vi "Thermal_Camera_Evaluation.vi"() -> (11 "placeholder image":T1(plugin-control))   [LabVIEW 2020]
uses:
  <vilib>/vision/Image Controls.llb/IMAQ Image.ctl
  DataCluster_TCAL.ctl
  <vilib>/Utility/file.llb/Write Delimited Spreadsheet (string).vi
  <vilib>/Utility/file.llb/Read Delimited Spreadsheet (string).vi
  <vilib>/Analysis/NI_AALBase.lvlib
panel:
  in  "Correct Data":bool
  out "Offset Applied?":bool=TRUE
  out "recentPaths":path[](array[path])=[path "C:/Users/au540322/Documents/Projects/Ice-Nucleation/Data/D20_4/Result Data.csv", path "C:/Users/au540322/Documents/Projects/Ice-Nucleation/Data/System Test_9/Result Data.csv"]
  out "version":string="version 0.0.0.1" caption="Version"
  out "Title":string="Thermal Camera Evaluation" caption="Version"
  in  "Remove_Correction":bool
  out "Offsets":dbl[](array[numeric])
  in  "Calc_All":bool
  in  "Well":i32=94
  in  "ImageIdx":u32(slide)=74 scale=0.0..527.0
  in  "Path":path=path "C:/Users/au540322/Documents/Projects/Ice-Nucleation/Data/D20_4"
  out "FreezeArray":bool[](array[boolean])=[TRUE, TRUE, TRUE, TRUE, TRUE, TRUE, TRUE, TRUE, TRUE, TRUE, TRUE, TRUE, TRUE, TRUE, TRUE, TRUE, TRUE, TRUE, FALSE, TRUE, TRUE, TRUE, TRUE, TRUE, TRUE, TRUE, TRUE, TRUE, TRUE, TRUE, TRUE, TRUE, TRUE, TRUE, TRUE, TRUE, TRUE, TRUE, TRUE, TRUE, TRUE, TRUE, FALSE, TRUE, TRUE, TRUE, TRUE, TRUE, TRUE, TRUE, TRUE, TRUE, TRUE, TRUE, TRUE, TRUE, TRUE, TRUE, TRUE, TRUE, TRUE, TRUE, TRUE, TRUE, TRUE, TRUE, FALSE, TRUE, TRUE, FALSE, TRUE, TRUE, TRUE, TRUE, TRUE, TRUE, TRUE, TRUE, TRUE, TRUE, TRUE, TRUE, TRUE, TRUE, TRUE, TRUE, TRUE, TRUE, TRUE, TRUE, TRUE, TRUE, TRUE, TRUE, TRUE, TRUE, TRUE, TRUE, TRUE, TRUE, TRUE, TRUE, TRUE, TRUE, TRUE, TRUE, TRUE, TRUE, TRUE, TRUE, TRUE, TRUE, TRUE, TRUE, TRUE, TRUE, TRUE, TRUE, TRUE, TRUE, TRUE, TRUE, TRUE, TRUE, TRUE, TRUE, TRUE, TRUE, TRUE, TRUE, TRUE, TRUE, TRUE, TRUE, TRUE, TRUE, TRUE, TRUE, TRUE, TRUE, TRUE, TRUE, TRUE, TRUE, TRUE, TRUE, TRUE, TRUE, TRUE, TRUE, TRUE, TRUE, TRUE, TRUE, TRUE, TRUE, TRUE, TRUE, TRUE, TRUE, TRUE, TRUE, TRUE, TRUE, TRUE, TRUE, TRUE, TRUE, TRUE, TRUE, TRUE, TRUE, TRUE, TRUE, TRUE, TRUE, TRUE, TRUE, TRUE, TRUE, TRUE, TRUE, TRUE, TRUE, TRUE, TRUE, TRUE, TRUE, TRUE, TRUE, TRUE, TRUE, TRUE, TRUE, TRUE, TRUE, TRUE, TRUE, TRUE, TRUE, TRUE, TRUE, TRUE, TRUE, TRUE, TRUE, TRUE, TRUE, TRUE, TRUE, FALSE, TRUE, TRUE, TRUE, TRUE, TRUE, TRUE, TRUE, TRUE, TRUE, TRUE, TRUE, TRUE, TRUE, TRUE, TRUE, TRUE, TRUE, TRUE, TRUE, TRUE, TRUE, TRUE, TRUE, FALSE, TRUE, TRUE, TRUE, TRUE, TRUE, TRUE, TRUE, TRUE, TRUE, TRUE, TRUE, TRUE, TRUE, TRUE, TRUE, TRUE, TRUE, TRUE, TRUE, TRUE, TRUE, TRUE, TRUE, FALSE, TRUE, TRUE, TRUE, TRUE, TRUE, TRUE, TRUE, TRUE, TRUE, TRUE, TRUE, TRUE, TRUE, TRUE, TRUE, TRUE, TRUE, TRUE, TRUE, TRUE, TRUE, TRUE, TRUE, TRUE, TRUE, TRUE, TRUE, TRUE, TRUE, TRUE, TRUE, TRUE, TRUE, TRUE, TRUE, TRUE, TRUE, TRUE, TRUE, TRUE, TRUE, TRUE, TRUE, TRUE, TRUE, TRUE, TRUE, TRUE, TRUE, TRUE, TRUE, TRUE, TRUE, TRUE, TRUE, TRUE, TRUE, TRUE, TRUE, TRUE, TRUE, TRUE, TRUE, TRUE, TRUE, TRUE, TRUE, TRUE, TRUE, TRUE, TRUE, TRUE, TRUE, TRUE, TRUE, TRUE, TRUE, TRUE, TRUE, TRUE, TRUE, TRUE, TRUE, TRUE, TRUE, TRUE, TRUE, TRUE, TRUE, TRUE, TRUE, TRUE, TRUE, TRUE, TRUE, TRUE, TRUE, TRUE, TRUE, TRUE, TRUE, TRUE, TRUE, TRUE, TRUE, TRUE, TRUE, TRUE, TRUE, TRUE, TRUE, TRUE, TRUE, TRUE, TRUE, TRUE, TRUE, TRUE, TRUE, TRUE, TRUE, TRUE, TRUE, TRUE, TRUE]
  out "ThermTemps":dbl[](array[numeric])=[7.37336, 7.350183, 7.292026, 7.209824, 7.126844, 7.047335, 6.967812, 6.887927, 6.807507, 6.726127, 6.647346, 6.566629, 6.484972, 6.403476, 6.320742, 6.240016, 6.159057, 6.077253, 5.994363, 5.911582, 5.834026, 5.750156, 5.668103, 5.585564, 5.503295, 5.421148, 5.337707, 5.255535, 5.176404, 5.097319, 5.014855, 4.933567, 4.8527, 4.772503, 4.690195, 4.609957, 4.530865, 4.450195, 4.368275, 4.287447, 4.20743, 4.128069, 4.046262, 3.966046, 3.884444, 3.804914, 3.72549, 3.644432, 3.56432, 3.482743, 3.402111, 3.320773, 3.241597, 3.160814, 3.078633, 2.999147, 2.916221, 2.834318, 2.753718, 2.671023, 2.590394, 2.507449, 2.425426, 2.345006, 2.263807, 2.180767, 2.098148, 2.01567, 1.933412, 1.852712, 1.770749, 1.688175, 1.60685, 1.526749, 1.447674, 1.3716, 1.297226, 1.221186, 1.146355, 1.070605, 0.992937, 0.915288, 0.838683, 0.762464, 0.679874, 0.600579, 0.51705, 0.434996, 0.356589, 0.277921, 0.196637, 0.111731, 0.026607, -0.060313, -0.14656, -0.233002, -0.318977, -0.403944, -0.487975, -0.568988, -0.651118, -0.726572, -0.802282, -0.877375, -0.955081, -1.032134, -1.111683, -1.190094, -1.270206, -1.349321, -1.429882, -1.51019, -1.594696, -1.675437, -1.76021, -1.842875, -1.926273, -2.011868, -2.097424, -2.180477, -2.265338, -2.350737, -2.434776, -2.520055, -2.603456, -2.685369, -2.767054, -2.849678, -2.928727, -3.007247, -3.085221, -3.160799, -3.237649, -3.314684, -3.391643, -3.468468, -3.546785, -3.624741, -3.70393, -3.783419, -3.864142, -3.943202, -4.022923, -4.103283, -4.185443, -4.267742, -4.351195, -4.432318, -4.516093, -4.599727, -4.682185, -4.766104, -4.850224, -4.93466, -5.017512, -5.101476, -5.183878, -5.266203, -5.3476, -5.430232, -5.512818, -5.595638, -5.678559, -5.759164, -5.842224, -5.925119, -6.00861, -6.087647, -6.169719, -6.250624, -6.332033, -6.41154, -6.493741, -6.574607, -6.65432, -6.735998, -6.81658, -6.884113, -6.971353, -7.058345, -7.13845, -7.217778, -7.29712, -7.376817, -7.457704, -7.536944, -7.618041, -7.696611, -7.776192, -7.856406, -7.936625, -8.015928, -8.096638, -8.176965, -8.256535, -8.333434, -8.412476, -8.491866, -8.572104, -8.653451, -8.736341, -8.818344, -8.9003, -8.979957, -9.063351, -9.144428, -9.225466, -9.308084, -9.389312, -9.471749, -9.55375, -9.635666, -9.719444, -9.801393, -9.883319, -9.965156, -10.046111, -10.126569, -10.206901, -10.288882, -10.367175, -10.44764, -10.528476, -10.607278, -10.686439, -10.76692, -10.846853, -10.925344, -11.005718, -11.085251, -11.164821, -11.243882, -11.32307, -11.402453, -11.482498, -11.561041, -11.641285, -11.721693, -11.802165, -11.881356, -11.960557, -12.038971, -12.117215, -12.198103, -12.277232, -12.357776, -12.438832, -12.518799, -12.601298, -12.682659, -12.764128, -12.845615, -12.926062, -13.007562, -13.090462, -13.172514, -13.253457, -13.335363, -13.415947, -13.500095, -13.581218, -13.662798, -13.745541, -13.827711, -13.909167, -13.988528, -14.067897, -14.146499, -14.22637, -14.306951, -14.385678, -14.465256, -14.545529, -14.624618, -14.703428, -14.780312, -14.860595, -14.938995, -15.018888, -15.099258, -15.177778, -15.257835, -15.336496, -15.415752, -15.494147, -15.573314, -15.652589, -15.731922, -15.809635, -15.888123, -15.96994, -16.049542, -16.129671, -16.210636, -16.291627, -16.372217, -16.453213, -16.533459, -16.614772, -16.697373, -16.777753, -16.859325, -16.941111, -17.021954, -17.104644, -17.18694, -17.265191, -17.34818, -17.429989, -17.511056, -17.592864, -17.672998, -17.752001, -17.832689, -17.912607, -17.991497, -18.072515, -18.152648, -18.231922, -18.310442, -18.39034, -18.469296, -18.547367, -18.625873, -18.703345, -18.784246, -18.861563, -18.939331, -19.016652, -19.094699, -19.172515, -19.250605, -19.329034, -19.40733, -19.486762, -19.565877, -19.648403, -19.726327, -19.808446, -19.888915, -19.969109, -20.049822, -20.129964, -20.210119, -20.290948, -20.37219, -20.454346, -20.533518, -20.615081, -20.69688, -20.779181, -20.859909, -20.940508, -21.021895, -21.10374, -21.185525, -21.268245, -21.348339, -21.425612, -21.505022, -21.583855, -21.662198, -21.739967, -21.818083, -21.894826, -21.972925, -22.050531, -22.127525, -22.204371, -22.282005, -22.35634, -22.434321, -22.511412, -22.589688, -22.667553, -22.744158, -22.822019, -22.89791, -22.975844, -23.05133, -23.130531, -23.211038, -23.290909, -23.370573, -23.45021, -23.530535, -23.609552, -23.687938, -23.768015, -23.847606, -23.927972, -24.010068, -24.089525, -24.16956, -24.249907, -24.330105, -24.40904, -24.488729, -24.569942, -24.649037, -24.729342, -24.80955, -24.888373, -24.967519, -25.047611, -25.125437, -25.204448, -25.282442, -25.360463, -25.437591, -25.514136, -25.593629, -25.668979, -25.743502, -25.820043, -25.89306, -25.97015, -26.045113, -26.118008, -26.194843, -26.268271, -26.342508, -26.416119, -26.490791, -26.566611, -26.642888, -26.719932, -26.797288, -26.874969, -26.951676, -27.028748, -27.104065, -27.181792, -27.258419, -27.33566, -27.413455, -27.493028, -27.56923, -27.646282, -27.721342, -27.798636, -27.878491, -27.956447, -28.033548, -28.109932, -28.186744, -28.262818, -28.340363, -28.41596, -28.491609, -28.56755, -28.642851, -28.720287, -28.794581, -28.868607, -28.943815, -29.019102, -29.093409, -29.168045, -29.242483, -29.315565, -29.390267, -29.463635, -29.540833, -29.613751, -29.686, -29.757983, -29.830992, -29.902322, -29.975634, -30.043051, -30.107764, -30.175561, -30.243789, -30.314343, -30.381896, -30.449693, -30.507812, -30.566745, -30.623567, -30.680952, -30.734143, -30.787765, -30.83898, -30.888996, -30.939253, -30.987606, -31.032869, -31.08053, -31.125474, -31.170159, -31.214239, -31.2553, -31.297168, -31.338367, -31.377898, -31.416899, -31.456416, -31.492706, -31.528817, -31.56739, -31.602582, -31.637368, -31.673019, -31.704931, -31.738656, -31.77053, -31.801731, -31.832112, -31.862399, -31.888523, -31.920833, -31.946986, -31.97368, -32.001595, -32.026341, -32.054092, -32.079652, -32.104587, -32.128267, -32.154891, -32.176728, -32.198059, -32.21954, -32.242051, -32.264665, -32.28386, -32.306436]
  out "PartitionArray":string[](array[string])=["A, MQ unfiltered", "A, MQ unfiltered", "A, MQ unfiltered", "B, D2O unfiltered", "B, D2O unfiltered", "B, D2O unfiltered", "C, 1mg/ml Snomax in MQ", "C, 1mg/ml Snomax in MQ", "C, 1mg/ml Snomax in MQ", "C, 1mg/ml Snomax in MQ", "C, 1mg/ml Snomax in MQ", "C, 1mg/ml Snomax in MQ", "D, 1mg/ml Snomax in 1:1 MQ:D2O", "D, 1mg/ml Snomax in 1:1 MQ:D2O", "D, 1mg/ml Snomax in 1:1 MQ:D2O", "D, 1mg/ml Snomax in 1:1 MQ:D2O", "D, 1mg/ml Snomax in 1:1 MQ:D2O", "D, 1mg/ml Snomax in 1:1 MQ:D2O", "E, 1mg/ml Snomax in D2O", "E, 1mg/ml Snomax in D2O", "E, 1mg/ml Snomax in D2O", "E, 1mg/ml Snomax in D2O", "E, 1mg/ml Snomax in D2O", "E, 1mg/ml Snomax in D2O", "A, MQ unfiltered", "A, MQ unfiltered", "A, MQ unfiltered", "B, D2O unfiltered", "B, D2O unfiltered", "B, D2O unfiltered", "C, 1mg/ml Snomax in MQ", "C, 1mg/ml Snomax in MQ", "C, 1mg/ml Snomax in MQ", "C, 1mg/ml Snomax in MQ", "C, 1mg/ml Snomax in MQ", "C, 1mg/ml Snomax in MQ", "D, 1mg/ml Snomax in 1:1 MQ:D2O", "D, 1mg/ml Snomax in 1:1 MQ:D2O", "D, 1mg/ml Snomax in 1:1 MQ:D2O", "D, 1mg/ml Snomax in 1:1 MQ:D2O", "D, 1mg/ml Snomax in 1:1 MQ:D2O", "D, 1mg/ml Snomax in 1:1 MQ:D2O", "E, 1mg/ml Snomax in D2O", "E, 1mg/ml Snomax in D2O", "E, 1mg/ml Snomax in D2O", "E, 1mg/ml Snomax in D2O", "E, 1mg/ml Snomax in D2O", "E, 1mg/ml Snomax in D2O", "A, MQ unfiltered", "A, MQ unfiltered", "A, MQ unfiltered", "B, D2O unfiltered", "B, D2O unfiltered", "B, D2O unfiltered", "C, 1mg/ml Snomax in MQ", "C, 1mg/ml Snomax in MQ", "C, 1mg/ml Snomax in MQ", "C, 1mg/ml Snomax in MQ", "C, 1mg/ml Snomax in MQ", "C, 1mg/ml Snomax in MQ", "D, 1mg/ml Snomax in 1:1 MQ:D2O", "D, 1mg/ml Snomax in 1:1 MQ:D2O", "D, 1mg/ml Snomax in 1:1 MQ:D2O", "D, 1mg/ml Snomax in 1:1 MQ:D2O", "D, 1mg/ml Snomax in 1:1 MQ:D2O", "D, 1mg/ml Snomax in 1:1 MQ:D2O", "E, 1mg/ml Snomax in D2O", "E, 1mg/ml Snomax in D2O", "E, 1mg/ml Snomax in D2O", "E, 1mg/ml Snomax in D2O", "E, 1mg/ml Snomax in D2O", "E, 1mg/ml Snomax in D2O", "A, MQ unfiltered", "A, MQ unfiltered", "A, MQ unfiltered", "B, D2O unfiltered", "B, D2O unfiltered", "B, D2O unfiltered", "C, 1mg/ml Snomax in MQ", "C, 1mg/ml Snomax in MQ", "C, 1mg/ml Snomax in MQ", "C, 1mg/ml Snomax in MQ", "C, 1mg/ml Snomax in MQ", "C, 1mg/ml Snomax in MQ", "D, 1mg/ml Snomax in 1:1 MQ:D2O", "D, 1mg/ml Snomax in 1:1 MQ:D2O", "D, 1mg/ml Snomax in 1:1 MQ:D2O", "D, 1mg/ml Snomax in 1:1 MQ:D2O", "D, 1mg/ml Snomax in 1:1 MQ:D2O", "D, 1mg/ml Snomax in 1:1 MQ:D2O", "E, 1mg/ml Snomax in D2O", "E, 1mg/ml Snomax in D2O", "E, 1mg/ml Snomax in D2O", "E, 1mg/ml Snomax in D2O", "E, 1mg/ml Snomax in D2O", "E, 1mg/ml Snomax in D2O", "A, MQ unfiltered", "A, MQ unfiltered", "A, MQ unfiltered", "B, D2O unfiltered", "B, D2O unfiltered", "B, D2O unfiltered", "C, 1mg/ml Snomax in MQ", "C, 1mg/ml Snomax in MQ", "C, 1mg/ml Snomax in MQ", "C, 1mg/ml Snomax in MQ", "C, 1mg/ml Snomax in MQ", "C, 1mg/ml Snomax in MQ", "D, 1mg/ml Snomax in 1:1 MQ:D2O", "D, 1mg/ml Snomax in 1:1 MQ:D2O", "D, 1mg/ml Snomax in 1:1 MQ:D2O", "D, 1mg/ml Snomax in 1:1 MQ:D2O", "D, 1mg/ml Snomax in 1:1 MQ:D2O", "D, 1mg/ml Snomax in 1:1 MQ:D2O", "E, 1mg/ml Snomax in D2O", "E, 1mg/ml Snomax in D2O", "E, 1mg/ml Snomax in D2O", "E, 1mg/ml Snomax in D2O", "E, 1mg/ml Snomax in D2O", "E, 1mg/ml Snomax in D2O", "A, MQ unfiltered", "A, MQ unfiltered", "A, MQ unfiltered", "B, D2O unfiltered", "B, D2O unfiltered", "B, D2O unfiltered", "C, 1mg/ml Snomax in MQ", "C, 1mg/ml Snomax in MQ", "C, 1mg/ml Snomax in MQ", "C, 1mg/ml Snomax in MQ", "C, 1mg/ml Snomax in MQ", "C, 1mg/ml Snomax in MQ", "D, 1mg/ml Snomax in 1:1 MQ:D2O", "D, 1mg/ml Snomax in 1:1 MQ:D2O", "D, 1mg/ml Snomax in 1:1 MQ:D2O", "D, 1mg/ml Snomax in 1:1 MQ:D2O", "D, 1mg/ml Snomax in 1:1 MQ:D2O", "D, 1mg/ml Snomax in 1:1 MQ:D2O", "E, 1mg/ml Snomax in D2O", "E, 1mg/ml Snomax in D2O", "E, 1mg/ml Snomax in D2O", "E, 1mg/ml Snomax in D2O", "E, 1mg/ml Snomax in D2O", "E, 1mg/ml Snomax in D2O", "A, MQ unfiltered", "A, MQ unfiltered", "A, MQ unfiltered", "B, D2O unfiltered", "B, D2O unfiltered", "B, D2O unfiltered", "C, 1mg/ml Snomax in MQ", "C, 1mg/ml Snomax in MQ", "C, 1mg/ml Snomax in MQ", "C, 1mg/ml Snomax in MQ", "C, 1mg/ml Snomax in MQ", "C, 1mg/ml Snomax in MQ", "D, 1mg/ml Snomax in 1:1 MQ:D2O", "D, 1mg/ml Snomax in 1:1 MQ:D2O", "D, 1mg/ml Snomax in 1:1 MQ:D2O", "D, 1mg/ml Snomax in 1:1 MQ:D2O", "D, 1mg/ml Snomax in 1:1 MQ:D2O", "D, 1mg/ml Snomax in 1:1 MQ:D2O", "E, 1mg/ml Snomax in D2O", "E, 1mg/ml Snomax in D2O", "E, 1mg/ml Snomax in D2O", "E, 1mg/ml Snomax in D2O", "E, 1mg/ml Snomax in D2O", "E, 1mg/ml Snomax in D2O", "A, MQ unfiltered", "A, MQ unfiltered", "A, MQ unfiltered", "B, D2O unfiltered", "B, D2O unfiltered", "B, D2O unfiltered", "C, 1mg/ml Snomax in MQ", "C, 1mg/ml Snomax in MQ", "C, 1mg/ml Snomax in MQ", "C, 1mg/ml Snomax in MQ", "C, 1mg/ml Snomax in MQ", "C, 1mg/ml Snomax in MQ", "D, 1mg/ml Snomax in 1:1 MQ:D2O", "D, 1mg/ml Snomax in 1:1 MQ:D2O", "D, 1mg/ml Snomax in 1:1 MQ:D2O", "D, 1mg/ml Snomax in 1:1 MQ:D2O", "D, 1mg/ml Snomax in 1:1 MQ:D2O", "D, 1mg/ml Snomax in 1:1 MQ:D2O", "E, 1mg/ml Snomax in D2O", "E, 1mg/ml Snomax in D2O", "E, 1mg/ml Snomax in D2O", "E, 1mg/ml Snomax in D2O", "E, 1mg/ml Snomax in D2O", "E, 1mg/ml Snomax in D2O", "A, MQ unfiltered", "A, MQ unfiltered", "A, MQ unfiltered", "B, D2O unfiltered", "B, D2O unfiltered", "B, D2O unfiltered", "C, 1mg/ml Snomax in MQ", "C, 1mg/ml Snomax in MQ", "C, 1mg/ml Snomax in MQ", "C, 1mg/ml Snomax in MQ", "C, 1mg/ml Snomax in MQ", "C, 1mg/ml Snomax in MQ", "D, 1mg/ml Snomax in 1:1 MQ:D2O", "D, 1mg/ml Snomax in 1:1 MQ:D2O", "D, 1mg/ml Snomax in 1:1 MQ:D2O", "D, 1mg/ml Snomax in 1:1 MQ:D2O", "D, 1mg/ml Snomax in 1:1 MQ:D2O", "D, 1mg/ml Snomax in 1:1 MQ:D2O", "E, 1mg/ml Snomax in D2O", "E, 1mg/ml Snomax in D2O", "E, 1mg/ml Snomax in D2O", "E, 1mg/ml Snomax in D2O", "E, 1mg/ml Snomax in D2O", "E, 1mg/ml Snomax in D2O", "A, MQ unfiltered", "A, MQ unfiltered", "A, MQ unfiltered", "B, D2O unfiltered", "B, D2O unfiltered", "B, D2O unfiltered", "C, 1mg/ml Snomax in MQ", "C, 1mg/ml Snomax in MQ", "C, 1mg/ml Snomax in MQ", "C, 1mg/ml Snomax in MQ", "C, 1mg/ml Snomax in MQ", "C, 1mg/ml Snomax in MQ", "D, 1mg/ml Snomax in 1:1 MQ:D2O", "D, 1mg/ml Snomax in 1:1 MQ:D2O", "D, 1mg/ml Snomax in 1:1 MQ:D2O", "D, 1mg/ml Snomax in 1:1 MQ:D2O", "D, 1mg/ml Snomax in 1:1 MQ:D2O", "D, 1mg/ml Snomax in 1:1 MQ:D2O", "E, 1mg/ml Snomax in D2O", "E, 1mg/ml Snomax in D2O", "E, 1mg/ml Snomax in D2O", "E, 1mg/ml Snomax in D2O", "E, 1mg/ml Snomax in D2O", "E, 1mg/ml Snomax in D2O", "A, MQ unfiltered", "A, MQ unfiltered", "A, MQ unfiltered", "B, D2O unfiltered", "B, D2O unfiltered", "B, D2O unfiltered", "C, 1mg/ml Snomax in MQ", "C, 1mg/ml Snomax in MQ", "C, 1mg/ml Snomax in MQ", "C, 1mg/ml Snomax in MQ", "C, 1mg/ml Snomax in MQ", "C, 1mg/ml Snomax in MQ", "D, 1mg/ml Snomax in 1:1 MQ:D2O", "D, 1mg/ml Snomax in 1:1 MQ:D2O", "D, 1mg/ml Snomax in 1:1 MQ:D2O", "D, 1mg/ml Snomax in 1:1 MQ:D2O", "D, 1mg/ml Snomax in 1:1 MQ:D2O", "D, 1mg/ml Snomax in 1:1 MQ:D2O", "E, 1mg/ml Snomax in D2O", "E, 1mg/ml Snomax in D2O", "E, 1mg/ml Snomax in D2O", "E, 1mg/ml Snomax in D2O", "E, 1mg/ml Snomax in D2O", "E, 1mg/ml Snomax in D2O", "A, MQ unfiltered", "A, MQ unfiltered", "A, MQ unfiltered", "B, D2O unfiltered", "B, D2O unfiltered", "B, D2O unfiltered", "C, 1mg/ml Snomax in MQ", "C, 1mg/ml Snomax in MQ", "C, 1mg/ml Snomax in MQ", "C, 1mg/ml Snomax in MQ", "C, 1mg/ml Snomax in MQ", "C, 1mg/ml Snomax in MQ", "D, 1mg/ml Snomax in 1:1 MQ:D2O", "D, 1mg/ml Snomax in 1:1 MQ:D2O", "D, 1mg/ml Snomax in 1:1 MQ:D2O", "D, 1mg/ml Snomax in 1:1 MQ:D2O", "D, 1mg/ml Snomax in 1:1 MQ:D2O", "D, 1mg/ml Snomax in 1:1 MQ:D2O", "E, 1mg/ml Snomax in D2O", "E, 1mg/ml Snomax in D2O", "E, 1mg/ml Snomax in D2O", "E, 1mg/ml Snomax in D2O", "E, 1mg/ml Snomax in D2O", "E, 1mg/ml Snomax in D2O", "A, MQ unfiltered", "A, MQ unfiltered", "A, MQ unfiltered", "B, D2O unfiltered", "B, D2O unfiltered", "B, D2O unfiltered", "C, 1mg/ml Snomax in MQ", "C, 1mg/ml Snomax in MQ", "C, 1mg/ml Snomax in MQ", "C, 1mg/ml Snomax in MQ", "C, 1mg/ml Snomax in MQ", "C, 1mg/ml Snomax in MQ", "D, 1mg/ml Snomax in 1:1 MQ:D2O", "D, 1mg/ml Snomax in 1:1 MQ:D2O", "D, 1mg/ml Snomax in 1:1 MQ:D2O", "D, 1mg/ml Snomax in 1:1 MQ:D2O", "D, 1mg/ml Snomax in 1:1 MQ:D2O", "D, 1mg/ml Snomax in 1:1 MQ:D2O", "E, 1mg/ml Snomax in D2O", "E, 1mg/ml Snomax in D2O", "E, 1mg/ml Snomax in D2O", "E, 1mg/ml Snomax in D2O", "E, 1mg/ml Snomax in D2O", "E, 1mg/ml Snomax in D2O", "A, MQ unfiltered", "A, MQ unfiltered", "A, MQ unfiltered", "B, D2O unfiltered", "B, D2O unfiltered", "B, D2O unfiltered", "C, 1mg/ml Snomax in MQ", "C, 1mg/ml Snomax in MQ", "C, 1mg/ml Snomax in MQ", "C, 1mg/ml Snomax in MQ", "C, 1mg/ml Snomax in MQ", "C, 1mg/ml Snomax in MQ", "D, 1mg/ml Snomax in 1:1 MQ:D2O", "D, 1mg/ml Snomax in 1:1 MQ:D2O", "D, 1mg/ml Snomax in 1:1 MQ:D2O", "D, 1mg/ml Snomax in 1:1 MQ:D2O", "D, 1mg/ml Snomax in 1:1 MQ:D2O", "D, 1mg/ml Snomax in 1:1 MQ:D2O", "E, 1mg/ml Snomax in D2O", "E, 1mg/ml Snomax in D2O", "E, 1mg/ml Snomax in D2O", "E, 1mg/ml Snomax in D2O", "E, 1mg/ml Snomax in D2O", "E, 1mg/ml Snomax in D2O", "A, MQ unfiltered", "A, MQ unfiltered", "A, MQ unfiltered", "B, D2O unfiltered", "B, D2O unfiltered", "B, D2O unfiltered", "C, 1mg/ml Snomax in MQ", "C, 1mg/ml Snomax in MQ", "C, 1mg/ml Snomax in MQ", "C, 1mg/ml Snomax in MQ", "C, 1mg/ml Snomax in MQ", "C, 1mg/ml Snomax in MQ", "D, 1mg/ml Snomax in 1:1 MQ:D2O", "D, 1mg/ml Snomax in 1:1 MQ:D2O", "D, 1mg/ml Snomax in 1:1 MQ:D2O", "D, 1mg/ml Snomax in 1:1 MQ:D2O", "D, 1mg/ml Snomax in 1:1 MQ:D2O", "D, 1mg/ml Snomax in 1:1 MQ:D2O", "E, 1mg/ml Snomax in D2O", "E, 1mg/ml Snomax in D2O", "E, 1mg/ml Snomax in D2O", "E, 1mg/ml Snomax in D2O", "E, 1mg/ml Snomax in D2O", "E, 1mg/ml Snomax in D2O", "A, MQ unfiltered", "A, MQ unfiltered", "A, MQ unfiltered", "B, D2O unfiltered", "B, D2O unfiltered", "B, D2O unfiltered", "C, 1mg/ml Snomax in MQ", "C, 1mg/ml Snomax in MQ", "C, 1mg/ml Snomax in MQ", "C, 1mg/ml Snomax in MQ", "C, 1mg/ml Snomax in MQ", "C, 1mg/ml Snomax in MQ", "D, 1mg/ml Snomax in 1:1 MQ:D2O", "D, 1mg/ml Snomax in 1:1 MQ:D2O", "D, 1mg/ml Snomax in 1:1 MQ:D2O", "D, 1mg/ml Snomax in 1:1 MQ:D2O", "D, 1mg/ml Snomax in 1:1 MQ:D2O", "D, 1mg/ml Snomax in 1:1 MQ:D2O", "E, 1mg/ml Snomax in D2O", "E, 1mg/ml Snomax in D2O", "E, 1mg/ml Snomax in D2O", "E, 1mg/ml Snomax in D2O", "E, 1mg/ml Snomax in D2O", "E, 1mg/ml Snomax in D2O"]
  out "FreezeTemps":dbl[](array[numeric])=[-17.28714285714284, -23.360476190476163, -18.044761904761884, -18.98333333333329, -13.286190476190427, -20.920476190476165, -5.292380952380938, -5.350476190476172, -5.453809523809525, -5.195714285714246, -5.249047619047587, -5.483333333333292, -2.8057142857142594, -2.902380952380952, -2.915714285714273, -2.8785714285713766, -2.9642857142857224, -3.019999999999982, 0.0, -1.2985714285713925, -0.7119047619047478, -0.5214285714285438, -0.0428571428570876, -0.5152380952380895, -16.166190476190422, -14.609999999999957, -25.292857142857116, -20.543333333333294, -22.113333333333287, -21.32571428571424, -5.505238095238042, -5.593809523809512, -5.405714285714225, -5.401428571428539, -5.500952380952356, -5.363333333333287, -3.08095238095234, -3.0838095238095207, -3.0514285714285734, -3.015714285714239, -2.96333333333331, -3.152380952380952, 0.0, -0.61761904761903, -0.7347619047618537, -0.5952380952380736, -0.6928571428571217, -0.4047619047618696, -19.03666666666666, -14.313333333333276, -15.039047619047608, -14.185238095238049, -20.61285714285711, -21.26190476190473, -5.579523809523778, -5.624285714285691, -5.4423809523809155, -5.434761904761899, -5.471904761904739, -5.935238095238049, -3.0038095238095366, -2.935714285714255, -2.964761904761872, -3.1223809523809223, -3.133333333333269, -2.9828571428570854, 0.0, -1.0409523809523193, -0.8623809523809314, 0.0, -0.1014285714285847, -0.7966666666666242, -15.671428571428578, -11.62428571428569, -15.217142857142846, -14.780476190476179, -20.487619047619006, -16.03047619047618, -5.399523809523771, -5.3642857142857, -5.5033333333332735, -5.954285714285675, -5.610476190476163, -5.480476190476168, -3.2566666666666606, -3.0785714285713652, -2.83428571428567, -3.031904761904741, -3.0571428571428214, -3.1619047619047365, -0.6461904761904407, -1.014285714285677, -0.8404761904761813, -0.9290476190475943, -0.8390476190476193, -0.8742857142856906, -25.16952380952378, -17.619999999999976, -22.054285714285697, -14.887142857142862, -19.3942857142857, -20.490952380952336, -5.6619047619047365, -5.628571428571377, -5.825714285714241, -5.541904761904732, -5.704761904761881, -5.809523809523796, -3.402380952380952, -3.1676190476190413, -3.2052380952380872, -3.1780952380951817, -3.08428571428567, -3.1638095238095048, -1.1566666666666379, -0.8852380952380372, -0.9509523809523444, -0.784761904761865, -0.6295238095237892, -0.5247619047618741, -20.52047619047616, -22.020952380952338, -18.561428571428564, -21.041904761904732, -20.22999999999996, -19.46857142857138, -5.632380952380913, -5.829047619047628, -5.757619047619016, -5.409999999999968, -5.2971428571428305, -5.7942857142857065, -3.439047619047585, -3.210476190476129, -3.2157142857142276, -3.1152380952380554, -3.0599999999999454, -2.903809523809514, -0.9961904761904066, -1.029047619047617, -0.9152380952380668, -0.8190476190475806, -0.4390476190475852, -0.7114285714285415, -21.997619047619025, -23.774285714285696, -20.46666666666664, -19.79761904761901, -16.629999999999995, -19.37476190476187, -5.673809523809496, -5.544761904761856, -5.559523809523796, -5.588571428571413, -5.5719047619047615, -5.441904761904766, -3.299047619047599, -3.1723809523809336, -3.216190476190434, -3.300476190476161, -2.9395238095237914, -3.2376190476190345, -1.2780952380952044, -0.9566666666666492, -1.0123809523809086, -0.4071428571428441, -0.1261904761904589, -0.6047619047618582, -23.76714285714283, -20.47142857142856, -20.978095238095193, -16.091904761904743, -22.034285714285687, -16.039999999999964, -5.609047619047601, -5.653333333333308, -5.613333333333287, -5.550476190476161, -5.621904761904716, -5.621904761904716, -3.3133333333332757, -3.3828571428571195, -3.167142857142835, -3.2052380952380872, -3.2128571428571036, -3.1499999999999773, -1.1733333333332894, -1.3190476190475806, -0.8604761904761631, -1.011428571428553, -0.9661904761904339, -0.8266666666666538, -16.467142857142846, -22.642380952380933, -21.78380952380951, -20.803333333333285, -18.689047619047614, -5.77571428571423, -5.7071428571428555, -5.840952380952331, -5.715238095238078, -5.647619047619003, -5.512380952380909, -5.458095238095211, -3.29047619047617, -3.388095238095218, -3.332857142857108, -3.2142857142857224, -3.185714285714255, -3.296190476190418, 0.0, -1.360476190476163, -0.9638095238095161, -0.7519047619047683, -0.8533333333332962, -0.7152380952380781, -13.07714285714286, -22.502857142857096, -14.274285714285725, -21.791904761904732, -18.57238095238094, -14.203809523809525, -5.652380952380952, -5.71666666666664, -5.596666666666636, -5.579047619047628, -5.486666666666679, -5.535714285714221, -3.5138095238095275, -3.322857142857117, -3.3861904761904498, -3.308095238095177, -3.056666666666672, -3.133333333333269, 0.0, -1.0552380952380531, -0.9566666666666492, -0.8438095238095116, -0.5733333333332666, -0.8880952380952181, -11.63952380952378, -16.895714285714234, -23.103333333333296, -14.486666666666679, -6.6823809523809246, -19.833333333333286, -5.862857142857138, -5.714761904761872, -5.702857142857113, -5.740952380952365, -5.64285714285711, -5.604285714285709, -3.1357142857142435, -3.3133333333332757, -3.1299999999999955, -3.1995238095237823, -3.238095238095184, -3.1633333333332985, 0.0, -0.9942857142856951, -0.9276190476190322, -0.8047619047619037, -0.8871428571428623, -0.9176190476190413, -22.81761904761902, -17.840476190476153, -11.563809523809539, -8.832857142857108, -7.065238095238044, -17.505714285714248, -5.720952380952326, -5.677619047619032, -5.690476190476147, -5.643809523809523, -5.464761904761872, -5.563333333333276, -3.345714285714223, -3.254285714285686, -2.8928571428571104, -3.0804761904761335, -2.969523809523764, -3.0995238095238165, -1.1228571428571286, -0.9161904761904225, -0.6747619047619082, -0.781904761904741, -0.8728571428571286, -0.6352380952380372, -23.009999999999962, -17.229523809523783, -9.71999999999997, -5.177142857142826, -22.008095238095194, -5.899999999999977, -5.7390476190475965, -5.714285714285722, -5.618095238095179, -5.594761904761867, -5.941904761904766, -5.534285714285716, -3.293333333333294, -3.2347619047618537, -2.966190476190434, -3.1838095238094866, -2.9609523809523353, -3.0385714285714016, -1.167142857142835, -1.0023809523809177, -0.9547619047618809, -0.9495238095237823, -0.8280952380952158, -0.8585714285713948, -15.54095238095232, -11.46999999999997, -10.558095238095177, -22.105714285714242, -9.649523809523771, -8.017142857142858, -5.544761904761856, -5.662380952380943, -5.586190476190438, -5.632380952380913, -5.582380952380902, -5.65476190476187, -3.2333333333332916, -3.0485714285713925, -3.2085714285713607, -3.1385714285713675, -3.2114285714285415, -3.283333333333303, -0.5752380952380918, -0.8571428571428328, -0.7447619047619014, -0.6280952380952272, -0.8199999999999932, -0.6380952380952181, -18.772857142857106, -16.079523809523778, -10.479523809523812, -21.853333333333296, -16.9080952380952, -20.799523809523777, -5.465714285714228, -5.371904761904716, -5.692857142857122, -5.553809523809491, -5.554761904761904, -5.547619047619037, -2.9614285714285415, -2.967619047618996, -3.189047619047585, -3.2057142857142367, -2.995238095238051, -3.0338095238095093, -1.1819047619047183, -0.7414285714285711, -0.8514285714285847, -0.6380952380952181, -0.6257142857142526, -0.5314285714285347, -15.450476190476138, -17.551428571428545, -14.244285714285695, -5.428095238095182, -13.503809523809537, -11.372380952380922, -5.407142857142844, -5.306190476190409, -5.479999999999961, -5.233333333333292, -5.076666666666654, -5.421428571428578, -2.956190476190443, -2.809523809523796, -2.8680952380951794, -2.8466666666666356, -2.704761904761881, -2.7071428571428555, -0.3071428571428214, -0.5847619047618764, -0.5171428571428578, -0.3957142857142344, -0.4861904761904157, -0.4599999999999795]
  out "FreezeIdx":i32[](array[numeric])=[255, 322, 264, 271, 213, 293, 124, 126, 128, 125, 124, 129, 98, 99, 102, 99, 98, 98, 0, 81, 76, 73, 80, 73, 242, 225, 335, 285, 302, 293, 131, 126, 127, 130, 129, 126, 100, 105, 106, 99, 98, 99, 0, 73, 75, 79, 77, 71, 272, 219, 231, 224, 285, 293, 130, 135, 124, 133, 126, 135, 98, 99, 108, 99, 99, 98, 0, 76, 75, 0, 77, 76, 236, 192, 232, 228, 284, 240, 125, 125, 126, 137, 128, 126, 105, 106, 96, 110, 99, 100, 71, 80, 77, 79, 74, 77, 335, 254, 302, 233, 271, 287, 128, 133, 136, 127, 128, 133, 99, 107, 100, 108, 101, 101, 80, 77, 76, 74, 73, 74, 287, 301, 265, 290, 280, 272, 128, 136, 130, 124, 123, 130, 102, 99, 108, 100, 107, 100, 76, 76, 82, 75, 73, 74, 303, 321, 285, 279, 243, 273, 126, 126, 125, 126, 132, 124, 98, 108, 104, 111, 99, 106, 84, 76, 75, 82, 89, 72, 320, 283, 291, 240, 297, 236, 129, 131, 129, 124, 131, 126, 100, 105, 99, 100, 99, 101, 81, 81, 75, 76, 77, 75, 243, 307, 301, 286, 267, 129, 124, 132, 125, 127, 125, 124, 97, 104, 100, 99, 100, 100, 0, 88, 76, 73, 75, 75, 209, 309, 219, 296, 262, 217, 127, 131, 134, 127, 127, 124, 104, 100, 108, 107, 98, 99, 0, 77, 83, 80, 71, 76, 191, 248, 312, 218, 143, 278, 126, 126, 131, 133, 125, 126, 97, 100, 98, 99, 104, 100, 0, 78, 81, 75, 76, 75, 311, 257, 192, 162, 147, 252, 126, 126, 126, 130, 124, 123, 98, 98, 97, 98, 98, 99, 74, 79, 72, 73, 74, 73, 316, 253, 172, 122, 302, 135, 129, 129, 130, 124, 136, 125, 99, 103, 97, 101, 98, 98, 77, 74, 74, 82, 74, 77, 234, 193, 182, 305, 170, 153, 126, 132, 125, 133, 126, 125, 99, 98, 99, 99, 99, 102, 72, 74, 73, 73, 74, 73, 271, 240, 181, 300, 248, 288, 124, 125, 133, 132, 129, 124, 97, 97, 98, 99, 99, 99, 78, 81, 74, 75, 75, 73, 238, 259, 221, 128, 214, 192, 128, 128, 128, 124, 126, 129, 99, 99, 98, 99, 98, 98, 75, 78, 74, 79, 73, 75]
  out "maxSize":i32=527
  out "img":i32
  out "Slide":u8(slide) scale=0.0..100.0
  in  "Help":bool
  out "Tutorial":string="Click on a Well to show single or click outside the plate to show all."
  out "Points":T2[](array[typedef])=[{"X"=62.0, "Y"=66.0}, {"X"=77.521736, "Y"=65.73913}, {"X"=93.04348, "Y"=65.478264}, {"X"=108.565216, "Y"=65.21739}, {"X"=124.08696, "Y"=64.95652}, {"X"=139.6087, "Y"=64.695656}, {"X"=155.13043, "Y"=64.434784}, {"X"=170.65218, "Y"=64.17391}, {"X"=186.17392, "Y"=63.913044}, {"X"=201.69565, "Y"=63.652176}, {"X"=217.21739, "Y"=63.391304}, {"X"=232.73914, "Y"=63.130436}, {"X"=248.26086, "Y"=62.869564}, {"X"=263.7826, "Y"=62.608696}, {"X"=279.30435, "Y"=62.347824}, {"X"=294.82608, "Y"=62.086956}, {"X"=310.34784, "Y"=61.826088}, {"X"=325.86957, "Y"=61.565216}, {"X"=341.3913, "Y"=61.304348}, {"X"=356.91306, "Y"=61.04348}, {"X"=372.43478, "Y"=60.782608}, {"X"=387.9565, "Y"=60.52174}, {"X"=403.47827, "Y"=60.260868}, {"X"=419.0, "Y"=60.0}, {"X"=62.333332, "Y"=81.53333}, {"X"=77.85507, "Y"=81.27246}, {"X"=93.37681, "Y"=81.0116}, {"X"=108.89855, "Y"=80.750725}, {"X"=124.42029, "Y"=80.48985}, {"X"=139.94203, "Y"=80.22899}, {"X"=155.46376, "Y"=79.96812}, {"X"=170.9855, "Y"=79.707245}, {"X"=186.50725, "Y"=79.44638}, {"X"=202.02898, "Y"=79.18551}, {"X"=217.55072, "Y"=78.92464}, {"X"=233.07246, "Y"=78.66377}, {"X"=248.5942, "Y"=78.4029}, {"X"=264.11594, "Y"=78.14203}, {"X"=279.6377, "Y"=77.88116}, {"X"=295.15942, "Y"=77.62029}, {"X"=310.68115, "Y"=77.35942}, {"X"=326.2029, "Y"=77.09855}, {"X"=341.72464, "Y"=76.837685}, {"X"=357.2464, "Y"=76.57681}, {"X"=372.76813, "Y"=76.31594}, {"X"=388.28986, "Y"=76.05507}, {"X"=403.8116, "Y"=75.794205}, {"X"=419.33334, "Y"=75.53333}, {"X"=62.666668, "Y"=97.066666}, {"X"=78.18841, "Y"=96.8058}, {"X"=93.710144, "Y"=96.54493}, {"X"=109.23188, "Y"=96.28406}, {"X"=124.753624, "Y"=96.02319}, {"X"=140.27536, "Y"=95.76232}, {"X"=155.7971, "Y"=95.50145}, {"X"=171.31885, "Y"=95.240585}, {"X"=186.84058, "Y"=94.97971}, {"X"=202.36232, "Y"=94.71884}, {"X"=217.88406, "Y"=94.45797}, {"X"=233.4058, "Y"=94.1971}, {"X"=248.92754, "Y"=93.93623}, {"X"=264.44928, "Y"=93.67536}, {"X"=279.971, "Y"=93.41449}, {"X"=295.49274, "Y"=93.153625}, {"X"=311.0145, "Y"=92.89275}, {"X"=326.53622, "Y"=92.63188}, {"X"=342.05795, "Y"=92.37102}, {"X"=357.5797, "Y"=92.110146}, {"X"=373.10144, "Y"=91.84927}, {"X"=388.62317, "Y"=91.58841}, {"X"=404.14493, "Y"=91.32754}, {"X"=419.66666, "Y"=91.066666}, {"X"=63.0, "Y"=112.600006}, {"X"=78.521736, "Y"=112.339134}, {"X"=94.04348, "Y"=112.07826}, {"X"=109.565216, "Y"=111.8174}, {"X"=125.08696, "Y"=111.55652}, {"X"=140.6087, "Y"=111.295654}, {"X"=156.13043, "Y"=111.03479}, {"X"=171.65218, "Y"=110.77391}, {"X"=187.17392, "Y"=110.51305}, {"X"=202.69565, "Y"=110.252174}, {"X"=218.21739, "Y"=109.9913}, {"X"=233.73914, "Y"=109.73044}, {"X"=249.26086, "Y"=109.46957}, {"X"=264.78262, "Y"=109.208694}, {"X"=280.30435, "Y"=108.94783}, {"X"=295.82608, "Y"=108.68696}, {"X"=311.34784, "Y"=108.42609}, {"X"=326.86957, "Y"=108.16522}, {"X"=342.3913, "Y"=107.90435}, {"X"=357.91306, "Y"=107.64348}, {"X"=373.43478, "Y"=107.382614}, {"X"=388.9565, "Y"=107.12174}, {"X"=404.47827, "Y"=106.86087}, {"X"=420.0, "Y"=106.600006}, {"X"=63.333332, "Y"=128.13333}, {"X"=78.85507, "Y"=127.87247}, {"X"=94.37681, "Y"=127.611595}, {"X"=109.89855, "Y"=127.35072}, {"X"=125.42029, "Y"=127.08986}, {"X"=140.94203, "Y"=126.82899}, {"X"=156.46376, "Y"=126.568115}, {"X"=171.9855, "Y"=126.30725}, {"X"=187.50725, "Y"=126.04638}, {"X"=203.02898, "Y"=125.78551}, {"X"=218.55072, "Y"=125.52464}, {"X"=234.07246, "Y"=125.26377}, {"X"=249.5942, "Y"=125.0029}, {"X"=265.11594, "Y"=124.742035}, {"X"=280.6377, "Y"=124.48116}, {"X"=296.15942, "Y"=124.22029}, {"X"=311.68115, "Y"=123.95943}, {"X"=327.2029, "Y"=123.69855}, {"X"=342.72464, "Y"=123.43768}, {"X"=358.2464, "Y"=123.17682}, {"X"=373.76813, "Y"=122.91594}, {"X"=389.28986, "Y"=122.655075}, {"X"=404.8116, "Y"=122.3942}, {"X"=420.33334, "Y"=122.13333}, {"X"=63.666668, "Y"=143.66667}, {"X"=79.18841, "Y"=143.40579}, {"X"=94.710144, "Y"=143.14493}, {"X"=110.23188, "Y"=142.88406}, {"X"=125.753624, "Y"=142.6232}, {"X"=141.27536, "Y"=142.36234}, {"X"=156.7971, "Y"=142.10146}, {"X"=172.31885, "Y"=141.84058}, {"X"=187.84058, "Y"=141.57971}, {"X"=203.36232, "Y"=141.31885}, {"X"=218.88406, "Y"=141.05798}, {"X"=234.4058, "Y"=140.7971}, {"X"=249.92754, "Y"=140.53624}, {"X"=265.44928, "Y"=140.27536}, {"X"=280.971, "Y"=140.0145}, {"X"=296.49274, "Y"=139.75363}, {"X"=312.0145, "Y"=139.49277}, {"X"=327.53622, "Y"=139.23189}, {"X"=343.05795, "Y"=138.97102}, {"X"=358.5797, "Y"=138.71014}, {"X"=374.10144, "Y"=138.44928}, {"X"=389.62317, "Y"=138.18842}, {"X"=405.14493, "Y"=137.92755}, {"X"=420.66666, "Y"=137.66667}, {"X"=64.0, "Y"=159.20001}, {"X"=79.521736, "Y"=158.93913}, {"X"=95.04348, "Y"=158.67827}, {"X"=110.565216, "Y"=158.41739}, {"X"=126.08696, "Y"=158.15652}, {"X"=141.6087, "Y"=157.89566}, {"X"=157.13043, "Y"=157.6348}, {"X"=172.65218, "Y"=157.37392}, {"X"=188.17392, "Y"=157.11304}, {"X"=203.69565, "Y"=156.85217}, {"X"=219.21739, "Y"=156.59131}, {"X"=234.73914, "Y"=156.33044}, {"X"=250.26086, "Y"=156.06958}, {"X"=265.78262, "Y"=155.8087}, {"X"=281.30435, "Y"=155.54782}, {"X"=296.82608, "Y"=155.28696}, {"X"=312.34784, "Y"=155.0261}, {"X"=327.86957, "Y"=154.76523}, {"X"=343.3913, "Y"=154.50435}, {"X"=358.91306, "Y"=154.24348}, {"X"=374.43478, "Y"=153.9826}, {"X"=389.9565, "Y"=153.72174}, {"X"=405.47827, "Y"=153.46088}, {"X"=421.0, "Y"=153.20001}, {"X"=64.333336, "Y"=174.73334}, {"X"=79.85507, "Y"=174.47247}, {"X"=95.37681, "Y"=174.21161}, {"X"=110.89855, "Y"=173.95073}, {"X"=126.42029, "Y"=173.68985}, {"X"=141.94203, "Y"=173.42899}, {"X"=157.46376, "Y"=173.16812}, {"X"=172.9855, "Y"=172.90726}, {"X"=188.50725, "Y"=172.64638}, {"X"=204.02898, "Y"=172.38551}, {"X"=219.55072, "Y"=172.12463}, {"X"=235.07246, "Y"=171.86377}, {"X"=250.5942, "Y"=171.6029}, {"X"=266.11594, "Y"=171.34204}, {"X"=281.6377, "Y"=171.08116}, {"X"=297.15942, "Y"=170.8203}, {"X"=312.68115, "Y"=170.55942}, {"X"=328.2029, "Y"=170.29855}, {"X"=343.72464, "Y"=170.03769}, {"X"=359.2464, "Y"=169.77682}, {"X"=374.76813, "Y"=169.51595}, {"X"=390.28986, "Y"=169.25507}, {"X"=405.8116, "Y"=168.9942}, {"X"=421.33334, "Y"=168.73334}, {"X"=64.666664, "Y"=190.26666}, {"X"=80.18841, "Y"=190.0058}, {"X"=95.710144, "Y"=189.74493}, {"X"=111.23188, "Y"=189.48407}, {"X"=126.753624, "Y"=189.22319}, {"X"=142.27536, "Y"=188.96233}, {"X"=157.7971, "Y"=188.70145}, {"X"=173.31885, "Y"=188.44058}, {"X"=188.84058, "Y"=188.17972}, {"X"=204.36232, "Y"=187.91885}, {"X"=219.88406, "Y"=187.65797}, {"X"=235.4058, "Y"=187.3971}, {"X"=250.92754, "Y"=187.13623}, {"X"=266.44928, "Y"=186.87537}, {"X"=281.971, "Y"=186.6145}, {"X"=297.49274, "Y"=186.35364}, {"X"=313.0145, "Y"=186.09276}, {"X"=328.53622, "Y"=185.83188}, {"X"=344.05795, "Y"=185.57101}, {"X"=359.5797, "Y"=185.31015}, {"X"=375.10144, "Y"=185.04929}, {"X"=390.62317, "Y"=184.7884}, {"X"=406.14493, "Y"=184.52754}, {"X"=421.66666, "Y"=184.26666}, {"X"=65.0, "Y"=205.8}, {"X"=80.521736, "Y"=205.53914}, {"X"=96.04348, "Y"=205.27826}, {"X"=111.565216, "Y"=205.0174}, {"X"=127.08696, "Y"=204.75653}, {"X"=142.6087, "Y"=204.49565}, {"X"=158.13043, "Y"=204.23479}, {"X"=173.65218, "Y"=203.97392}, {"X"=189.17392, "Y"=203.71304}, {"X"=204.69565, "Y"=203.45218}, {"X"=220.21739, "Y"=203.19131}, {"X"=235.73914, "Y"=202.93044}, {"X"=251.26086, "Y"=202.66957}, {"X"=266.78262, "Y"=202.40869}, {"X"=282.30435, "Y"=202.14783}, {"X"=297.82608, "Y"=201.88696}, {"X"=313.34784, "Y"=201.62608}, {"X"=328.86957, "Y"=201.36522}, {"X"=344.3913, "Y"=201.10435}, {"X"=359.91306, "Y"=200.84348}, {"X"=375.43478, "Y"=200.58261}, {"X"=390.9565, "Y"=200.32175}, {"X"=406.47827, "Y"=200.06087}, {"X"=422.0, "Y"=199.8}, {"X"=65.333336, "Y"=221.33334}, {"X"=80.85507, "Y"=221.07248}, {"X"=96.37681, "Y"=220.8116}, {"X"=111.89855, "Y"=220.55074}, {"X"=127.42029, "Y"=220.28987}, {"X"=142.94203, "Y"=220.02899}, {"X"=158.46376, "Y"=219.76813}, {"X"=173.9855, "Y"=219.50726}, {"X"=189.50725, "Y"=219.24638}, {"X"=205.02898, "Y"=218.98552}, {"X"=220.55072, "Y"=218.72466}, {"X"=236.07246, "Y"=218.46378}, {"X"=251.5942, "Y"=218.20291}, {"X"=267.11594, "Y"=217.94203}, {"X"=282.6377, "Y"=217.68117}, {"X"=298.15942, "Y"=217.4203}, {"X"=313.68115, "Y"=217.15942}, {"X"=329.2029, "Y"=216.89856}, {"X"=344.72464, "Y"=216.6377}, {"X"=360.2464, "Y"=216.37682}, {"X"=375.76813, "Y"=216.11595}, {"X"=391.28986, "Y"=215.85509}, {"X"=406.8116, "Y"=215.59421}, {"X"=422.33334, "Y"=215.33334}, {"X"=65.666664, "Y"=236.86667}, {"X"=81.18841, "Y"=236.6058}, {"X"=96.710144, "Y"=236.34492}, {"X"=112.23188, "Y"=236.08406}, {"X"=127.753624, "Y"=235.8232}, {"X"=143.27536, "Y"=235.56232}, {"X"=158.7971, "Y"=235.30145}, {"X"=174.31885, "Y"=235.04059}, {"X"=189.84058, "Y"=234.77971}, {"X"=205.36232, "Y"=234.51884}, {"X"=220.88406, "Y"=234.25798}, {"X"=236.4058, "Y"=233.9971}, {"X"=251.92754, "Y"=233.73624}, {"X"=267.44928, "Y"=233.47536}, {"X"=282.971, "Y"=233.2145}, {"X"=298.49274, "Y"=232.95363}, {"X"=314.0145, "Y"=232.69275}, {"X"=329.53622, "Y"=232.43188}, {"X"=345.05795, "Y"=232.17102}, {"X"=360.5797, "Y"=231.91014}, {"X"=376.10144, "Y"=231.64928}, {"X"=391.62317, "Y"=231.38841}, {"X"=407.14493, "Y"=231.12753}, {"X"=422.66666, "Y"=230.86667}, {"X"=66.0, "Y"=252.40001}, {"X"=81.521736, "Y"=252.13914}, {"X"=97.04348, "Y"=251.87827}, {"X"=112.565216, "Y"=251.6174}, {"X"=128.08696, "Y"=251.35654}, {"X"=143.6087, "Y"=251.09566}, {"X"=159.13043, "Y"=250.8348}, {"X"=174.65218, "Y"=250.57393}, {"X"=190.17392, "Y"=250.31305}, {"X"=205.69565, "Y"=250.05219}, {"X"=221.21739, "Y"=249.79132}, {"X"=236.73914, "Y"=249.53044}, {"X"=252.26086, "Y"=249.26958}, {"X"=267.78262, "Y"=249.0087}, {"X"=283.30435, "Y"=248.74783}, {"X"=298.82608, "Y"=248.48697}, {"X"=314.34784, "Y"=248.22609}, {"X"=329.86957, "Y"=247.96523}, {"X"=345.3913, "Y"=247.70436}, {"X"=360.91306, "Y"=247.44348}, {"X"=376.43478, "Y"=247.18262}, {"X"=391.9565, "Y"=246.92175}, {"X"=407.47827, "Y"=246.66087}, {"X"=423.0, "Y"=246.40001}, {"X"=66.333336, "Y"=267.93335}, {"X"=81.85507, "Y"=267.6725}, {"X"=97.37681, "Y"=267.4116}, {"X"=112.89855, "Y"=267.15073}, {"X"=128.42029, "Y"=266.88986}, {"X"=143.94203, "Y"=266.62897}, {"X"=159.46376, "Y"=266.3681}, {"X"=174.9855, "Y"=266.10724}, {"X"=190.50725, "Y"=265.84637}, {"X"=206.02898, "Y"=265.5855}, {"X"=221.55072, "Y"=265.32465}, {"X"=237.07246, "Y"=265.06378}, {"X"=252.5942, "Y"=264.80292}, {"X"=268.11594, "Y"=264.54202}, {"X"=283.6377, "Y"=264.28116}, {"X"=299.15942, "Y"=264.0203}, {"X"=314.68115, "Y"=263.7594}, {"X"=330.2029, "Y"=263.49854}, {"X"=345.72464, "Y"=263.23767}, {"X"=361.2464, "Y"=262.9768}, {"X"=376.76813, "Y"=262.71594}, {"X"=392.28986, "Y"=262.45508}, {"X"=407.8116, "Y"=262.1942}, {"X"=423.33334, "Y"=261.93335}, {"X"=66.666664, "Y"=283.46667}, {"X"=82.18841, "Y"=283.2058}, {"X"=97.710144, "Y"=282.94495}, {"X"=113.23188, "Y"=282.68408}, {"X"=128.75362, "Y"=282.42322}, {"X"=144.27536, "Y"=282.16232}, {"X"=159.7971, "Y"=281.90146}, {"X"=175.31885, "Y"=281.6406}, {"X"=190.84058, "Y"=281.3797}, {"X"=206.36232, "Y"=281.11884}, {"X"=221.88406, "Y"=280.85797}, {"X"=237.4058, "Y"=280.5971}, {"X"=252.92754, "Y"=280.33624}, {"X"=268.44928, "Y"=280.07538}, {"X"=283.971, "Y"=279.8145}, {"X"=299.49274, "Y"=279.55365}, {"X"=315.0145, "Y"=279.29276}, {"X"=330.53622, "Y"=279.0319}, {"X"=346.05795, "Y"=278.77103}, {"X"=361.5797, "Y"=278.51013}, {"X"=377.10144, "Y"=278.24927}, {"X"=392.62317, "Y"=277.9884}, {"X"=408.14493, "Y"=277.72754}, {"X"=423.66666, "Y"=277.46667}, {"X"=67.0, "Y"=299.0}, {"X"=82.521736, "Y"=298.73914}, {"X"=98.04348, "Y"=298.47827}, {"X"=113.565216, "Y"=298.2174}, {"X"=129.08696, "Y"=297.95654}, {"X"=144.6087, "Y"=297.69565}, {"X"=160.13043, "Y"=297.43478}, {"X"=175.65218, "Y"=297.17392}, {"X"=191.17392, "Y"=296.91302}, {"X"=206.69565, "Y"=296.65216}, {"X"=222.21739, "Y"=296.3913}, {"X"=237.73914, "Y"=296.13043}, {"X"=253.26086, "Y"=295.86957}, {"X"=268.78262, "Y"=295.6087}, {"X"=284.30435, "Y"=295.34784}, {"X"=299.82608, "Y"=295.08698}, {"X"=315.34784, "Y"=294.82608}, {"X"=330.86957, "Y"=294.56522}, {"X"=346.3913, "Y"=294.30435}, {"X"=361.91306, "Y"=294.04346}, {"X"=377.43478, "Y"=293.7826}, {"X"=392.9565, "Y"=293.52173}, {"X"=408.47827, "Y"=293.26086}, {"X"=424.0, "Y"=293.0}] {"Y" format="%.2f"; "X" format="%.2f"}
  out "Image":T1(plugin-control)
  out "FreezeTemp":dbl=-0.8390476190476193 caption="Froze at" format="%.3g °C"
  out "Title 2":string="Well Data" caption="Version"
  out "Well":string="D23"
  out "CurTemp":dbl=1.5766666666667106 caption="Temp" format="%.3g °C"
  out "Contents":string="E, 1mg/ml Snomax in D2O"
  out "Temps":dbl[][](graph)
  out "Temps single":dbl[](graph)=[5.531428571428592, 5.503809523809593, 5.5400000000000205, 5.459047619047681, 5.39714285714291, 5.2928571428571445, 5.241428571428628, 5.18428571428575, 5.007142857142867, 4.931904761904775, 4.809523809523853, 4.909047619047669, 4.747142857142876, 4.635238095238094, 4.415238095238124, 4.284761904761922, 4.249047619047644, 4.226190476190482, 4.137619047619069, 4.0109523809524035, 3.944761904761947, 3.7904761904762267, 3.8252380952381486, 3.7423809523809837, 3.571428571428612, 3.4947619047619582, 3.4966666666667265, 3.329047619047685, 3.245714285714314, 3.2019047619048138, 3.0895238095238255, 3.009047619047635, 2.9138095238095616, 2.716666666666697, 2.677619047619089, 2.543809523809557, 2.5214285714286007, 2.342857142857156, 2.3033333333333417, 2.276190476190493, 2.181904761904775, 2.0571428571428783, 1.9038095238095707, 1.827142857142917, 1.7461904761904634, 1.582857142857165, 1.5066666666667174, 1.5004761904762063, 1.5095238095238415, 1.36047619047622, 1.2328571428571422, 1.1666666666666856, 1.0000000000000568, 0.9819047619047865, 0.9090476190476693, 0.7404761904762154, 0.6947619047619469, 0.5071428571428669, 0.4980952380952317, 0.3190476190476375, 0.2890476190476647, 0.1800000000000068, 0.1114285714286325, 0.0323809523810041, -0.11761904761903, -0.1738095238094957, -0.1942857142856838, -0.150952380952333, -0.2676190476190072, -0.4671428571428464, -0.5428571428570876, -0.589999999999975, -0.6971428571428078, -0.8390476190476193, 1.5766666666667106, 1.95952380952383, 2.0919047619048, 2.090476190476238, 2.009047619047635, 1.9466666666667152, 2.033809523809566, 1.9204761904762222, 1.8066666666667288, 1.8442857142857747, 1.9061904761904884, 1.8423809523810064, 1.7100000000000364, 1.6704761904762222, 1.3585714285714516, 1.2161904761904907, 1.0633333333333326, 0.6014285714286416, -0.1571428571428441, -1.8128571428571263, -2.284761904761865, -2.4685714285714084, -2.5480952380951862, -2.772857142857106, -2.9495238095237823, -3.04047619047617, -3.0866666666666447, -3.2666666666666515, -3.2504761904761494, -3.4014285714285393, -3.3957142857142344, -3.4771428571428373, -3.5528571428571354, -3.7219047619047387, -3.8114285714285643, -3.8347619047618764, -3.9480952380952203, -4.072380952380911, -4.1604761904761745, -4.1795238095238005, -4.307142857142821, -4.550476190476161, -4.605714285714271, -4.532380952380947, -4.656666666666638, -4.8261904761904475, -5.041904761904732, -5.182857142857131, -5.24666666666667, -5.395714285714234, -5.435714285714255, -5.539999999999964, -5.619999999999948, -5.719047619047615, -5.802380952380929, -5.90476190476187, -5.913809523809505, -6.07714285714286, -6.1314285714285575, -6.181904761904718, -6.393809523809523, -6.40428571428572, -6.553333333333285, -6.642380952380904, -6.7433333333332826, -6.719047619047615, -6.798095238095186, -6.927142857142826, -6.949999999999989, -7.055714285714259, -7.2071428571428555, -7.288095238095195, -7.363809523809493, -7.359047619047601, -7.540952380952319, -7.679047619047594, -7.8609523809523125, -8.032380952380947, -8.09904761904761, -8.176666666666677, -8.109999999999957, -8.318095238095225, -8.435238095238049, -8.5223809523809, -8.626190476190459, -8.63904761904763, -8.766666666666652, -8.849523809523816, -8.879999999999995, -9.036666666666633, -9.213809523809516, -9.259047619047578, -9.36761904761903, -9.445714285714246, -9.556190476190409, -9.661428571428587, -9.745714285714257, -9.806666666666672, -9.899523809523771, -9.993809523809489, -9.99523809523805, -10.209523809523773, -10.362380952380931, -10.39619047619044, -10.470952380952326, -10.555238095238053, -10.68809523809523, -10.715238095238078, -10.897619047619003, -10.826666666666654, -10.890476190476136, -10.989999999999952, -11.12952380952379, -11.251428571428562, -11.412380952380943, -11.38952380952378, -11.67999999999995, -11.625714285714253, -11.720476190476177, -11.84238095238095, -11.945714285714246, -12.1580952380952, -12.155714285714225, -12.1795238095238, -12.384761904761888, -12.415238095238067, -12.494761904761901, -12.440952380952353, -12.708095238095211, -12.774285714285725, -12.91809523809519, -12.98142857142858, -13.10619047619042, -13.224761904761863, -13.212380952380954, -13.304285714285697, -13.497619047619025, -13.524761904761874, -13.59095238095233, -13.619999999999948, -13.773809523809518, -13.859999999999957, -13.949999999999989, -14.326190476190447, -14.24190476190472, -14.28380952380951, -14.489047619047597, -14.570476190476143, -14.707142857142856, -14.692380952380915, -14.773809523809518, -14.759523809523785, -14.943333333333271, -15.14619047619044, -15.155238095238076, -15.373333333333278, -15.363333333333287, -15.421904761904727, -15.485714285714266, -15.641904761904755, -15.760952380952347, -15.869523809523798, -15.875714285714253, -15.970952380952326, -16.12952380952379, -16.152380952380952, -16.3590476190476, -16.2938095238095, -16.54571428571427, -16.550952380952367, -16.660476190476174, -16.9080952380952, -16.85619047619042, -16.9347619047619, -17.084761904761876, -17.19666666666666, -17.231428571428552, -17.292380952380938, -17.49857142857138, -17.575238095238063, -17.656666666666638, -17.806190476190437, -17.84619047619043, -18.00047619047615, -18.05571428571426, -18.091428571428565, -18.206190476190443, -18.33095238095234, -18.39619047619044, -18.445238095238068, -18.609999999999985, -18.67999999999998, -18.8342857142857, -18.83761904761903, -18.94999999999996, -19.130476190476145, -19.26666666666665, -19.252857142857096, -19.274761904761874, -19.36285714285711, -19.34571428571425, -19.46333333333328, -19.65619047619043, -19.664285714285683, -19.950476190476166, -20.024285714285696, -20.09095238095233, -20.14809523809521, -20.31714285714284, -20.369047619047592, -20.452857142857113, -20.549523809523777, -20.618095238095208, -20.742857142857105, -20.832857142857108, -20.893809523809523, -20.974285714285685, -21.059523809523796, -21.206190476190443, -21.36285714285711, -21.47666666666666, -21.578571428571394, -21.68999999999997, -21.658571428571378, -21.732380952380936, -21.763333333333293, -21.907142857142844, -21.959047619047595, -22.029523809523795, -22.169047619047603, -22.30571428571426, -22.39142857142855, -22.53190476190474, -22.746190476190435, -22.792380952380938, -22.68333333333328, -22.962857142857104, -23.052857142857107, -23.15952380952379, -23.083333333333286, -23.163809523809505, -23.35095238095235, -23.495714285714257, -23.619047619047592, -23.575238095238063, -23.637619047619012, -23.736190476190444, -23.747619047619025, -23.9295238095238, -24.160476190476146, -24.250952380952327, -24.212380952380926, -24.39142857142855, -24.514285714285705, -24.68476190476187, -24.86619047619044, -24.85952380952378, -24.889047619047602, -25.12904761904761, -25.079523809523778, -25.116666666666646, -25.322857142857117, -25.45809523809521, -25.391904761904755, -25.62619047619043, -25.649999999999977, -25.594761904761867, -25.651428571428568, -25.831904761904752, -25.946190476190424, -26.054761904761875, -26.24190476190475, -26.180952380952334, -26.28095238095233, -26.34095238095233, -26.318571428571374, -26.642380952380933, -26.80047619047616, -26.762857142857115, -26.930952380952334, -27.172380952380934, -27.30238095238093, -27.413809523809505, -27.41999999999996, -27.529999999999973, -27.558571428571383, -27.775238095238052, -27.76190476190473, -28.038095238095195, -28.036190476190427, -28.212857142857104, -28.115238095238055, -28.402380952380923, -28.39761904761903, -28.573333333333295, -28.766190476190445, -28.779047619047617, -28.82238095238094, -28.895714285714234, -29.014761904761883, -29.07095238095235, -29.375238095238075, -29.472857142857123, -29.380476190476145, -29.431904761904747, -29.69476190476189, -29.63809523809519, -29.860476190476163, -30.029047619047617, -30.121904761904744, -30.072857142857117, -30.15428571428569, -30.343333333333305, -30.31428571428569, -30.46857142857138, -30.605238095238064, -30.667619047619013, -30.798571428571393, -30.747142857142848, -30.910476190476146, -30.98190476190473, -31.308571428571383, -31.384761904761888, -31.516190476190445, -31.348095238095198, -31.589999999999975, -31.69999999999996, -31.81238095238092, -31.89761904761903, -32.05571428571426, -31.9733333333333, -32.23857142857139, -32.42142857142855, -32.463809523809516, -32.5333333333333, -32.412380952380914, -32.667142857142835, -32.752857142857124, -32.83809523809521, -32.97714285714284, -32.939047619047614, -33.05666666666664, -33.273333333333284, -33.22476190476189, -33.273333333333284, -33.51761904761901, -33.53142857142856, -33.61380952380952, -33.79619047619042, -34.02095238095234, -34.02857142857138, -34.016190476190445, -34.12761904761902, -34.31666666666666, -34.5790476190476, -34.529523809523795, -34.47238095238092, -34.571428571428555, -34.78666666666666, -34.890476190476164, -34.9890476190476, -35.024285714285696, -35.15952380952379, -35.244285714285695, -35.45619047619044, -35.30047619047616, -35.47999999999996, -35.62904761904761, -35.64333333333329, -35.6528571428571, -35.80095238095234, -35.851904761904734, -36.02761904761903, -36.151904761904746, -36.08619047619044, -36.3728571428571, -36.380476190476145, -36.53523809523807, -36.66523809523807, -36.78904761904761, -36.845238095238074, -37.170476190476165, -37.24190476190475, -37.22380952380951, -37.3590476190476, -37.420476190476165, -37.4595238095238, -37.44476190476189, -37.5328571428571, -37.51047619047617, -37.69999999999996, -37.91476190476189, -37.97714285714284, -38.1742857142857, -38.30619047619044, -38.421904761904756, -38.47380952380951, -38.55571428571426, -38.61142857142855, -38.63095238095235, -38.97952380952378, -38.98190476190473, -38.965714285714256, -39.0790476190476, -39.22190476190474, -39.274285714285696, -39.51095238095235, -39.719047619047615, -39.696190476190424, -39.70999999999998, -39.70333333333329, -39.70476190476188, -39.75190476190474, -39.682380952380925, -39.7938095238095, -39.970952380952326, -40.03571428571425, -39.859999999999985, -40.05714285714282, -40.04999999999998, -40.076666666666654, -40.11047619047616, -40.12571428571425, -40.0328571428571, -40.13238095238091, -40.14809523809521, -40.37142857142857, -40.28428571428569, -40.34190476190474, -40.376666666666665, -40.421904761904756, -40.482380952380936, -40.49666666666664, -40.49666666666664, -40.600476190476144, -40.66142857142856, -40.61476190476188, -40.712380952380926, -40.66095238095235, -40.81523809523807, -40.91952380952378, -41.0895238095238, -41.02190476190475, -40.93523809523808, -40.95857142857139, -41.03761904761902, -41.115238095238055, -41.1795238095238, -41.12380952380951, -41.131904761904735, -41.15238095238092, -41.2095238095238, -41.224285714285685, -41.249523809523794]
  out "Temps single grad":dbl[](graph)=[0.0, -0.027619047618998138, 0.036190476190427034, -0.08095238095233981, -0.06190476190477057, -0.10428571428576561, -0.051428571428516534, -0.057142857142878256, -0.1771428571428828, -0.07523809523809177, -0.12238095238092228, 0.09952380952381645, -0.1619047619047933, -0.11190476190478194, -0.21999999999997044, -0.13047619047620174, -0.035714285714277594, -0.02285714285716267, -0.08857142857141298, -0.12666666666666515, -0.06619047619045659, -0.15428571428572013, 0.03476190476192187, -0.08285714285716494, -0.17095238095237164, -0.07666666666665378, 0.0019047619047682929, -0.16761904761904134, -0.08333333333337123, -0.043809523809500206, -0.11238095238098822, -0.08047619047619037, -0.09523809523807358, -0.1971428571428646, -0.039047619047607895, -0.13380952380953204, -0.022380952380956387, -0.1785714285714448, -0.03952380952381418, -0.027142857142848698, -0.09428571428571786, -0.12476190476189686, -0.15333333333330756, -0.07666666666665378, -0.0809523809524535, -0.16333333333329847, -0.0761904761904475, -0.006190476190511163, 0.00904761904763518, -0.14904761904762154, -0.12761904761907772, -0.06619047619045659, -0.16666666666662877, -0.01809523809527036, -0.0728571428571172, -0.1685714285714539, -0.0457142857142685, -0.18761904761908, -0.00904761904763518, -0.1790476190475942, -0.029999999999972826, -0.10904761904765789, -0.0685714285713743, -0.07904761904762839, -0.1500000000000341, -0.05619047619046569, -0.020476190476188122, 0.04333333333335082, -0.11666666666667419, -0.19952380952383925, -0.07571428571424121, -0.04714285714288735, -0.10714285714283278, -0.1419047619048115, 2.41571428571433, 0.38285714285711947, 0.13238095238097003, -0.0014285714285620088, -0.08142857142860294, -0.06238095238092001, 0.08714285714285097, -0.11333333333334394, -0.11380952380949338, 0.03761904761904589, 0.06190476190471372, -0.06380952380948202, -0.13238095238097003, -0.03952380952381418, -0.31190476190477057, -0.14238095238096093, -0.15285714285715812, -0.461904761904691, -0.7585714285714857, -1.6557142857142821, -0.47190476190473873, -0.1838095238095434, -0.0795238095237778, -0.2247619047619196, -0.17666666666667652, -0.09095238095238756, -0.04619047619047478, -0.18000000000000682, 0.016190476190502068, -0.15095238095238983, 0.005714285714304879, -0.08142857142860294, -0.07571428571429806, -0.16904761904760335, -0.08952380952382555, -0.023333333333312112, -0.11333333333334394, -0.12428571428569057, -0.08809523809526354, -0.019047619047626085, -0.12761904761902088, -0.2433333333333394, -0.05523809523810996, 0.07333333333332348, -0.12428571428569057, -0.16952380952380963, -0.21571428571428442, -0.14095238095239893, -0.06380952380953886, -0.1490476190475647, -0.040000000000020464, -0.10428571428570876, -0.07999999999998408, -0.09904761904766701, -0.08333333333331439, -0.10238095238094047, -0.00904761904763518, -0.1633333333333553, -0.054285714285697395, -0.05047619047616081, -0.21190476190480467, -0.010476190476197189, -0.1490476190475647, -0.08904761904761926, -0.10095238095237846, 0.024285714285667837, -0.07904761904757152, -0.12904761904763973, -0.02285714285716267, -0.10571428571427077, -0.15142857142859611, -0.08095238095233981, -0.07571428571429806, 0.0047619047618923105, -0.18190476190471827, -0.1380952380952749, -0.18190476190471827, -0.17142857142863477, -0.06666666666666288, -0.07761904761906635, 0.06666666666671972, -0.2080952380952681, -0.11714285714282369, -0.08714285714285097, -0.10380952380955932, -0.012857142857171766, -0.12761904761902088, -0.08285714285716494, -0.030476190476179, -0.15666666666663787, -0.1771428571428828, -0.045238095238062215, -0.10857142857145163, -0.07809523809521579, -0.11047619047616308, -0.10523809523817818, -0.08428571428567011, -0.06095238095241484, -0.092857142857099, -0.09428571428571786, -0.0014285714285620088, -0.2142857142857224, -0.15285714285715812, -0.0338095238095093, -0.07476190476188549, -0.08428571428572695, -0.1328571428571763, -0.027142857142848698, -0.18238095238092455, 0.0709523809523489, -0.06380952380948202, -0.09952380952381645, -0.13952380952383692, -0.12190476190477284, -0.16095238095238074, 0.02285714285716267, -0.2904761904761699, 0.054285714285697395, -0.09476190476192414, -0.12190476190477284, -0.1033333333332962, -0.2123809523809541, 0.002380952380974577, -0.02380952380957524, -0.20523809523808723, -0.030476190476179, -0.07952380952383464, 0.053809523809547954, -0.2671428571428578, -0.06619047619051344, -0.1438095238094661, -0.06333333333338942, -0.12476190476184001, -0.11857142857144254, 0.012380952380908639, -0.09190476190474328, -0.19333333333332803, -0.027142857142848698, -0.06619047619045659, -0.02904761904761699, -0.1538095238095707, -0.0861904761904384, -0.09000000000003183, -0.37619047619045887, 0.08428571428572695, -0.041904761904788757, -0.20523809523808723, -0.08142857142854609, -0.1366666666667129, 0.014761904761940059, -0.08142857142860294, 0.014285714285733775, -0.18380952380948656, -0.2028571428571695, -0.00904761904763518, -0.21809523809520215, 0.009999999999990905, -0.058571428571440265, -0.06380952380953886, -0.15619047619048843, -0.11904761904759198, -0.10857142857145163, -0.006190476190454319, -0.09523809523807358, -0.158571428571463, -0.02285714285716267, -0.20666666666664923, 0.06523809523810087, -0.2519047619047683, -0.0052380952380985946, -0.10952380952380736, -0.24761904761902542, 0.05190476190477966, -0.07857142857147892, -0.14999999999997726, -0.11190476190478194, -0.03476190476189345, -0.06095238095238642, -0.20619047619044295, -0.0766666666666822, -0.08142857142857451, -0.1495238095237994, -0.03999999999999204, -0.15428571428572013, -0.05523809523810996, -0.035714285714306016, -0.11476190476187753, -0.12476190476189686, -0.06523809523810087, -0.04904761904762722, -0.16476190476191732, -0.06999999999999318, -0.15428571428572013, -0.0033333333333303017, -0.11238095238093138, -0.18047619047618468, -0.13619047619050662, 0.013809523809555913, -0.021904761904778525, -0.08809523809523512, 0.017142857142857792, -0.11761904761902997, -0.19285714285715017, -0.008095238095251034, -0.2861904761904839, -0.07380952380952976, -0.06666666666663446, -0.057142857142878256, -0.16904761904763177, -0.05190476190475124, -0.08380952380952067, -0.09666666666666401, -0.06857142857143117, -0.12476190476189686, -0.09000000000000341, -0.06095238095241484, -0.08047619047616195, -0.0852380952381111, -0.14666666666664696, -0.1566666666666663, -0.11380952380955023, -0.10190476190473419, -0.11142857142857565, 0.03142857142859157, -0.07380952380955819, -0.03095238095235686, -0.14380952380955137, -0.05190476190475124, -0.07047619047619946, -0.1395238095238085, -0.13666666666665606, -0.08571428571428896, -0.14047619047619264, -0.21428571428569398, -0.046190476190503205, 0.10904761904765792, -0.2795238095238233, -0.09000000000000341, -0.10666666666668334, 0.07619047619050434, -0.08047619047621879, -0.1871428571428453, -0.1447619047619071, -0.12333333333333485, 0.04380952380952863, -0.06238095238094843, -0.0985714285714323, -0.011428571428581336, -0.18190476190477511, -0.2309523809523455, -0.09047619047618127, 0.03857142857140161, -0.17904761904762267, -0.12285714285715699, -0.17047619047616536, -0.18142857142856883, 0.006666666666660603, -0.029523809523823275, -0.2400000000000091, 0.049523809523833506, -0.037142857142868024, -0.20619047619047137, -0.13523809523809405, 0.06619047619045659, -0.2342857142856758, -0.023809523809546818, 0.05523809523810996, -0.056666666666700394, -0.18047619047618468, -0.11428571428567125, -0.10857142857145163, -0.1871428571428737, 0.06095238095241484, -0.09999999999999432, -0.060000000000002274, 0.022380952380956387, -0.3238095238095582, -0.1580952380952283, 0.03761904761904589, -0.1680952380952192, -0.24142857142859953, -0.12999999999999545, -0.11142857142857565, -0.006190476190454319, -0.11000000000001364, -0.028571428571410706, -0.21666666666666856, 0.013333333333321207, -0.27619047619046455, 0.0019047619047682929, -0.17666666666667652, 0.09761904761904816, -0.287142857142868, 0.0047619047618923105, -0.17571428571426395, -0.19285714285715017, -0.012857142857171766, -0.043333333333322344, -0.07333333333329506, -0.11904761904764882, -0.05619047619046569, -0.3042857142857258, -0.09761904761904816, 0.09238095238097799, -0.0514285714286018, -0.26285714285714334, 0.056666666666700394, -0.22238095238097344, -0.1685714285714539, -0.09285714285712743, 0.04904761904762722, -0.08142857142857451, -0.18904761904761358, 0.02904761904761699, -0.1542857142856917, -0.13666666666668448, -0.06238095238094843, -0.1309523809523796, 0.051428571428544956, -0.16333333333329847, -0.07142857142858361, -0.3266666666666538, -0.07619047619050434, -0.13142857142855746, 0.16809523809524762, -0.2419047619047774, -0.10999999999998522, -0.1123809523809598, -0.0852380952381111, -0.1580952380952283, 0.08238095238095866, -0.2652380952380895, -0.18285714285715926, -0.04238095238096662, -0.0695238095237869, 0.1209523809523887, -0.25476190476192073, -0.08571428571428896, -0.08523809523808268, -0.13904761904763063, 0.03809523809522375, -0.11761904761902997, -0.21666666666664014, 0.048571428571392516, -0.048571428571392516, -0.24428571428572354, -0.013809523809555913, -0.08238095238095866, -0.18238095238089613, -0.2247619047619196, -0.00761904761904475, 0.01238095238093706, -0.11142857142857565, -0.189047619047642, -0.26238095238093706, 0.049523809523805085, 0.057142857142878256, -0.09904761904763859, -0.21523809523810655, -0.10380952380950248, -0.0985714285714323, -0.03523809523809973, -0.13523809523809405, -0.08476190476190482, -0.21190476190474783, 0.15571428571428214, -0.17952380952380054, -0.14904761904764996, -0.014285714285676931, -0.009523809523813043, -0.1480952380952374, -0.050952380952395515, -0.17571428571429237, -0.124285714285719, 0.06571428571430715, -0.28666666666666174, -0.00761904761904475, -0.15476190476192642, -0.12999999999999545, -0.12380952380954113, -0.05619047619046569, -0.3252380952380918, -0.07142857142858361, 0.01809523809524194, -0.13523809523809405, -0.06142857142856428, -0.03904761904763632, 0.014761904761911637, -0.0880952380952067, 0.022380952380927965, -0.18952380952379144, -0.2147619047619287, -0.06238095238094843, -0.1971428571428646, -0.13190476190473532, -0.11571428571431852, -0.05190476190475124, -0.08190476190475238, -0.055714285714287826, -0.019523809523803948, -0.3485714285714323, -0.0023809523809461552, 0.016190476190473646, -0.11333333333334394, -0.1428571428571388, -0.052380952380957524, -0.23666666666665037, -0.2080952380952681, 0.022857142857191093, -0.013809523809555913, 0.006666666666689025, -0.0014285714285904305, -0.04714285714285893, 0.06952380952381532, -0.11142857142857565, -0.17714285714282596, -0.064761904761923, 0.17571428571426395, -0.1971428571428362, 0.007142857142838466, -0.026666666666670835, -0.0338095238095093, -0.0152380952380895, 0.09285714285715585, -0.09952380952381645, -0.015714285714295784, -0.2233333333333576, 0.08714285714287939, -0.05761904761905612, -0.03476190476192187, -0.045238095238090636, -0.060476190476180136, -0.014285714285705353, 0.0, -0.10380952380950248, -0.06095238095241484, 0.04666666666668107, -0.09761904761904816, 0.05142857142857338, -0.15428571428572013, -0.10428571428570876, -0.17000000000001592, 0.06761904761904702, 0.08666666666667311, -0.023333333333312112, -0.07904761904762836, -0.07761904761903793, -0.06428571428574514, 0.055714285714287826, -0.008095238095222612, -0.020476190476188094, -0.057142857142878256, -0.014761904761883216, -0.025238095238108826]
  out "Temps grads":dbl[][](graph)
  # "hints: \nUse the Mouse Wheel to zoom in and out"
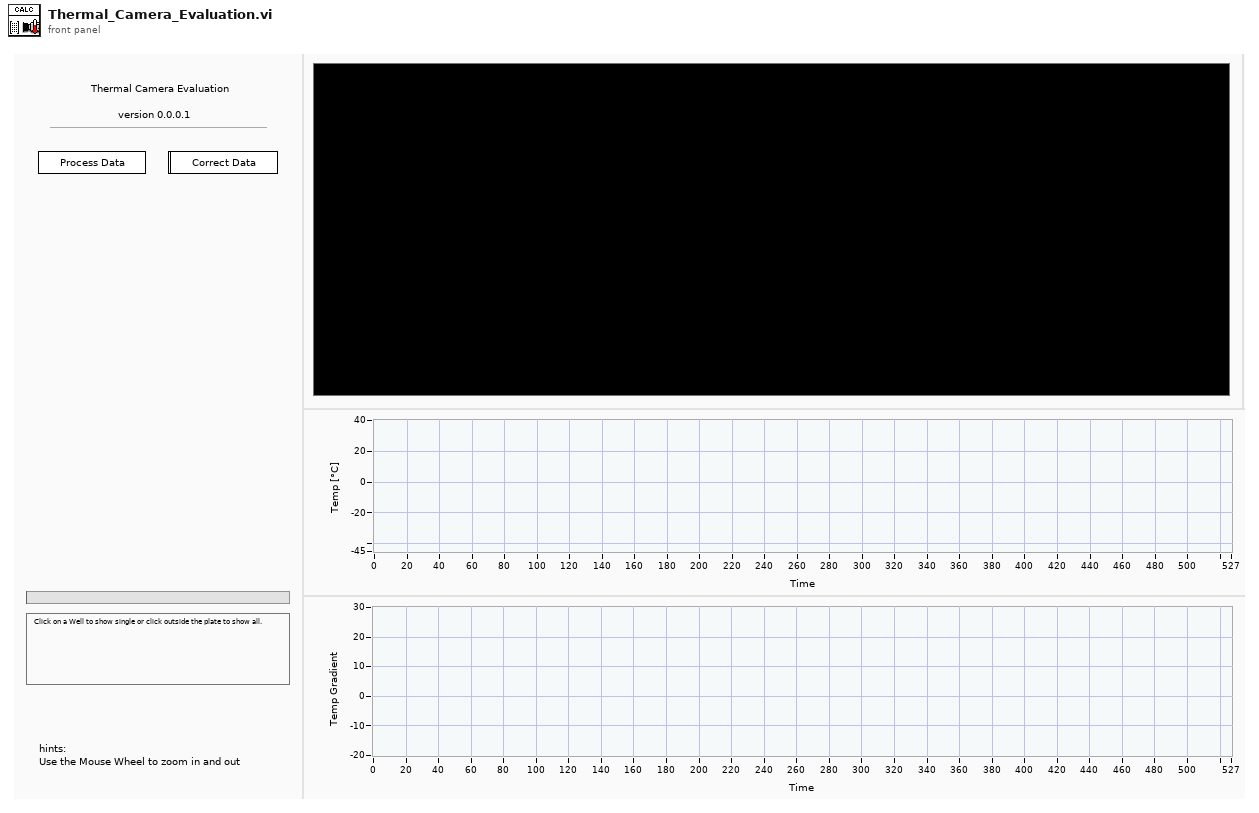
[diagram p1: front panel]
types:
  T1 = typedef "IMAQ Image.ctl" = refnum<image>
  T2 = typedef "IMAQ Point" = cluster{"X":sgl, "Y":sgl}
  T3 = enum32{"Invalid", "Standard", "Closed", "Hidden", "Minimized", "Maximized"}
  T4 = enum32{"invalid app kind", "Development System", "Run Time System", "Student Edition", "Embedded LabVIEW", "Evaluation", "Custom"}
  T5 = cluster{"Global Rectangle":i32[], "Contours":cluster{"Contour Type":u32, "ROI Type":u32, "Points":i32[]}[]}
  T6 = typedef "DataCluster_TCAL.ctl" = cluster{"Core":cluster{"Current VI Reference":refnum<vi>, "Close Panel on Exit?":bool}, "Image Out":T1, "State":i32, "Points":cluster{"Top Left":T2, "Top Right":T2, "Bottom Left":T2, "Bottom Right":T2, "x space 2":dbl, "y space 2":sgl, "x_space":sgl, "y_space":sgl, "Pixels":cluster{"X":i32, "Y":i32}[][], "Fixpoint":T2}, "img_array":T1[], "Temps":dbl[], "Temps_Array":dbl[][], "Scan Area":dbl, "Fixpoint Area":dbl, "PCR Size":u16}
  T7 = enum8{"Enabled", "Disabled", "Disabled and Grayed Out"}
  T8 = cluster{"Desired Font (Application)":enum16{"User-specified Font", "Application Font", "System Font", "Dialog Font"}, "[User-specified Font]":cluster{"Font Name":string, "Size":i16, "Strikeout?":bool, "Italic?":bool, "Underline?":bool, "Outline?":bool, "Shadow?":bool, "Bold?":bool, "Rotation Angle":dbl}, "Horizontal Alignment":i16, "Vertical Alignment":i16}
  T9 = typedef "ROI Descriptor" = cluster{"Global Rectangle":i32[], "Contours":cluster{"ID":enum32{"External", "Internal"}, "Type":u32, "Coordinates":i32[]}[]}
  T10 = typedef "Image Type" = u32
  T11 = cluster{"Top Left":T2, "Top Right":T2, "Bottom Left":T2, "Bottom Right":T2, "x space 2":dbl, "y space 2":sgl, "x_space":sgl, "y_space":sgl, "Pixels":cluster{"X":i32, "Y":i32}[][], "Fixpoint":T2}
  T12 = cluster{"Current VI Reference":refnum<vi>, "Close Panel on Exit?":bool}
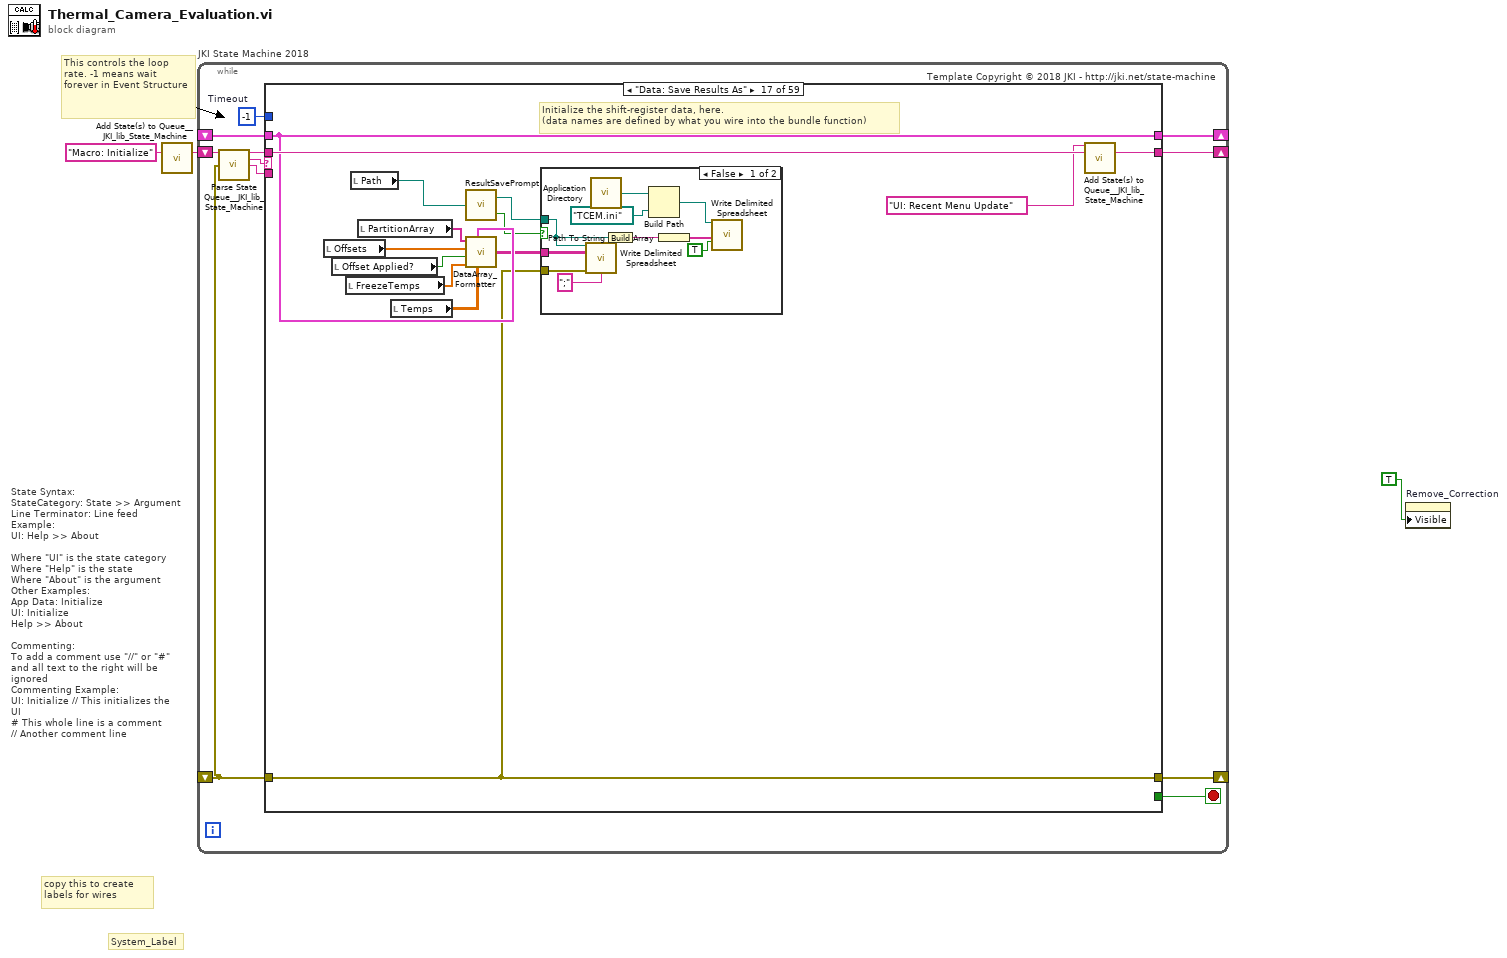
[diagram p0: block diagram]
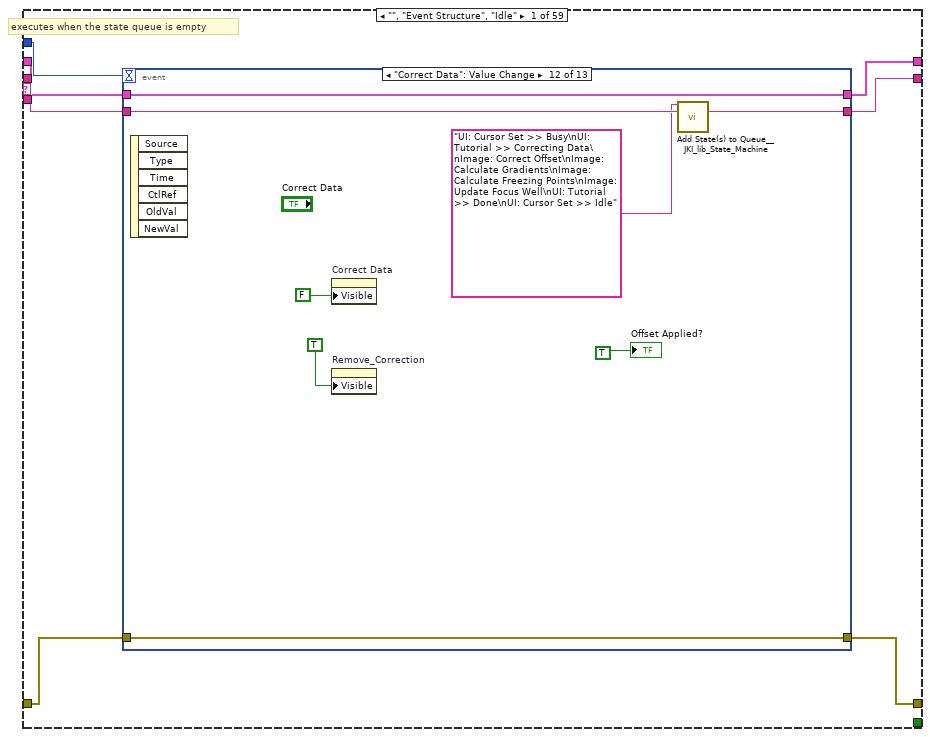
[diagram p2: hidden frame]
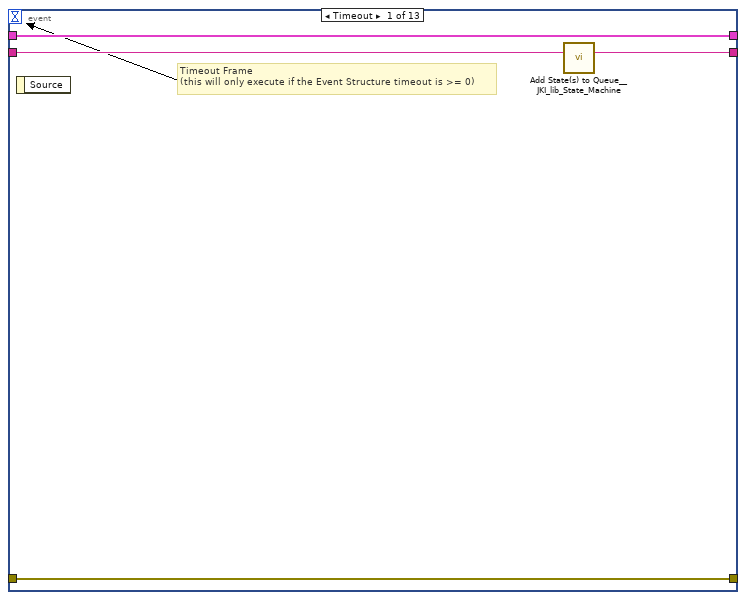
[diagram p3: hidden frame]
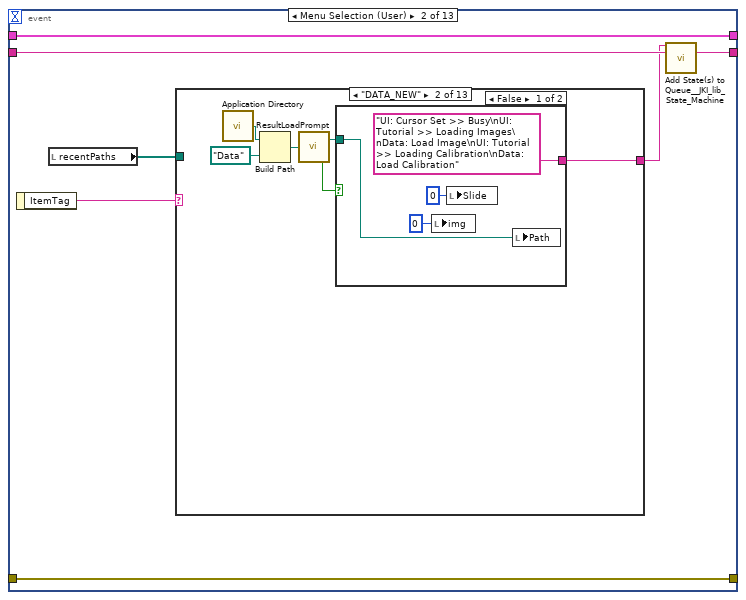
[diagram p4: hidden frame]
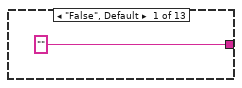
[diagram p5: hidden frame]
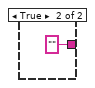
[diagram p6: hidden frame]
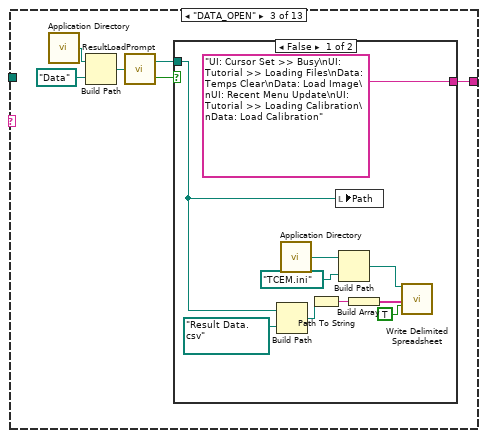
[diagram p7: hidden frame]
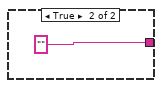
[diagram p8: hidden frame]
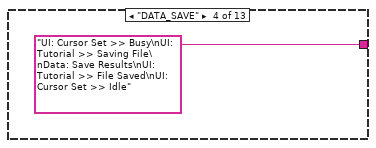
[diagram p9: hidden frame]
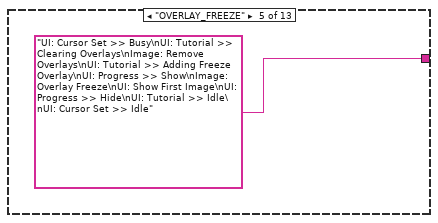
[diagram p10: hidden frame]
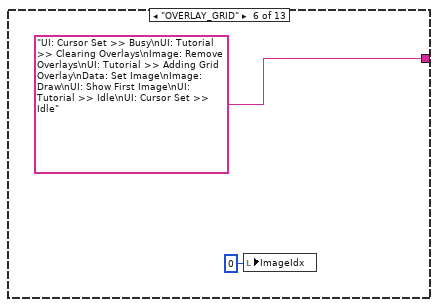
[diagram p11: hidden frame]
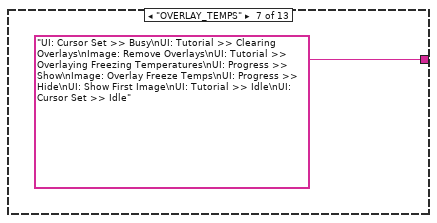
[diagram p12: hidden frame]
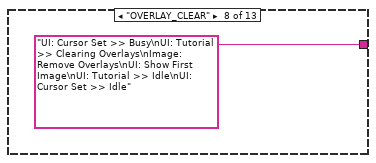
[diagram p13: hidden frame]
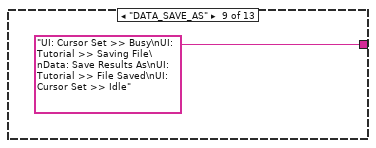
[diagram p14: hidden frame]
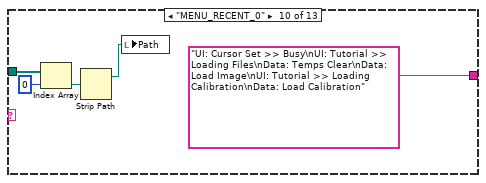
[diagram p15: hidden frame]
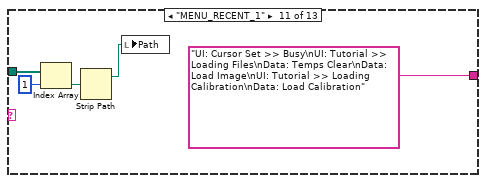
[diagram p16: hidden frame]
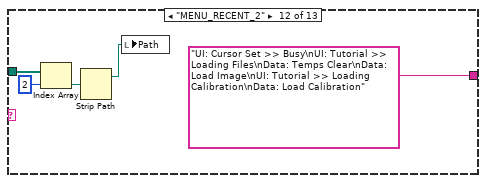
[diagram p17: hidden frame]
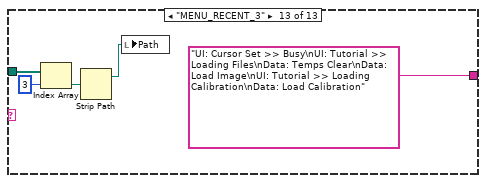
[diagram p18: hidden frame]
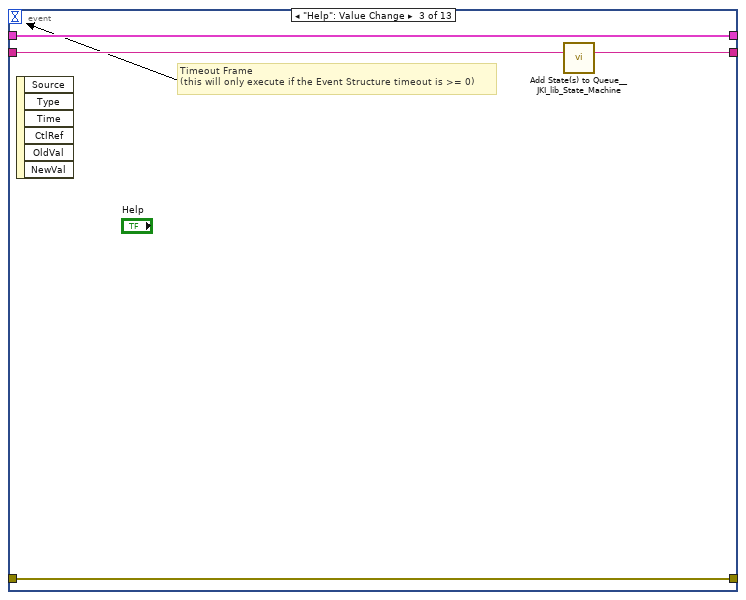
[diagram p19: hidden frame]
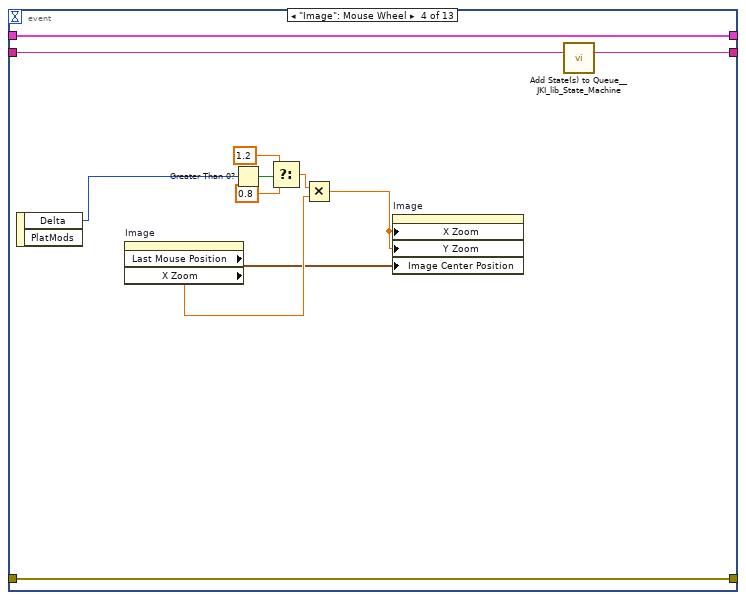
[diagram p20: hidden frame]
diagram:
  # "State Syntax:\nStateCategory: State >> Argument\nLine Terminator: Line feed\nExample:\nUI: Help >> About\n\nWhere \"UI\" is the state category\nWhere \"Help\" is the state\nWhere \"About\" is the argument\nOther Examples:\nApp Data: Initialize\nUI: Initialize\nHelp >> About\n\nCommenting:\nTo add a comment use \"//\" or \"#\" and all text to the right will be ignored\nCommenting Example:\nUI: Initialize // This initializes the UI\n# This whole line is a comment\n// Another comment line"
  # "copy this to create labels for wires"
  # "This controls the loop rate. -1 means wait forever in Event Structure"
  # "System_Label"
  n1 = call <vilib>:"Add State(s) to Queue__JKI_lib_State_Machine.vi"("State(s) in (\"\")"="Macro: Initialize") -> ("States Out"=w3:string)  [unwired: 14 in]
  n2 = while "JKI State Machine 2018" {
    shift-right: [w7] -> _
    shift-left: _ -> [w6]
    shift-right: [w10] -> _
    shift-left: _ -> [w4]
    shift-right: [w9] -> _
    shift-left: w3 -> [w11]
    stop <- w8 stop-if-true
    w5 = -1  # Timeout
    # "Template Copyright © 2018 JKI - http://jki.net/state-machine"
    n3 = call <vilib>:"Parse State Queue__JKI_lib_State_Machine.vi"("State Queue"=w11, "Error In (no error)"=w4) -> ("Remaining States"=w13:string, "Current State"=w14:string, "Arguments"=w12:string)  [unwired: 11 in]
    n4 = case shown="\"Data: Save Results As\"" w14 {
      selector: w14 -> [_ _ w187 _ _ _ _ _ _ _ _ _ _ _ _ _ _ _ _ _ _ _ _ _ _ _ _ _ _ _ _ _ _ _ _ _ _ _ _ _ _ _ _ _ _ _ _ _ _ _ _ _ _ _ _ _ _ _ _]
      tunnel: w13 -> [w21 w186 w191 w210 w216 w221 w225 w241 w298 w308 w335 w362 w375 w382 w389 w406 w435 w453 w460 w492 w500 w508 w515 w520 w527 w539 w551 w561 w571 w581 w592 w661 w666 w676 w680 w685 w690 w710 w724 w742 w762 w780 w791 w808 w874 w896 w916 w938 w982 w1011 w1034 w1063 w1106 w1146 w1181 w1194 w1215 w1225 w1234]
      tunnel: w12 -> [_ _ _ _ _ _ _ _ _ _ _ _ _ _ _ _ _ _ _ _ w496 _ _ w516 w523 w534 w547 w557 w567 w577 w586 _ _ _ _ _ _ _ _ _ _ _ _ w806 _ _ _ _ _ _ _ _ _ _ _ _ _ _ _]
      tunnel: w6 -> [w19 w183 w189 w203 w213 w219 w222 w228 w295 w305 w328 w358 _ w379 w386 w404 w433 w451 w457 w490 w498 w506 w512 w518 w525 w537 w549 w559 w569 w579 w588 w658 w663 w673 w677 w682 w687 w691 w722 w733 w753 w771 w786 w804 w861 w885 w905 w922 w968 w1008 w1031 w1060 w1103 w1141 w1178 w1185 w1212 w1222 w1231]
      tunnel: [w18 w184 w193 w207 errorcluster {"status"=FALSE, "code"=0, "source"=""} ("error out") w218 w223 w230 w292 w306 w333 w360 w363 w380 w387 w400 w428 w450 w458 w489 w497 w505 w513 w517 w524 w535 w548 w558 w568 w578 w589 w659 w664 w674 w678 w683 w688 w708 w719 w740 w760 w778 w783 w801 w871 w894 w914 w936 w980 w1009 w1032 w1061 w1104 w1144 w1179 w1192 w1213 w1223 w1232] -> w10
      tunnel: w4 -> [w17 w184 w192 w207 w212 w218 w223 w237 w292 w306 w333 w360 w363 w380 w387 w400 w428 w447 w458 w489 w497 w505 w513 w517 w524 w536 w548 w558 w568 w578 w590 w659 w664 w674 w678 w683 w688 w708 w720 w740 w760 w778 w785 w802 w871 w894 w914 w936 w980 w1009 w1032 w1061 w1104 w1144 w1179 w1192 w1213 w1223 w1232]
      tunnel: [w20 w185 w190 w209 w215 w220 w224 w240 w297 w307 w334 w361 w374 w381 w388 w405 w434 w452 w459 w491 w499 w507 w514 w519 w526 w538 w550 w560 w570 w580 w591 w660 w665 w675 w679 w684 w689 w709 w723 w741 w761 w779 w790 w807 w873 w895 w915 w937 w981 w1010 w1033 w1062 w1105 w1145 w1180 w1193 w1214 w1224 w1233] -> w9
      tunnel: [_ _ _ _ _ TRUE _ _ _ _ _ _ _ _ _ _ _ _ _ _ _ _ _ _ _ _ _ _ _ _ _ _ _ _ _ _ _ _ _ _ _ _ _ _ _ _ _ _ _ _ _ _ _ _ _ _ _ _ _] -> w8
      tunnel: [w16 w183 w189 w208 w213 w219 w222 w239 w296 w305 w327 w358 w373 w378 w386 w404 w433 w451 w457 w490 w498 w506 w512 w518 w525 w537 w549 w559 w569 w579 w588 w658 w663 w673 w677 w682 w687 w691 w722 w732 w752 w770 w786 w804 w860 w885 w905 w921 w968 w1008 w1031 w1060 w1103 w1141 w1178 w1185 w1212 w1222 w1231] -> w7
      tunnel: w5 -> [w15 _ _ _ _ _ _ _ _ _ _ _ _ _ _ _ _ _ _ _ _ _ _ _ _ _ _ _ _ _ _ _ _ _ _ _ _ _ _ _ _ _ _ _ _ _ _ _ _ _ _ _ _ _ _ _ _ _ _]
      frame "", "Event Structure", "Idle" {
        # "executes when the state queue is empty"
        n5 = event shown="[11] \"Correct Data\": Value Change" {
          selector: _ -> [_ _ _ _ _ _ _ _ _ _ _ _ _]
          dyn-events: _ -> [_ _ _ _ _ _ _ _ _ _ _ _ _]
          timeout: w15 -> [_ _ _ _ _ _ _ _ _ _ _ _ _]
          tunnel: w21 -> [w25 w32 w92 w104 w114 w120 w129 w138 w147 w156 w166 w174 w182]
          tunnel: [w24 w31 w91 w103 w113 w119 w128 w137 w146 w155 w165 w173 w181] -> w20
          tunnel: w19 -> [w22 w29 w89 w101 w111 w117 w126 w135 w144 w153 w163 w171 w179]
          tunnel: [w23 w30 w90 w102 w112 w118 w127 w136 w145 w154 w164 w172 w180] -> w18
          tunnel: w17 -> [w23 w30 w90 w102 w112 w118 w127 w136 w145 w154 w164 w172 w180]
          tunnel: [w22 w29 w89 w101 w111 w117 w126 w135 w144 w153 w163 w171 w179] -> w16
          event Timeout {
            # "Timeout Frame\n(this will only execute if the Event Structure timeout is >= 0)"
            n6 = event-data() -> ()  [unwired: 1 in, 1 out]
            n7 = call <vilib>:"Add State(s) to Queue__JKI_lib_State_Machine.vi"("State(s) in (\"\")"=w25) -> ("States Out"=w24:string)  [unwired: 14 in]
          }
          event Menu Selection (User) {
            n8 = event-data() -> ("ItemTag"=w28:string)  [unwired: 1 in]
            n9 = local read "recentPaths"() -> (w26:path[])
            n10 = case shown="\"DATA_NEW\"" w28 {
              tunnel: ["" w39 w50 "UI: Cursor Set >> Busy\nUI: Tutorial >> Saving File\nData: Save Results\nUI: Tutorial >> File Saved\nUI: Cursor Set >> Idle" "UI: Cursor Set >> Busy\nUI: Tutorial >> Clearing Overlays\nImage: Remove Overlays\nUI: Tutorial >> Adding Freeze Overlay\nUI: Progress >> Show\nImage: Overlay Freeze\nUI: Show First Image\nUI: Progress >> Hide\nUI: Tutorial >> Idle\nUI: Cursor Set >> Idle" "UI: Cursor Set >> Busy\nUI: Tutorial >> Clearing Overlays\nImage: Remove Overlays\nUI: Tutorial >> Adding Grid Overlay\nData: Set Image\nImage: Draw\nUI: Show First Image\nUI: Tutorial >> Idle\nUI: Cursor Set >> Idle" "UI: Cursor Set >> Busy\nUI: Tutorial >> Clearing Overlays\nImage: Remove Overlays\nUI: Tutorial >> Overlaying Freezing Temperatures\nUI: Progress >> Show\nImage: Overlay Freeze Temps\nUI: Progress >> Hide\nUI: Show First Image\nUI: Tutorial >> Idle\nUI: Cursor Set >> Idle" "UI: Cursor Set >> Busy\nUI: Tutorial >> Clearing Overlays\nImage: Remove Overlays\nUI: Show First Image\nUI: Tutorial >> Idle\nUI: Cursor Set >> Idle" "UI: Cursor Set >> Busy\nUI: Tutorial >> Saving File\nData: Save Results As\nUI: Tutorial >> File Saved\nUI: Cursor Set >> Idle" "UI: Cursor Set >> Busy\nUI: Tutorial >> Loading Files\nData: Temps Clear\nData: Load Image\nUI: Tutorial >> Loading Calibration\nData: Load Calibration" "UI: Cursor Set >> Busy\nUI: Tutorial >> Loading Files\nData: Temps Clear\nData: Load Image\nUI: Tutorial >> Loading Calibration\nData: Load Calibration" "UI: Cursor Set >> Busy\nUI: Tutorial >> Loading Files\nData: Temps Clear\nData: Load Image\nUI: Tutorial >> Loading Calibration\nData: Load Calibration" "UI: Cursor Set >> Busy\nUI: Tutorial >> Loading Files\nData: Temps Clear\nData: Load Image\nUI: Tutorial >> Loading Calibration\nData: Load Calibration"] -> w27
              tunnel: w26 -> [_ _ _ _ _ _ _ _ _ w72 w77 w82 w87]
              frame "False", Default {
              }
              frame "DATA_NEW" {
                n11 = call <vilib>:"Application Directory.vi"() -> ("Application Directory"=w38:path)
                n12 = Build Path(base path=w38, name or relative path=path "Data") -> (appended path=w37:path)
                n13 = call "ResultLoadPrompt.vi"("Path"=w37) -> ("selected path"=w34:path, "cancel?"=w35:bool)
                n14 = case shown="False" w35 {
                  tunnel: ["UI: Cursor Set >> Busy\nUI: Tutorial >> Loading Images\nData: Load Image\nUI: Tutorial >> Loading Calibration\nData: Load Calibration" ""] -> w39
                  tunnel: w34 -> [w40 _]
                  frame False {
                    n15 = local write "img"(0 ("img")) -> ()
                    n16 = local write "Slide"(u8 0 ("Slide")) -> ()
                    n17 = local write "Path"(w40) -> ()
                  }
                  frame True {
                  }
                }
              }
              frame "DATA_OPEN" {
                n18 = call <vilib>:"Application Directory.vi"() -> ("Application Directory"=w49:path)
                n19 = Build Path(base path=w49, name or relative path=path "Data") -> (appended path=w47:path)
                n20 = call "ResultLoadPrompt.vi"("Path"=w47) -> ("selected path"=w46:path, "cancel?"=w45:bool)
                n21 = case shown="False" w45 {
                  tunnel: ["UI: Cursor Set >> Busy\nUI: Tutorial >> Loading Files\nData: Temps Clear\nData: Load Image\nUI: Recent Menu Update\nUI: Tutorial >> Loading Calibration\nData: Load Calibration" ""] -> w50
                  tunnel: w46 -> [w59 _]
                  frame False {
                    n22 = Build Path(base path=w59, name or relative path=path "Result Data.csv") -> (appended path=w51:path)
                    n23 = call <vilib>:"Application Directory.vi"() -> ("Application Directory"=w55:path)
                    n24 = Path To String(path=w51) -> (string=w58:string)
                    n25 = local write "Path"(w59) -> ()
                    n26 = Build Path(base path=w55, name or relative path=path "TCEM.ini" ("file path (dialog if empty)")) -> (appended path=w56:path)
                    n27 = Build Array(w58) -> (w57:string[])
                    n28 = call-poly <vilib>:"Write Delimited Spreadsheet.vi"("file path (dialog if empty)"=w56, "1D data"=w57, "append to file? (new file:F)"=TRUE) -> ()  [unwired: 11 in, 2 out]
                  }
                  frame True {
                  }
                }
              }
              frame "DATA_SAVE" {
              }
              frame "OVERLAY_FREEZE" {
              }
              frame "OVERLAY_GRID" {
                n29 = local write "ImageIdx"(0 ("img")) -> ()
              }
              frame "OVERLAY_TEMPS" {
              }
              frame "OVERLAY_CLEAR" {
              }
              frame "DATA_SAVE_AS" {
              }
              frame "MENU_RECENT_0" {
                n30 = Index Array(array=w72, index=0) -> (element=w70:path)
                n31 = Strip Path(path=w70) -> (stripped path=w69:path)  [unwired: 1 out]
                n32 = local write "Path"(w69) -> ()
              }
              frame "MENU_RECENT_1" {
                n33 = Index Array(array=w77, index=1) -> (element=w75:path)
                n34 = Strip Path(path=w75) -> (stripped path=w74:path)  [unwired: 1 out]
                n35 = local write "Path"(w74) -> ()
              }
              frame "MENU_RECENT_2" {
                n36 = Index Array(array=w82, index=2) -> (element=w80:path)
                n37 = Strip Path(path=w80) -> (stripped path=w79:path)  [unwired: 1 out]
                n38 = local write "Path"(w79) -> ()
              }
              frame "MENU_RECENT_3" {
                n39 = Index Array(array=w87, index=3) -> (element=w85:path)
                n40 = Strip Path(path=w85) -> (stripped path=w84:path)  [unwired: 1 out]
                n41 = local write "Path"(w84) -> ()
              }
            }
            n42 = call <vilib>:"Add State(s) to Queue__JKI_lib_State_Machine.vi"("State(s) in Front (\"\")"=w27, "State(s) in (\"\")"=w32) -> ("States Out"=w31:string)  [unwired: 13 in]
          }
          event "Help": Value Change {
            # "Timeout Frame\n(this will only execute if the Event Structure timeout is >= 0)"
            n43 = event-data() -> ()  [unwired: 1 in, 6 out]
            n44 = call <vilib>:"Add State(s) to Queue__JKI_lib_State_Machine.vi"("State(s) in (\"\")"=w92) -> ("States Out"=w91:string)  [unwired: 14 in]
          }
          event "Image": Mouse Wheel {
            n45 = event-data() -> ("Delta"=w100:i32)  [unwired: 1 in, 1 out]
            n46 = property on="Image" class="ImageControl"() -> ("Last Mouse Position"=w94:cluster{"X":i32, "Y":i32}, "X Zoom"=w95:sgl)  [unwired: 2 in, 2 out]
            n47 = Greater Than 0?(x=w100) -> (x > 0?=w99:bool)
            n48 = Select(t=1.2, s=w99, f=0.8) -> (s? t:f=w96:dbl)
            n49 = Multiply(x=w96, y=w95) -> (x*y=w93:dbl)
            n50 = property on="Image" class="ImageControl"("X Zoom"=w93, "Y Zoom"=w93, "Image Center Position"=w94) -> ()  [unwired: 2 in, 2 out]
            n51 = call <vilib>:"Add State(s) to Queue__JKI_lib_State_Machine.vi"("State(s) in (\"\")"=w104) -> ("States Out"=w103:string)  [unwired: 14 in]
          }
          event "Image": Mouse Up {
            n52 = event-data() -> ()  [unwired: 1 in, 1 out]
            n53 = property on="Image" class="ImageControl"() -> ("Last Mouse Position"=w110:cluster{"X":i32, "Y":i32})  [unwired: 2 in, 2 out]
            n54 = local read "Temps"() -> (w105:dbl[][])
            n55 = local read "Points"() -> (w109:T2[])
            n56 = call "SingleWellUpdater.vi"("Temps"=w105, "Well Coordinates"=w109, "Last Mouse Position"=w110) -> ("Well idx"=w106:i32, "ROI Descriptor"=w107:T9, "State out"=w108:string)  [unwired: 6 in]
            n57 = property on="Image" class="ImageControl"("ROI"=w107) -> ()  [unwired: 2 in, 2 out]
            n58 = local write "Well"(w106) -> ()
            n59 = call <vilib>:"Add State(s) to Queue__JKI_lib_State_Machine.vi"("State(s) in Front (\"\")"=w108, "State(s) in (\"\")"=w114) -> ("States Out"=w113:string)  [unwired: 13 in]
          }
          event Panel Close? {
            # "Discard the event because we'll close the front panel ourselves in Macro: Exit"
            # "Close Panel button (pressed) Event\n(this executes Macro: Exit to terminate the VI)"
            n60 = event-data() -> ()  [unwired: 1 in, 1 out]
            n61 = call <vilib>:"Add State(s) to Queue__JKI_lib_State_Machine.vi"("State(s) in Front (\"\")"="Macro: Exit", "State(s) in (\"\")"=w120) -> ("States Out"=w119:string)  [unwired: 13 in]
            n62 = event-data("Discard?"=TRUE) -> ()  [unwired: 1 in, 1 out]
          }
          event "Temps single": Cursor Move {
            w122 = 0 ("lower limit")
            n63 = event-data() -> ()  [unwired: 1 in, 9 out]
            n64 = property on="Temps single" class="WFGraph (strict)"() -> ("Cursor.Cursor X"=w124:dbl)  [unwired: 2 in, 2 out]
            n65 = local read "maxSize"() -> (w123:i32)
            n66 = In Range and Coerce(upper limit=w123, x=w124, lower limit=w122) -> (coerced(x)=w121:dbl)  [unwired: 1 out]
            n67 = local write "ImageIdx"(w121) -> ()
            n68 = property on="Temps single" class="WFGraph (strict)"("XScale.Maximum"=w123, "XScale.Minimum"=w122) -> ()  [unwired: 2 in, 2 out]
            n69 = property on="Temps single" class="WFGraph (strict)"("Cursor.Cursor X"=w121) -> ()  [unwired: 2 in, 2 out]
            n70 = property on="Temps" class="WFGraph (strict)"("Cursor.Cursor X"=w121) -> ()  [unwired: 2 in, 2 out]
            n71 = property on="Temps grads" class="WFGraph (strict)"("Cursor.Cursor X"=w121) -> ()  [unwired: 2 in, 2 out]
            n72 = property on="Temps single grad" class="WFGraph (strict)"("Cursor.Cursor X"=w121) -> ()  [unwired: 2 in, 2 out]
            n73 = call <vilib>:"Add State(s) to Queue__JKI_lib_State_Machine.vi"("State(s) in Front (\"\")"="Data: Set Image\nData: Show Img\nData: Update Well Temp", "State(s) in (\"\")"=w129) -> ("States Out"=w128:string)  [unwired: 13 in]
          }
          event "Temps": Cursor Move {
            w132 = 0 ("lower limit")
            n74 = event-data() -> ()  [unwired: 1 in, 1 out]
            n75 = property on="Temps" class="WFGraph (strict)"() -> ("Cursor.Cursor X"=w133:dbl)  [unwired: 2 in, 2 out]
            n76 = local read "maxSize"() -> (w131:i32)
            n77 = In Range and Coerce(upper limit=w131, x=w133, lower limit=w132) -> (coerced(x)=w130:dbl)  [unwired: 1 out]
            n78 = property on="Temps" class="WFGraph (strict)"("Cursor.Cursor X"=w130, "XScale.Maximum"=w131, "XScale.Minimum"=w132) -> ()  [unwired: 2 in, 2 out]
            n79 = local write "ImageIdx"(w130) -> ()
            n80 = property on="Temps single" class="WFGraph (strict)"("Cursor.Cursor X"=w130) -> ()  [unwired: 2 in, 2 out]
            n81 = property on="Temps grads" class="WFGraph (strict)"("Cursor.Cursor X"=w130) -> ()  [unwired: 2 in, 2 out]
            n82 = property on="Temps single grad" class="WFGraph (strict)"("Cursor.Cursor X"=w130) -> ()  [unwired: 2 in, 2 out]
            n83 = call <vilib>:"Add State(s) to Queue__JKI_lib_State_Machine.vi"("State(s) in Front (\"\")"="Data: Set Image\nData: Show Img\nData: Update Well Temp", "State(s) in (\"\")"=w138) -> ("States Out"=w137:string)  [unwired: 13 in]
          }
          event "Temps single grad": Cursor Move {
            w140 = 0 ("lower limit")
            n84 = event-data() -> ()  [unwired: 1 in, 1 out]
            n85 = property on="Temps single grad" class="WFGraph (strict)"() -> ("Cursor.Cursor X"=w141:dbl)  [unwired: 2 in, 2 out]
            n86 = local read "maxSize"() -> (w139:i32)
            n87 = In Range and Coerce(upper limit=w139, x=w141, lower limit=w140) -> (coerced(x)=w142:dbl)  [unwired: 1 out]
            n88 = property on="Temps" class="WFGraph (strict)"("Cursor.Cursor X"=w142, "XScale.Maximum"=w139, "XScale.Minimum"=w140) -> ()  [unwired: 2 in, 2 out]
            n89 = local write "ImageIdx"(w142) -> ()
            n90 = property on="Temps single" class="WFGraph (strict)"("Cursor.Cursor X"=w142) -> ()  [unwired: 2 in, 2 out]
            n91 = property on="Temps single grad" class="WFGraph (strict)"("Cursor.Cursor X"=w142, "XScale.Maximum"=w139, "XScale.Minimum"=w140) -> ()  [unwired: 2 in, 2 out]
            n92 = property on="Temps grads" class="WFGraph (strict)"("Cursor.Cursor X"=w142) -> ()  [unwired: 2 in, 2 out]
            n93 = call <vilib>:"Add State(s) to Queue__JKI_lib_State_Machine.vi"("State(s) in Front (\"\")"="Data: Set Image\nData: Show Img\nData: Update Well Temp", "State(s) in (\"\")"=w147) -> ("States Out"=w146:string)  [unwired: 13 in]
          }
          event "Temps grads": Value Change {
            w148 = 0 ("lower limit")
            n94 = event-data() -> ()  [unwired: 1 in, 6 out]
            n95 = property on="Temps grads" class="WFGraph (strict)"() -> ("Cursor.Cursor X"=w150:dbl)  [unwired: 2 in, 2 out]
            n96 = local read "maxSize"() -> (w149:i32)
            n97 = In Range and Coerce(upper limit=w149, x=w150, lower limit=w148) -> (coerced(x)=w151:dbl)  [unwired: 1 out]
            n98 = property on="Temps" class="WFGraph (strict)"("Cursor.Cursor X"=w151, "XScale.Maximum"=w149, "XScale.Minimum"=w148) -> ()  [unwired: 2 in, 2 out]
            n99 = local write "ImageIdx"(w151) -> ()
            n100 = property on="Temps single" class="WFGraph (strict)"("Cursor.Cursor X"=w151) -> ()  [unwired: 2 in, 2 out]
            n101 = property on="Temps grads" class="WFGraph (strict)"("XScale.Maximum"=w149, "XScale.Minimum"=w148, "Cursor.Cursor X"=w151) -> ()  [unwired: 2 in, 2 out]
            n102 = property on="Temps single grad" class="WFGraph (strict)"("Cursor.Cursor X"=w151, "XScale.Maximum"=w149, "XScale.Minimum"=w148) -> ()  [unwired: 2 in, 2 out]
            n103 = call <vilib>:"Add State(s) to Queue__JKI_lib_State_Machine.vi"("State(s) in Front (\"\")"="Data: Set Image\nData: Show Img\nData: Update Well Temp", "State(s) in (\"\")"=w156) -> ("States Out"=w155:string)  [unwired: 13 in]
          }
          event "Calc_All": Value Change {
            w159 = FALSE ("Visible")
            w158 = TRUE ("Visible")
            w161 = u8 0 ("Slide")
            n104 = event-data() -> ()  [unwired: 1 in, 6 out]
            n105 = local write "ImageIdx"(w161) -> ()
            n106 = local write "Slide"(w161) -> ()
            n107 = local write "img"(0 ("img")) -> ()
            n108 = property on="Temps" class="WFGraph (strict)"("Visible"=w158) -> ()  [unwired: 2 in, 2 out]
            n109 = property on="Graph2 grad" class="WFGraph (strict)"("Visible"=w158) -> ()  [unwired: 2 in, 2 out]
            n110 = property on="Temps single" class="WFGraph (strict)"("Visible"=w159) -> ()  [unwired: 2 in, 2 out]
            n111 = property on="Temps single grad" class="WFGraph (strict)"("Visible"=w159) -> ()  [unwired: 2 in, 2 out]
            n112 = local write "Offset Applied?"(FALSE ("Offset Applied?")) -> ()
            n113 = call <vilib>:"Add State(s) to Queue__JKI_lib_State_Machine.vi"("State(s) in Front (\"\")"="Data: Temps Clear\nData: Set Image\nUI: Cursor Set >> Busy\nUI: Progress >> Show\nImage: Calculate All Temps\nImage: Calculate Gradients\nImage: Calculate Freezing Points\nImage: Calculate Offset\nUI: Progress >> Hide\nUI: Cursor Set >> Idle\nUI: Tutorial >> Click on a Well to show single or click outside the plate to show all.", "State(s) in (\"\")"=w166) -> ("States Out"=w165:string)  [unwired: 13 in]
          }
          event "Correct Data": Value Change {
            n114 = event-data() -> ()  [unwired: 1 in, 6 out]
            n115 = property on="Correct Data" class="Bool"("Visible"=FALSE) -> ()  [unwired: 2 in, 2 out]
            n116 = property on="Remove_Correction" class="Bool"("Visible"=TRUE) -> ()  [unwired: 2 in, 2 out]
            n117 = call <vilib>:"Add State(s) to Queue__JKI_lib_State_Machine.vi"("State(s) in Front (\"\")"="UI: Cursor Set >> Busy\nUI: Tutorial >> Correcting Data\nImage: Correct Offset\nImage: Calculate Gradients\nImage: Calculate Freezing Points\nImage: Update Focus Well\nUI: Tutorial >> Done\nUI: Cursor Set >> Idle", "State(s) in (\"\")"=w174) -> ("States Out"=w173:string)  [unwired: 13 in]
            "Offset Applied?" <- TRUE ("Offset Applied?")
          }
          event "Remove_Correction": Value Change {
            n118 = event-data() -> ()  [unwired: 1 in, 6 out]
            n119 = property on="Remove_Correction" class="Bool"("Visible"=FALSE) -> ()  [unwired: 2 in, 2 out]
            n120 = property on="Correct Data" class="Bool"("Visible"=TRUE) -> ()  [unwired: 2 in, 2 out]
            n121 = local write "Offset Applied?"(FALSE ("Offset Applied?")) -> ()
            n122 = call <vilib>:"Add State(s) to Queue__JKI_lib_State_Machine.vi"("State(s) in Front (\"\")"="UI: Cursor Set >> Busy\nUI: Tutorial >> Correcting Data\nImage: Remove Offset\nImage: Calculate Gradients\nImage: Calculate Freezing Points\nImage: Update Focus Well\nUI: Tutorial >> Done\nUI: Cursor Set >> Idle", "State(s) in (\"\")"=w182) -> ("States Out"=w181:string)  [unwired: 13 in]
          }
        }
      }
      frame "---------- Core ----------" {
        # "Do not put any code in this frame.\n(it is a separator no-op)"
        n123 = call <vilib>:"Add State(s) to Queue__JKI_lib_State_Machine.vi"("State(s) in (\"\")"=w186) -> ("States Out"=w185:string)  [unwired: 14 in]
      }
      frame Default {
        w196 = 42 items=["No error", "Argument error", "Memory is full", "Out of zone", "End of file", "File already open", "Generic file I/O error", "File not found", "File permission error", "Disk is full", "Duplicate path", "Too many files open", "System feature not enabled", "Resource file not found", "Cannot add resource", "Resource not found", "Image not found", "Image memory error", "Pen does not exist", "Config type invalid", "Config token not found", "Config parse error", "Config memory error", "Bad external code format", "Bad external code offset", "External code not present", "Null window", "Destroy window error", "Null menu", "Print aborted", "Bad print record", "Print driver error", "Windows error during printing", "Memory error during printing", "Print dialog error", "Generic print error", "Invalid device refnum", "Device not found", "Device parameter error", "Device unit error", "Cannot open device", "Device call aborted", "Generic error", "Cancelled by user", "Object ID too low", "Object ID too high", "Object not in heap", "Unknown heap", "Unknown object (invalid DefProc)", "Unknown object (DefProc not in table)", "Message out of range", "Invalid (null) method", "Unknown message", "Manager call not supported", "Bad address", "Network operation in progress", "Network operation timed out", "Connection is busy", "Network attribute not supported", "Network error", "Address in use", "System out of memory", "Connection aborted", "Connection refused", "Not connected", "Already connected", "Connection closed", "Initialization error (interapplication manager)", "Bad occurrence", "Wait on unbound occurrence handler", "Occurrence queue overflow", "Datalog type conflict", "Unused", "Unrecognized type (interapplication manager)", "Memory corrupt", "Failed to make temporary DLL", "Old CIN version", "Drag socket not found", "Failed to load drop-object", "Failed to register OLE object", "Failed to release OLE object", "Format specifier type mismatch", "Unknown format specifier", "Too few format specifiers", "Too many format specifiers", "Scan failed", "Newer CIN version", "Error converting to variant", "Runtime menu error", "Password tampered", "Variant attribute not found", "Incompatible variant data type", "Event data is not available", "Event Store is not present", "Occurrence is not found", "Event Queue is not created", "Event info is not available", "Refnum passed is NULL", "Error retrieving Class GUID", "Error retrieving CoClass GUID", "Error retrieving TypeLib GUID.", "Bad built application magic bytes.", "Specific driver is different from the specific driver associated with the Logical Name.", "There is no session opened to the class driver.", "Max Error", "MAX - Error with config objects", "MAX - Error loading configuration", "MAX - Group not supported"]
        # "Current State"
        # "Do not delete, rename, or modify this frame.\n(this is used to capture unhandled states and typos)"
        # "Handle mistyped state name (developer tool)"
        n124 = Format Into String(format string="Software Exception: Unhandled State \"%s\"." ("message"), error in=w192, w187) -> (resulting string=w195:string, error out=w194:errorcluster)  [unwired: 1 in]
        n125 = call <vilib>:"Error Cluster From Error Code.vi"("show call chain? (False)"=TRUE, "error in (no error)"=w194, "error message (\"\")"=w195, "error code (0)"=w196) -> ("error out"=w193:errorcluster)  [unwired: 5 in]
        n126 = call <vilib>:"Add State(s) to Queue__JKI_lib_State_Machine.vi"("State(s) in (\"\")"=w191) -> ("States Out"=w190:string)  [unwired: 14 in]
      }
      frame "Initialize Core Data" {
        # "Do not delete, rename, or modify this frame.\n(this is used to determine panel behavior on exit)"
        # "originally closed?"
        # "exe?"
        # "If panel starts closed or is an EXE, then close it when we exit"
        n127 = property class="App"() -> ("App.Kind"=w206:T4)  [unwired: 2 in, 2 out]
        n128 = control-ref of="Current VI Reference"() -> (w201:refnum<vi>)
        n129 = property class="VI"() -> ("FP.State"=w200:T3)  [unwired: 2 in, 2 out]
        n130 = Equal?(x=w200, y=T3."Closed" ("Front Panel Window:State")) -> (x = y?=w198:bool)
        n131 = Equal?(x=w206, y=T4."Run Time System" ("Application:Kind")) -> (x = y?=w204:bool)
        n132 = Or(x=w198, y=w204) -> (x .or. y?=w202:bool)
        n133 = Bundle By Name(cluster=w203, "Core.Current VI Reference"=w201, "Core.Close Panel on Exit?"=w202) -> (w208:T6)
        n134 = call <vilib>:"Add State(s) to Queue__JKI_lib_State_Machine.vi"("State(s) in (\"\")"=w210) -> ("States Out"=w209:string)  [unwired: 14 in]
      }
      frame "Error Handler" {
        # "Unhandled Error -- Display it"
        # "Handle any errors here.\nYou can also output any states to clean-up after errors occur"
        # "Clear error"
        n135 = call <vilib>:"General Error Handler.vi"("error in (no error)"=w212) -> ()  [unwired: 10 in, 5 out]
        n136 = call <vilib>:"Add State(s) to Queue__JKI_lib_State_Machine.vi"("State(s) in Front (\"\")"="/* Post Error States", "State(s) in (\"\")"=w216) -> ("States Out"=w215:string)  [unwired: 13 in]
      }
      frame "Exit" {
        # "Do not put any code in this frame.\n(No errors that occur here will be handled.)"
        n137 = call <vilib>:"Add State(s) to Queue__JKI_lib_State_Machine.vi"("State(s) in (\"\")"=w221) -> ("States Out"=w220:string)  [unwired: 14 in]
      }
      frame "---------- Data ----------" {
        # "Do not put any code in this frame.\n(It is a separator no-op. You can make a copy of this frame to create a new Data frame)"
        n138 = call <vilib>:"Add State(s) to Queue__JKI_lib_State_Machine.vi"("State(s) in (\"\")"=w225) -> ("States Out"=w224:string)  [unwired: 14 in]
      }
      frame "Data: Load Image" {
        # "Do not put any code in this frame.\n(It is a separator no-op. You can make a copy of this frame to create a new Data frame)"
        n139 = local write "Slide"(u8 0 ("Slide")) -> ()
        n140 = local write "img"(0 ("img")) -> ()
        n141 = Empty String/Path?(string/path="Path") -> (empty?=w235:bool)
        n142 = case shown="False" w235 {
          tunnel: [w260 _] -> w238
          tunnel: w237 -> [w255 w290]
          tunnel: [w261 w290] -> w231
          tunnel: "Path" -> [w244 _]
          tunnel: [w257 _] -> w233
          tunnel: w228 -> [w246 _]
          frame False {
            w249 = 0.0 ("X Scale.Range:Minimum")
            w251 = 40.0 ("Y Scale.Range:Maximum")
            w250 = -45.0 ("X Scale.Range:Minimum")
            n143 = Build Path(base path=w244, name or relative path=path "Images") -> (appended path=w247:path)
            n144 = List Folder(path=w247) -> (filenames=w258:string[])  [unwired: 3 in, 3 out]
            n145 = property on="Slide" class="Slide (strict)"(error in=w255, "Visible"=TRUE) -> (error out=w254:errorcluster)  [unwired: 1 in, 1 out]
            n146 = call "Partition_Extract.vi"("input cluster"=w246, "Path"=w244) -> ("PartitionArray"=→"PartitionArray":string[])
            n147 = call "Thermistor_Extract.vi"("Path"=w244) -> ("ThermTemps"=→"ThermTemps":dbl[])
            n148 = Array Size(array=w258) -> (size(s)=w253:i32)
            n149 = Format Into String(w253) -> (resulting string=w252:string)  [unwired: 3 in, 1 out]
            n150 = for {
              tunnel: [w289] -> w263
              tunnel: [w273] -> w257 mode=indexing
              tunnel: [w276] -> _ mode=indexing
              tunnel: w258 -> [w281] mode=indexing
              tunnel: w247 -> [w280]
              tunnel: w253 -> [w275]
              tunnel: w254 -> [w276]
              workers-P: _ -> [_]
              tunnel: w252 -> [w265]
              i -> [w274]
              w284 = T10 7 items=["Grayscale (U8)", "Grayscale (I16)", "Grayscale (SGL)", "Complex (CSG)", "RGB (U32)", "HSL (U32)", "RGB (U64)", "Grayscale (U16)"] ("Image Type")
              n151 = Format Into String(w274) -> (resulting string=w282:string)  [unwired: 3 in, 1 out]
              n152 = local read "img"() -> (w272:i32)
              n153 = Concatenate Strings("img_" ("Image Name"), w282) -> (w283:string)
              n154 = Build Path(base path=w280, name or relative path=w281) -> (appended path=w279:path)
              n155 = Increment(x=w272) -> (x+1=w266:i32)
              n156 = call "IMAQ Create"("Image Name"=w283, "Image Type"=w284, "error in (no error)"=w276) -> ("New Image"=w287:T1, "error out"=w288:errorcluster)  [unwired: 2 in]
              n157 = Format Into String(w266) -> (resulting string=w269:string)  [unwired: 3 in, 1 out]
              n158 = local write "img"(w266) -> ()
              n159 = call "IMAQ ReadFile 2"("File Path"=w279, "error in (no error)"=w288, "Image"=w287) -> ("error out"=w286:errorcluster, "Image Out"=w264:T1)  [unwired: 4 in, 3 out]
              n160 = Divide(x=w266, y=w275) -> (x/y=w278:dbl)
              n161 = Concatenate Strings("Loading image " ("Tutorial"), w269, " of " ("Tutorial"), w265) -> (w270:string)
              n162 = Multiply(x=w278, y=100.0) -> (x*y=→"Slide":dbl)
              n163 = local write "Tutorial"(w270) -> ()
              n164 = call "IMAQ Clear Overlay"("error in (no error)"=w286, "Image"=w264) -> ("error out"=w289:errorcluster, "Image Out"=w273:T1)  [unwired: 8 in]
              n165 = local write "Image"(w273) -> ()
            }
            n166 = Decrement(x=w253) -> (x-1=w242:i32)
            "maxSize" <- w242
            n167 = property on="ImageIdx" class="Slide (strict)"("Scale.Maximum"=w242, "Scale.Minimum"=0.0 ("Scale.Range:Minimum")) -> ()  [unwired: 2 in, 2 out]
            n168 = property on="Temps single grad" class="WFGraph (strict)"("XScale.Maximum"=w242) -> ()  [unwired: 2 in, 2 out]
            n169 = property on="Temps grads" class="WFGraph (strict)"("XScale.Maximum"=w242) -> ()  [unwired: 2 in, 2 out]
            n170 = property on="Temps single" class="WFGraph (strict)"("XScale.Maximum"=w242, "XScale.Minimum"=w249, "YScale.Maximum"=w251, "YScale.Minimum"=w250) -> ()  [unwired: 2 in, 2 out]
            n171 = property on="Temps" class="WFGraph (strict)"("XScale.Maximum"=w242, "XScale.Minimum"=w249, "YScale.Maximum"=w251, "YScale.Minimum"=w250) -> ()  [unwired: 2 in, 2 out]
            n172 = Index Array(array=w257) -> (element=w260:T1)  [unwired: 1 in]
            "Image" <- w260
            n173 = property on="Image" class="ImageControl"(error in=w263, "ROI"=T5 {"Global Rectangle"=[], "Contours"=[]}) -> (error out=w261:errorcluster)  [unwired: 1 in, 1 out]
          }
          frame True {
            (unwired) FALSE ("Visible")
          }
        }
        n174 = property on="Slide" class="Slide (strict)"(error in=w231, "Visible"=FALSE) -> (error out=w230:errorcluster)  [unwired: 1 in, 1 out]
        n175 = Bundle By Name(cluster=w228, "Image Out"=w238, "img_array"=w233) -> (w239:T6)
        n176 = local write "ImageIdx"(u32 0 ("Image")) -> ()
        n177 = call <vilib>:"Add State(s) to Queue__JKI_lib_State_Machine.vi"("State(s) in Front (\"\")"="Image: Draw" ("State(s) in Front (\"\")"), "State(s) in (\"\")"=w241) -> ("States Out"=w240:string)  [unwired: 13 in]
      }
      frame "Data: Set Image" {
        # "Do not put any code in this frame.\n(It is a separator no-op. You can make a copy of this frame to create a new Data frame)"
        n178 = Unbundle By Name(w295) -> ("img_array"=w294:T1[])
        n179 = Index Array(array=w294, index="ImageIdx") -> (element=w291:T1)
        n180 = Bundle By Name(cluster=w295, "Image Out"=w291) -> (w296:T6)
        n181 = call <vilib>:"Add State(s) to Queue__JKI_lib_State_Machine.vi"("State(s) in (\"\")"=w298) -> ("States Out"=w297:string)  [unwired: 14 in]
      }
      frame "Data: Load Results" {
        # "Do not put any code in this frame.\n(It is a separator no-op. You can make a copy of this frame to create a new Data frame)"
        n182 = local read "Path"() -> (w301:path)
        n183 = Build Path(base path=w301, name or relative path=path "Result Data.csv") -> (appended path=w302:path)
        n184 = call <vilib>:"Check if File or Folder Exists.vi"("path"=w302) -> ("file or folder exists?"=w304:bool, "dup path"=w303:path)  [unwired: 8 in, 1 out]
        n185 = case shown="True" w304 {
          tunnel: w303 -> [_ w317]
          tunnel: ["" ("State(s) in Front (\"\")") "UI: Single Temps >> Hide" ("State(s) in Front (\"\")")] -> w299
          frame False {
          }
          frame True {
            n186 = call-poly <vilib>:"Read Delimited Spreadsheet.vi"("file path (dialog if empty)"=w317, "delimiter (\\t)"=";" ("delimiter (\\t)")) -> ("all rows"=w316:string[][])  [unwired: 8 in, 5 out]
            n187 = call <vilib>:"Application Directory.vi"() -> ("Application Directory"=w319:path)
            n188 = Path To String(path=w317) -> (string=w324:string)
            n189 = call "DataArray_Reformatter.vi"("Data Array"=w316) -> ("Temps"=w314:dbl[][], "FreezeTemps"=w315:dbl[], "Offsets"=w312:dbl[], "Offset Applied"=w311:bool)
            n190 = Build Path(base path=w319, name or relative path=path "TCEM.ini" ("file path (dialog if empty)")) -> (appended path=w320:path)
            n191 = Build Array(w324) -> (w323:string[])
            n192 = Not(x=w311) -> (.not. x?=w310:bool)
            n193 = local write "Offsets"(w312) -> ()
            n194 = local write "Offset Applied?"(w311) -> ()
            n195 = property on="Remove_Correction" class="Bool"("Visible"=w311) -> ()  [unwired: 2 in, 2 out]
            n196 = local write "FreezeTemps"(w315) -> ()
            n197 = local write "Temps"(w314) -> ()
            n198 = call-poly <vilib>:"Write Delimited Spreadsheet.vi"("file path (dialog if empty)"=w320, "1D data"=w323, "append to file? (new file:F)"=TRUE) -> ()  [unwired: 11 in, 2 out]
            n199 = property on="Correct Data" class="Bool"("Visible"=w310) -> ()  [unwired: 2 in, 2 out]
          }
        }
        n200 = call <vilib>:"Add State(s) to Queue__JKI_lib_State_Machine.vi"("State(s) in Front (\"\")"=w299, "State(s) in (\"\")"=w308) -> ("States Out"=w307:string)  [unwired: 13 in]
      }
      frame "Data: Load Calibration" {
        # "Do not put any code in this frame.\n(It is a separator no-op. You can make a copy of this frame to create a new Data frame)"
        n201 = local read "Path"() -> (w326:path)
        n202 = Build Path(base path=w326, name or relative path=path "TCC.cal") -> (appended path=w331:path)
        n203 = call <vilib>:"Check if File or Folder Exists.vi"("path"=w331) -> ("file or folder exists?"=w332:bool, "dup path"=w329:path)  [unwired: 8 in, 1 out]
        n204 = case shown="True" w332 {
          tunnel: w329 -> [_ w357]
          tunnel: w328 -> [w337 w356]
          tunnel: [w338 w355] -> w327
          tunnel: w326 -> [w341 _]
          tunnel: [w336 "Image: Draw\nData: Load Results\nData: Set Image\nImage: Calculate Gradients\nImage: Calculate Freezing Points\nUI: Calc >> True\nUI: Menu Overlay Grid >> True\nUI: Menu Overlay Temps >> True\nUI: Progress >> Hide\nUI: Cursor Set >> Idle\nUI: Tutorial >> Click on a Well to show single or click outside the plate to show all."] -> w325
          frame False {
            n205 = call "CalibrationLoadPrompt.vi"("Root Path"=w341) -> ("cancel?"=w339:bool, "selected path"=w340:path)  [unwired: 9 in]
            n206 = case shown="False" w339 {
              tunnel: w340 -> [w345 _]
              tunnel: [w343 w350] -> w338
              tunnel: w337 -> [w344 w350]
              tunnel: ["Image: Draw\nData: Load Results\nData: Set Image\nImage: Calculate Gradients\nImage: Calculate Freezing Points\nUI: Menu Overlay Grid >> True\nUI: Menu Overlay Temps >> True\nUI: Calc >> True\nUI: Progress >> Hide\nUI: Cursor Set >> Idle\nUI: Tutorial >> Click on a Well to show single or click outside the plate to show all." "UI: Calc >> Disable\nUI: Progress >> Hide\nUI: Cursor Set >> Idle\nUI: Tutorial >> Error: Missing Calibration File!"] -> w336
              frame False {
                n207 = call "TCam_Calibration_LoadSettings.vi"("path"=w345) -> ("Fixpoint Area"=w346:dbl, "Scan Area"=w347:dbl, "Points"=w348:T11)  [unwired: 7 in, 1 out]
                n208 = Bundle By Name(cluster=w344, "Points"=w348, "Scan Area"=w347, "Fixpoint Area"=w346) -> (w343:T6)
              }
              frame True {
              }
            }
          }
          frame True {
            n209 = call "TCam_Calibration_LoadSettings.vi"("path"=w357) -> ("Fixpoint Area"=w352:dbl, "Scan Area"=w353:dbl, "Points"=w354:T11)  [unwired: 7 in, 1 out]
            n210 = Bundle By Name(cluster=w356, "Points"=w354, "Scan Area"=w353, "Fixpoint Area"=w352) -> (w355:T6)
          }
        }
        n211 = call <vilib>:"Add State(s) to Queue__JKI_lib_State_Machine.vi"("State(s) in Front (\"\")"=w325, "State(s) in (\"\")"=w335) -> ("States Out"=w334:string)  [unwired: 13 in]
      }
      frame "Data: Show Img" {
        # "Do not put any code in this frame.\n(It is a separator no-op. You can make a copy of this frame to create a new Data frame)"
        n212 = Unbundle By Name(w358) -> ("Image Out"=w359:T1)
        n213 = local write "Image"(w359) -> ()
        n214 = call <vilib>:"Add State(s) to Queue__JKI_lib_State_Machine.vi"("State(s) in (\"\")"=w362) -> ("States Out"=w361:string)  [unwired: 14 in]
      }
      frame "Data: Initialize" {
        w364 = dbl[] [] ("Offsets")
        w365 = dbl[][] []  # Temps_Array
        w366 = dbl[] []  # Temps
        w369 = T1[] []  # img_array
        w371 = u32 1 items=["Zoom Tool"=8, "Selection Tool"=0, "Pan Tool"=9, "Point Tool"=1, "Line Tool"=2, "Rectangle Tool"=3, "Rotated Rectangle Tool"=12, "Polyline Tool"=10, "Polygon Tool"=5, "Freehand Tool"=11, "Closed Freehand Tool"=6, "Ellipse Tool"=4, "Annulus Tool"=7] ("Current ROI Tool")
        w368 = 0  # State
        w372 = T12 {"Current VI Reference"=refnum, "Close Panel on Exit?"=FALSE}  # Core
        # "Initialize the shift-register data, here.\n(data names are defined by what you wire into the bundle function)"
        n215 = property on="Image" class="ImageControl"("Current ROI Tool"=w371) -> ()  [unwired: 2 in, 2 out]
        n216 = local write "Offsets"(w364) -> ()
        n217 = local write "ThermTemps"(w364) -> ()
        n218 = local write "Slide"(w368) -> ()
        n219 = Bundle By Name(cluster=T6 {"Core"={"Current VI Reference"=refnum, "Close Panel on Exit?"=FALSE}, "Image Out"=refnum, "State"=0, "Points"={"Top Left"={"X"=0.0, "Y"=0.0}, "Top Right"={"X"=0.0, "Y"=0.0}, "Bottom Left"={"X"=0.0, "Y"=0.0}, "Bottom Right"={"X"=0.0, "Y"=0.0}, "x space 2"=0.0, "y space 2"=0.0, "x_space"=0.0, "y_space"=0.0, "Pixels"=[], "Fixpoint"={"X"=0.0, "Y"=0.0}}, "img_array"=[], "Temps"=[], "Temps_Array"=[], "Scan Area"=0.0, "Fixpoint Area"=0.0, "PCR Size"=0} ("Cluster"), "Core"=w372, "Image Out"=T1 refnum, "State"=w368, "img_array"=w369, "Temps"=w366, "Temps_Array"=w365) -> (w373:T6)
        n220 = call <vilib>:"Add State(s) to Queue__JKI_lib_State_Machine.vi"("State(s) in (\"\")"=w375) -> ("States Out"=w374:string)  [unwired: 14 in]
      }
      frame "Data: Temps Clear" {
        w376 = dbl[][] [] ("Temps_Array")
        w377 = dbl[] []  # Temps
        # "Initialize the shift-register data, here.\n(data names are defined by what you wire into the bundle function)"
        n221 = local write "Temps single"(w377) -> ()
        n222 = local write "Temps grads"(w376) -> ()
        n223 = local write "Temps"(w376) -> ()
        n224 = local write "Temps single grad"(w377) -> ()
        n225 = Bundle By Name(cluster=w379, "Temps"=w377, "Temps_Array"=w376) -> (w378:T6)
        n226 = call <vilib>:"Add State(s) to Queue__JKI_lib_State_Machine.vi"("State(s) in (\"\")"=w382) -> ("States Out"=w381:string)  [unwired: 14 in]
      }
      frame "Data: Update Well Temp" {
        # "Initialize the shift-register data, here.\n(data names are defined by what you wire into the bundle function)"
        n227 = local read "Temps single"() -> (w384:dbl[])
        n228 = local read "ImageIdx"() -> (w385:u32)
        n229 = Index Array(array=w384, index=w385) -> (element=w383:dbl)
        n230 = local write "CurTemp"(w383) -> ()
        n231 = call <vilib>:"Add State(s) to Queue__JKI_lib_State_Machine.vi"("State(s) in (\"\")"=w389) -> ("States Out"=w388:string)  [unwired: 14 in]
      }
      frame "Data: Save Results" {
        # "Initialize the shift-register data, here.\n(data names are defined by what you wire into the bundle function)"
        n232 = local read "Path"() -> (w396:path)
        n233 = local read "Offsets"() -> (w391:dbl[])
        n234 = local read "FreezeTemps"() -> (w390:dbl[])
        n235 = Build Path(base path=w396, name or relative path=path "Result Data.csv") -> (appended path=w393:path)
        n236 = local read "PartitionArray"() -> (w403:string[])
        n237 = local read "Temps"() -> (w402:dbl[][])
        n238 = call <vilib>:"Check if File or Folder Exists.vi"("path"=w393) -> ("file or folder exists?"=w397:bool, "dup path"=w392:path)  [unwired: 8 in, 1 out]
        n239 = case shown="True" w397 {
          selector: w397 -> [_ w411]
          tunnel: w396 -> [w409 _]
          tunnel: [w408 w410] -> w395
          tunnel: [w407 w411] -> w394
          tunnel: w392 -> [_ w410]
          frame False {
            n240 = call "ResultSavePrompt.vi"("Path"=w409) -> ("selected path"=w408:path, "cancel?"=w407:bool)
          }
          frame True {
          }
        }
        n241 = call "DataArray_Formatter.vi"("Temps"=w402, "input cluster"=w404, "FreezeTemps"=w390, "Offsets"=w391, "PartitionArray"=w403) -> ("Data Array"=w401:string[][])  [unwired: 1 in]
        n242 = case shown="True" w394 {
          tunnel: w401 -> [_ w421]
          tunnel: w400 -> [_ w419]
          tunnel: w395 -> [_ w418]
          frame False {
          }
          frame True {
            n243 = call-poly <vilib>:"Write Delimited Spreadsheet.vi"("file path (dialog if empty)"=w418, "2D data"=w421, "error in (no error)"=w419, "delimiter (\\t)"=";" ("delimiter (\\t)")) -> ()  [unwired: 10 in, 2 out]
            n244 = call <vilib>:"Application Directory.vi"() -> ("Application Directory"=w412:path)
            n245 = Path To String(path=w418) -> (string=w417:string)
            n246 = Build Path(base path=w412, name or relative path=path "TCEM.ini" ("file path (dialog if empty)")) -> (appended path=w413:path)
            n247 = Build Array(w417) -> (w416:string[])
            n248 = call-poly <vilib>:"Write Delimited Spreadsheet.vi"("file path (dialog if empty)"=w413, "1D data"=w416, "append to file? (new file:F)"=TRUE) -> ()  [unwired: 11 in, 2 out]
          }
        }
        n249 = call <vilib>:"Add State(s) to Queue__JKI_lib_State_Machine.vi"("State(s) in Front (\"\")"="UI: Recent Menu Update" ("State(s) in Front (\"\")"), "State(s) in (\"\")"=w406) -> ("States Out"=w405:string)  [unwired: 13 in]
      }
      frame "Data: Save Results As" {
        # "Initialize the shift-register data, here.\n(data names are defined by what you wire into the bundle function)"
        n250 = local read "Offsets"() -> (w422:dbl[])
        n251 = local read "Offset Applied?"() -> (w423:bool)
        n252 = local read "FreezeTemps"() -> (w431:dbl[])
        n253 = local read "Path"() -> (w425:path)
        n254 = local read "PartitionArray"() -> (w432:string[])
        n255 = local read "Temps"() -> (w430:dbl[][])
        n256 = call "ResultSavePrompt.vi"("Path"=w425) -> ("selected path"=w427:path, "cancel?"=w426:bool)
        n257 = call "DataArray_Formatter.vi"("Temps"=w430, "input cluster"=w433, "FreezeTemps"=w431, "Offset Applied?"=w423, "Offsets"=w422, "PartitionArray"=w432) -> ("Data Array"=w429:string[][])
        n258 = case shown="False" w426 {
          tunnel: w429 -> [w445 _]
          tunnel: w428 -> [w443 _]
          tunnel: w427 -> [w442 _]
          frame False {
            n259 = call-poly <vilib>:"Write Delimited Spreadsheet.vi"("file path (dialog if empty)"=w442, "2D data"=w445, "error in (no error)"=w443, "delimiter (\\t)"=";" ("delimiter (\\t)")) -> ()  [unwired: 10 in, 2 out]
            n260 = call <vilib>:"Application Directory.vi"() -> ("Application Directory"=w436:path)
            n261 = Path To String(path=w442) -> (string=w441:string)
            n262 = Build Path(base path=w436, name or relative path=path "TCEM.ini" ("file path (dialog if empty)")) -> (appended path=w437:path)
            n263 = Build Array(w441) -> (w440:string[])
            n264 = call-poly <vilib>:"Write Delimited Spreadsheet.vi"("file path (dialog if empty)"=w437, "1D data"=w440, "append to file? (new file:F)"=TRUE) -> ()  [unwired: 11 in, 2 out]
          }
          frame True {
          }
        }
        n265 = call <vilib>:"Add State(s) to Queue__JKI_lib_State_Machine.vi"("State(s) in Front (\"\")"="UI: Recent Menu Update" ("State(s) in Front (\"\")"), "State(s) in (\"\")"=w435) -> ("States Out"=w434:string)  [unwired: 13 in]
      }
      frame "Data: Cleanup" {
        # "Cleanup any data and references, here.\n(this is called automatically, by the Macro: Exit)"
        n266 = Unbundle By Name(w451) -> ("img_array"=w449:T1[], "Image Out"=w448:T1)
        n267 = call "IMAQ Dispose"("Image"=w448, "error in (no error)"=w447) -> ("error out"=w446:errorcluster)  [unwired: 4 in]
        n268 = for {
          shift-right: [w455] -> w450
          shift-left: w446 -> [w456]
          tunnel: w449 -> [w454] mode=indexing
          n269 = call "IMAQ Dispose"("Image"=w454, "error in (no error)"=w456) -> ("error out"=w455:errorcluster)  [unwired: 4 in]
        }
        n270 = call <vilib>:"Add State(s) to Queue__JKI_lib_State_Machine.vi"("State(s) in (\"\")"=w453) -> ("States Out"=w452:string)  [unwired: 14 in]
      }
      frame "---------- UI ----------" {
        # "Do not put any code in this frame.\n(It is a separator no-op. You can make a copy of this frame to create a new UI frame)"
        n271 = call <vilib>:"Add State(s) to Queue__JKI_lib_State_Machine.vi"("State(s) in (\"\")"=w460) -> ("States Out"=w459:string)  [unwired: 14 in]
      }
      frame "UI: Initialize" {
        w472 = T10 4 items=["Grayscale (U8)", "Grayscale (I16)", "Grayscale (SGL)", "Complex (CSG)", "RGB (U32)", "HSL (U32)", "RGB (U64)", "Grayscale (U16)"] ("Image Type")
        w461 = FALSE ("Visible")
        w483 = dbl[] []
        w481 = 0.0 ("Cursor.Cursor Position:Cursor X")
        w482 = dbl[][] []
        # "Initialize the User Interface, here.\n(this is called automatically, by the Macro: Init)"
        n272 = control-ref of="Splitter 4"() -> (w463:refnum<vi>)
        n273 = local write "Offset Applied?"(FALSE ("Offset Applied?")) -> ()
        n274 = property on="Temps" class="WFGraph (strict)"("XScale.Minimum"=0.0 ("X Scale.Range:Minimum")) -> ()  [unwired: 2 in, 2 out]
        n275 = call "ShowHideSplit.vi"("Splitter in"=w463, "Show Split"=w461) -> ()  [unwired: 1 in]
        n276 = property on="Contents" class="Str"("Visible"=w461) -> ()  [unwired: 2 in, 2 out]
        n277 = property on="Image" class="ImageControl"("Zoom to Fit Mode"=TRUE) -> ()  [unwired: 2 in, 2 out]
        n278 = property on="Calc_All" class="Bool"("Visible"=w461) -> ()  [unwired: 2 in, 2 out]
        n279 = property on="CurTemp" class="DigNum (strict)"("Visible"=FALSE) -> ()  [unwired: 2 in, 2 out]
        n280 = call <vilib>:"Application Directory.vi"() -> ("Application Directory"=w476:path)
        n281 = property on="Well" class="Str"("Visible"=w461) -> ()  [unwired: 2 in, 2 out]
        n282 = call "Read Exe Version.vi"("Application name"=path "TCE.exe") -> ("FileVersion"=w468:string)  [unwired: 7 in, 3 out]
        n283 = Path To String(path=w476) -> (string=w478:string)
        n284 = property on="Remove_Correction" class="Bool"("Visible"=w461) -> ()  [unwired: 2 in, 2 out]
        n285 = Concatenate Strings("version " ("string"), w468) -> (→"version":string)
        n286 = property on="Correct Data" class="Bool"("Visible"=w461) -> ()  [unwired: 2 in, 2 out]
        n287 = call "IMAQ Create"("Image Name"="placeholder_img_TCE", "Image Type"=w472) -> ("New Image"=w475:T1)  [unwired: 3 in, 1 out]
        n288 = Concatenate Strings(w478, "\\camera_placeholder.png") -> (w477:string)
        n289 = String To Path(string=w477) -> (path=w479:path)
        n290 = call "IMAQ ReadFile 2"("Use File Path Image Type"=FALSE, "File Path"=w479, "Image"=w475) -> ("Image Out"=w470:T1)  [unwired: 4 in, 4 out]
        "placeholder image" <- w470
        n291 = local write "Image"(w470) -> ()
        n292 = local write "Path"(path "" ("Path")) -> ()
        n293 = local write "Temps single"(w483) -> ()
        n294 = local write "Temps single grad"(w483) -> ()
        n295 = local write "Temps"(w482) -> ()
        n296 = property on="Temps single" class="WFGraph (strict)"("Cursor.Cursor X"=w481) -> ()  [unwired: 2 in, 2 out]
        n297 = property on="Temps" class="WFGraph (strict)"("Cursor.Cursor X"=w481) -> ()  [unwired: 2 in, 2 out]
        n298 = local write "Temps grads"(w482) -> ()
        n299 = property on="Temps grads" class="WFGraph (strict)"("Cursor.Cursor X"=w481) -> ()  [unwired: 2 in, 2 out]
        n300 = property on="Temps single grad" class="WFGraph (strict)"("Cursor.Cursor X"=w481) -> ()  [unwired: 2 in, 2 out]
        n301 = call <vilib>:"Add State(s) to Queue__JKI_lib_State_Machine.vi"("State(s) in Front (\"\")"="UI: Tutorial\nUI: Recent Menu Update\nUI: Progress >> Hide\nUI: Menu Save >> Hide\nUI: Menu Overlay Grid >> Hide\nUI: Menu Overlay Temps >> Hide" ("State(s) in Front (\"\")"), "State(s) in (\"\")"=w492) -> ("States Out"=w491:string)  [unwired: 13 in]
        "img" <- 0
        "Title" <- "Thermal Camera Evaluation" ("Title")
        "Title 2" <- "Well Data" ("Title 2")
      }
      frame "UI: Progress" {
        # "Initialize the User Interface, here.\n(this is called automatically, by the Macro: Init)"
        n302 = case shown="\"Show\"" w496 {
          tunnel: [FALSE ("Visible") TRUE ("Visible")] -> w495
          frame "Hide", Default {
          }
          frame "Show" {
          }
        }
        n303 = local write "Slide"(u8 0 ("Slide")) -> ()
        n304 = local write "img"(0 ("img")) -> ()
        n305 = property on="Slide" class="Slide (strict)"("Visible"=w495) -> ()  [unwired: 2 in, 2 out]
        n306 = call <vilib>:"Add State(s) to Queue__JKI_lib_State_Machine.vi"("State(s) in (\"\")"=w500) -> ("States Out"=w499:string)  [unwired: 14 in]
      }
      frame "UI: Recent Menu Update" {
        # "Initialize the User Interface, here.\n(this is called automatically, by the Macro: Init)"
        n307 = Current VI's Menubar() -> (w504:refnum<k9>)
        n308 = call "RunTimeMenu_Initialize_TCE.vi"("Menu in"=w504) -> ("paths"=→"recentPaths":path[])  [unwired: 9 in, 1 out]
        n309 = call <vilib>:"Add State(s) to Queue__JKI_lib_State_Machine.vi"("State(s) in (\"\")"=w508) -> ("States Out"=w507:string)  [unwired: 14 in]
      }
      frame "UI: Show First Image" {
        w509 = 0.0 ("Cursor.Cursor Position:Cursor X")
        # "Initialize the User Interface, here.\n(this is called automatically, by the Macro: Init)"
        n310 = Unbundle By Name(w512) -> ("img_array"=w511:T1[])
        n311 = property on="Temps" class="WFGraph (strict)"("Cursor.Cursor X"=w509) -> ()  [unwired: 2 in, 2 out]
        n312 = property on="Temps grads" class="WFGraph (strict)"("Cursor.Cursor X"=w509) -> ()  [unwired: 2 in, 2 out]
        n313 = property on="Temps single grad" class="WFGraph (strict)"("Cursor.Cursor X"=w509) -> ()  [unwired: 2 in, 2 out]
        n314 = property on="Temps single" class="WFGraph (strict)"("Cursor.Cursor X"=w509) -> ()  [unwired: 2 in, 2 out]
        n315 = Index Array(array=w511) -> (element=w510:T1)  [unwired: 1 in]
        n316 = local write "Image"(w510) -> ()
        n317 = call <vilib>:"Add State(s) to Queue__JKI_lib_State_Machine.vi"("State(s) in (\"\")"=w515) -> ("States Out"=w514:string)  [unwired: 14 in]
      }
      frame "UI: Tutorial" {
        # "Initialize the User Interface, here.\n(this is called automatically, by the Macro: Init)"
        n318 = call <vilib>:"Add State(s) to Queue__JKI_lib_State_Machine.vi"("State(s) in (\"\")"=w520) -> ("States Out"=w519:string)  [unwired: 14 in]
        "Tutorial" <- w516
      }
      frame "UI: Calc" {
        # "Initialize the User Interface, here.\n(this is called automatically, by the Macro: Init)"
        n319 = case shown="\"True\"" w523 {
          tunnel: [T7."Disabled and Grayed Out" ("Disabled") T7."Disabled and Grayed Out" ("Disabled") T7."Enabled" ("Disabled")] -> w522
          tunnel: [TRUE FALSE TRUE] -> w521
          frame "Disable", "False", Default {
          }
          frame "Hidden", "Hide" {
          }
          frame "True" {
          }
        }
        n320 = property on="Calc_All" class="Bool"("DisabledEnum"=w522) -> ()  [unwired: 2 in, 2 out]
        n321 = property on="Calc_All" class="Bool"("Visible"=w521) -> ()  [unwired: 2 in, 2 out]
        n322 = call <vilib>:"Add State(s) to Queue__JKI_lib_State_Machine.vi"("State(s) in (\"\")"=w527) -> ("States Out"=w526:string)  [unwired: 14 in]
      }
      frame "UI: Cursor Set" {
        # "Argument"
        # "Set and Unset Cursor Busy.\n(Usage: \"UI: Cursor Set >> Busy|Idle\")"
        n323 = case shown="\"Busy\"" w534 {
          tunnel: w536 -> [w541 w543]
          tunnel: [w540 w542] -> w535
          frame "Idle", Default {
            n324 = call <vilib>:"Unset Busy.vi"("error in (no error)"=w541) -> ("error out"=w540:errorcluster)  [unwired: 10 in]
          }
          frame "Busy" {
            n325 = call <vilib>:"Set Busy.vi"("error in (no error)"=w543) -> ("error out"=w542:errorcluster)  [unwired: 9 in, 1 out]
          }
        }
        n326 = call <vilib>:"Add State(s) to Queue__JKI_lib_State_Machine.vi"("State(s) in (\"\")"=w539) -> ("States Out"=w538:string)  [unwired: 14 in]
      }
      frame "UI: Menu Save" {
        # "Argument"
        # "Set and Unset Cursor Busy.\n(Usage: \"UI: Cursor Set >> Busy|Idle\")"
        n327 = case shown="\"Active\", \"Show\", \"True\"" w547 {
          tunnel: [FALSE TRUE] -> w545
          frame "Disable", "False", Default {
          }
          frame "Active", "Show", "True" {
          }
        }
        n328 = Current VI's Menubar() -> (w546:refnum<k9>)
        n329 = call "RunTimeMenu_Save_State_TCE.vi"("enabled"=w545, "item tag"=string[] ["DATA_SAVE", "DATA_SAVE_AS"], "Menu in"=w546) -> ()  [unwired: 8 in, 1 out]
        n330 = call <vilib>:"Add State(s) to Queue__JKI_lib_State_Machine.vi"("State(s) in (\"\")"=w551) -> ("States Out"=w550:string)  [unwired: 14 in]
      }
      frame "UI: Menu Overlay Grid" {
        # "Argument"
        # "Set and Unset Cursor Busy.\n(Usage: \"UI: Cursor Set >> Busy|Idle\")"
        n331 = case shown="\"Active\", \"Show\", \"True\"" w557 {
          tunnel: [FALSE TRUE] -> w555
          frame "Disable", "False", Default {
          }
          frame "Active", "Show", "True" {
          }
        }
        n332 = Current VI's Menubar() -> (w556:refnum<k9>)
        n333 = call "RunTimeMenu_Save_State_TCE.vi"("enabled"=w555, "item tag"=string[] ["OVERLAY_GRID", "OVERLAY_CLEAR"], "Menu in"=w556) -> ()  [unwired: 8 in, 1 out]
        n334 = call <vilib>:"Add State(s) to Queue__JKI_lib_State_Machine.vi"("State(s) in (\"\")"=w561) -> ("States Out"=w560:string)  [unwired: 14 in]
      }
      frame "UI: Menu Overlay Temps" {
        # "Argument"
        # "Set and Unset Cursor Busy.\n(Usage: \"UI: Cursor Set >> Busy|Idle\")"
        n335 = case shown="\"Active\", \"Show\", \"True\"" w567 {
          tunnel: [FALSE TRUE] -> w565
          frame "Disable", "False", Default {
          }
          frame "Active", "Show", "True" {
          }
        }
        n336 = Current VI's Menubar() -> (w566:refnum<k9>)
        n337 = call "RunTimeMenu_Save_State_TCE.vi"("enabled"=w565, "item tag"=string[] ["OVERLAY_TEMPS", "OVERLAY_FREEZE"], "Menu in"=w566) -> ()  [unwired: 8 in, 1 out]
        n338 = call <vilib>:"Add State(s) to Queue__JKI_lib_State_Machine.vi"("State(s) in (\"\")"=w571) -> ("States Out"=w570:string)  [unwired: 14 in]
      }
      frame "UI: Single Temps" {
        # "Argument"
        # "Set and Unset Cursor Busy.\n(Usage: \"UI: Cursor Set >> Busy|Idle\")"
        n339 = control-ref of="Splitter 4"() -> (w574:refnum<vi>)
        n340 = case shown="\"Active\", \"Show\", \"True\"" w577 {
          tunnel: [w582 w585] -> w575
          tunnel: w574 -> [w583 w584]
          frame "Disable", "False", Default {
            w582 = FALSE
            n341 = call "ShowHideSplit.vi"("Splitter in"=w583, "Show Split"=w582) -> ()  [unwired: 1 in]
          }
          frame "Active", "Show", "True" {
            w585 = TRUE
            n342 = call "ShowHideSplit.vi"("Splitter in"=w584, "Show Split"=w585) -> ()  [unwired: 1 in]
          }
        }
        n343 = property on="Temps single grad" class="WFGraph (strict)"("Visible"=w575) -> ()  [unwired: 2 in, 2 out]
        n344 = property on="Temps single" class="WFGraph (strict)"("Visible"=w575) -> ()  [unwired: 2 in, 2 out]
        n345 = Not(x=w575) -> (.not. x?=w576:bool)
        n346 = property on="Temps grads" class="WFGraph (strict)"("Visible"=w576) -> ()  [unwired: 2 in, 2 out]
        n347 = property on="Temps" class="WFGraph (strict)"("Visible"=w576) -> ()  [unwired: 2 in, 2 out]
        n348 = property on="CurTemp" class="DigNum (strict)"("Visible"=w575) -> ()  [unwired: 2 in, 2 out]
        n349 = property on="Contents" class="Str"("Visible"=w575) -> ()  [unwired: 2 in, 2 out]
        n350 = property on="Well" class="Str"("Visible"=w575) -> ()  [unwired: 2 in, 2 out]
        n351 = call <vilib>:"Add State(s) to Queue__JKI_lib_State_Machine.vi"("State(s) in (\"\")"=w581) -> ("States Out"=w580:string)  [unwired: 14 in]
      }
      frame "UI: Front Panel State" {
        # "Argument"
        # "Set Front Panel Open or Closed\n(Usage: \"UI: Front Panel State >> Open|Close\")"
        n352 = Unbundle By Name(w588) -> ("Core.Current VI Reference"=w587:refnum<vi>)
        n353 = case shown="\"Minimize\", \"Minimized\"" w586 {
          tunnel: w590 -> [w598 w613 w624 w637 w650]
          tunnel: [w600 w614 w626 w639 w652] -> w589
          tunnel: w587 -> [w599 w611 w625 w638 w651]
          frame "Open", "Standard", Default {
            w593 = T3."Standard" ("State")
            n354 = property class="VI"(reference=w599, error in=w598) -> (reference out=w596:refnum<vi>, error out=w597:errorcluster, "FP.State"=w595:T3)
            n355 = Not Equal?(x=w595, y=w593) -> (x != y?=w594:bool)
            n356 = case shown="True" w594 {
              tunnel: [w604 w606] -> w600
              tunnel: w597 -> [w603 w606]
              tunnel: w596 -> [w602 _]
              tunnel: w593 -> [w601 _]
              frame True {
                n357 = invoke class="VI" method="FP.Open"(reference=w602, error in=w603, "Activate"=TRUE, "State"=w601) -> (error out=w604:errorcluster)  [unwired: 1 in, 4 out]
              }
              frame False {
              }
            }
          }
          frame "Close", "Closed" {
            n358 = property class="VI"(reference=w611, error in=w613) -> (reference out=w610:refnum<vi>, error out=w612:errorcluster, "FP.State"=w608:T3)
            n359 = Not Equal?(x=w608, y=T3."Closed" ("Front Panel Window:State")) -> (x != y?=w607:bool)
            n360 = case shown="True" w607 {
              tunnel: [w615 w618] -> w614
              tunnel: w612 -> [w615 w617]
              tunnel: w610 -> [_ w616]
              frame False {
              }
              frame True {
                n361 = invoke class="VI" method="FP.Close"(reference=w616, error in=w617) -> (error out=w618:errorcluster)  [unwired: 1 in, 2 out]
              }
            }
          }
          frame "Hidden", "Hide" {
            w619 = T3."Hidden" ("State")
            n362 = property class="VI"(reference=w625, error in=w624) -> (reference out=w622:refnum<vi>, error out=w623:errorcluster, "FP.State"=w621:T3)
            n363 = Not Equal?(x=w621, y=w619) -> (x != y?=w620:bool)
            n364 = case shown="True" w620 {
              tunnel: [w630 w631] -> w626
              tunnel: w623 -> [w629 w631]
              tunnel: w622 -> [w628 _]
              tunnel: w619 -> [w627 _]
              frame True {
                n365 = invoke class="VI" method="FP.Open"(reference=w628, error in=w629, "State"=w627) -> (error out=w630:errorcluster)  [unwired: 2 in, 4 out]
              }
              frame False {
              }
            }
          }
          frame "Minimize", "Minimized" {
            w632 = T3."Minimized" ("State")
            n366 = property class="VI"(reference=w638, error in=w637) -> (reference out=w635:refnum<vi>, error out=w636:errorcluster, "FP.State"=w634:T3)
            n367 = Not Equal?(x=w634, y=w632) -> (x != y?=w633:bool)
            n368 = case shown="True" w633 {
              tunnel: [w643 w644] -> w639
              tunnel: w636 -> [w642 w644]
              tunnel: w635 -> [w641 _]
              tunnel: w632 -> [w640 _]
              frame True {
                n369 = invoke class="VI" method="FP.Open"(reference=w641, error in=w642, "State"=w640) -> (error out=w643:errorcluster)  [unwired: 2 in, 4 out]
              }
              frame False {
              }
            }
          }
          frame "Maximize", "Maximized" {
            w645 = T3."Maximized" ("State")
            n370 = property class="VI"(reference=w651, error in=w650) -> (reference out=w648:refnum<vi>, error out=w649:errorcluster, "FP.State"=w647:T3)
            n371 = Not Equal?(x=w647, y=w645) -> (x != y?=w646:bool)
            n372 = case shown="True" w646 {
              tunnel: [w656 w657] -> w652
              tunnel: w649 -> [w655 w657]
              tunnel: w648 -> [w654 _]
              tunnel: w645 -> [w653 _]
              frame True {
                n373 = invoke class="VI" method="FP.Open"(reference=w654, error in=w655, "State"=w653) -> (error out=w656:errorcluster)  [unwired: 2 in, 4 out]
              }
              frame False {
              }
            }
          }
        }
        n374 = call <vilib>:"Add State(s) to Queue__JKI_lib_State_Machine.vi"("State(s) in (\"\")"=w592) -> ("States Out"=w591:string)  [unwired: 14 in]
      }
      frame "---------- Macro ----------" {
        # "Do not put any code in this frame.\n(It is a separator no-op. You can make a copy of this frame to create a new Macro frame)"
        n375 = call <vilib>:"Add State(s) to Queue__JKI_lib_State_Machine.vi"("State(s) in (\"\")"=w661) -> ("States Out"=w660:string)  [unwired: 14 in]
      }
      frame "Macro: Initialize" {
        w662 = "// UI: Cursor Set >> Busy\nData: Initialize\nInitialize Core Data\nUI: Initialize\nUI: Front Panel State >> Show\nUI: Tutorial >> Load Image\n// Image: Draw\n// UI: Cursor Set >> Idle"  # // UI: Cursor Set >> Busy Data: Initialize Initialize Core Data UI: Initialize UI: Front Panel State >> Show UI: Tutorial >> Load Image // Image: Draw // UI: Cursor Set >> Idle
        # "Initialization Macro\n(This is called once, when the VI starts)"
        n376 = call <vilib>:"Add State(s) to Queue__JKI_lib_State_Machine.vi"("State(s) in Front (\"\")"=w662, "State(s) in (\"\")"=w666) -> ("States Out"=w665:string)  [unwired: 13 in]
      }
      frame "Macro: Exit" {
        # "Exit Macro\n(This is called once, when the VI exits)"
        n377 = Unbundle By Name(w673) -> ("Core.Close Panel on Exit?"=w672:bool)
        n378 = Select(t="UI: Front Panel State >> Close", s=w672, f="") -> (s? t:f=w669:string)
        n379 = call <vilib>:"Add State(s) to Queue__JKI_lib_State_Machine.vi"("State(s) in (\"\")"=w669, "State(s) at Back (\"\")"="Data: Cleanup\nExit") -> ("States Out"=w667:string)  [unwired: 13 in]
        n380 = call <vilib>:"Add State(s) to Queue__JKI_lib_State_Machine.vi"("State(s) in Front (\"\")"=w667, "State(s) in (\"\")"=w676) -> ("States Out"=w675:string)  [unwired: 13 in]
      }
      frame "---------- Image ----------" {
        # "Template Separator\n(You can make a copy of, or modify, this frame)"
        n381 = call <vilib>:"Add State(s) to Queue__JKI_lib_State_Machine.vi"("State(s) in (\"\")"=w680) -> ("States Out"=w679:string)  [unwired: 14 in]
      }
      frame "Image: Draw" {
        # "Template Separator\n(You can make a copy of, or modify, this frame)"
        n382 = call <vilib>:"Add State(s) to Queue__JKI_lib_State_Machine.vi"("State(s) in Front (\"\")"="UI: Cursor Set >> Busy\nImage: Clear ROI\nImage: Calculate BR\nImage: Calculate y space\nImage: Calculate x space\nImage: Calculate Positions\nImage: Drawlines\nImage: Draw Points\nUI: Cursor Set >> Idle" ("State(s) in Front (\"\")"), "State(s) in (\"\")"=w685) -> ("States Out"=w684:string)  [unwired: 13 in]
      }
      frame "Image: Redraw" {
        # "Template Separator\n(You can make a copy of, or modify, this frame)"
        n383 = call <vilib>:"Add State(s) to Queue__JKI_lib_State_Machine.vi"("State(s) in Front (\"\")"="UI: Cursor Set >> Busy\nImage: Clear ROI\nImage: Drawlines\nImage: Draw Points\nImage: Calculate Temps\nUI: Cursor Set >> Idle" ("State(s) in Front (\"\")"), "State(s) in (\"\")"=w690) -> ("States Out"=w689:string)  [unwired: 13 in]
      }
      frame "Image: Drawlines" {
        # "Template Separator\n(You can make a copy of, or modify, this frame)"
        n384 = Unbundle By Name(w691) -> ("Points.Top Left.X"=w707:sgl, "Points.Top Right.X"=w706:sgl, "Points.Bottom Left.X"=w705:sgl, "Points.Bottom Right.X"=w704:sgl)
        n385 = Equal To 0?(x=w707) -> (x = 0?=w703:bool)
        n386 = Equal To 0?(x=w706) -> (x = 0?=w702:bool)
        n387 = Equal To 0?(x=w705) -> (x = 0?=w693:bool)
        n388 = Equal To 0?(x=w704) -> (x = 0?=w694:bool)
        n389 = Or(x=w693, y=w694) -> (x .or. y?=w692:bool)
        n390 = Select(t="", s=w693, f="Image: Draw Line >> TL_BL\n") -> (s? t:f=w699:string)
        n391 = Select(t="", s=w692, f="Image: Draw Line >> TR_BR\nImage: Draw Line >> BL_BR\nImage: Draw Line >> Vertical\nImage: Draw Line >> Horizontal") -> (s? t:f=w696:string)
        n392 = case shown="False" w703 {
          tunnel: w702 -> [w714 _]
          tunnel: w699 -> [w713 _]
          tunnel: w696 -> [w712 _]
          tunnel: [w711 _] -> w695
          frame False {
            n393 = case shown="False" w714 {
              tunnel: w713 -> [w717 _]
              tunnel: w712 -> [w716 _]
              tunnel: [w715 _] -> w711
              frame False {
                n394 = Concatenate Strings("Image: Draw Line >> TL_TR\n", w717, w716) -> (w715:string)
              }
              frame True {
              }
            }
          }
          frame True {
          }
        }
        n395 = call <vilib>:"Add State(s) to Queue__JKI_lib_State_Machine.vi"("State(s) in Front (\"\")"=w695, "State(s) in (\"\")"=w710) -> ("States Out"=w709:string)  [unwired: 13 in]
      }
      frame "Image: Clear ROI" {
        # "Your code here.\n(You can make a copy of, or modify, this frame)"
        n396 = Unbundle By Name(w722) -> ("Image Out"=w721:T1)
        n397 = call "IMAQ Clear Overlay"("error in (no error)"=w720, "Image"=w721) -> ("error out"=w719:errorcluster)  [unwired: 8 in, 1 out]
        n398 = call <vilib>:"Add State(s) to Queue__JKI_lib_State_Machine.vi"("State(s) in (\"\")"=w724) -> ("States Out"=w723:string)  [unwired: 14 in]
      }
      frame "Image: Calculate x space" {
        # "Your code here.\n(You can make a copy of, or modify, this frame)"
        n399 = Unbundle By Name(w733) -> ("Points.Top Left"=w739:T2, "Points.Top Right"=w738:T2, "PCR Size"=w725:u16)
        n400 = case shown="0, Default" w725 {
          tunnel: [24 12] -> w726
          frame 0, Default {
          }
          frame 1 {
          }
        }
        n401 = Unbundle(w739) -> ("X"=w736:sgl, "Y"=w734:sgl)
        n402 = Unbundle(w738) -> ("X"=w737:sgl, "Y"=w735:sgl)
        n403 = Decrement(x=w726) -> (x-1=w729:i32)
        n404 = Subtract(x=w737, y=w736) -> (x-y=w730:sgl)
        n405 = Divide(x=w730, y=w729) -> (x/y=w731:sgl)
        n406 = Subtract(x=w735, y=w734) -> (x-y=w728:sgl)
        n407 = Divide(x=w728, y=w729) -> (x/y=w727:sgl)
        n408 = Bundle By Name(cluster=w733, "Points.x_space"=w731, "Points.y_space"=w727) -> (w732:T6)
        n409 = call <vilib>:"Add State(s) to Queue__JKI_lib_State_Machine.vi"("State(s) in (\"\")"=w742) -> ("States Out"=w741:string)  [unwired: 14 in]
      }
      frame "Image: Calculate BR" {
        # "Your code here.\n(You can make a copy of, or modify, this frame)"
        n410 = Unbundle By Name(w753) -> ("Points.Top Left"=w759:T2, "Points.Top Right"=w758:T2, "Points.Bottom Left"=w751:T2)
        n411 = Unbundle(w759) -> ("X"=w756:sgl, "Y"=w754:sgl)
        n412 = Unbundle(w751) -> ("X"=w750:sgl, "Y"=w748:sgl)
        n413 = Unbundle(w758) -> ("X"=w757:sgl, "Y"=w755:sgl)
        n414 = Subtract(x=w757, y=w756) -> (x-y=w749:sgl)
        n415 = Add(x=w750, y=w749) -> (x+y=w745:sgl)
        n416 = Subtract(x=w755, y=w754) -> (x-y=w747:sgl)
        n417 = Add(x=w747, y=w748) -> (x+y=w746:sgl)
        n418 = Bundle By Name(cluster=w753, "Points.Bottom Right.X"=w745, "Points.Bottom Right.Y"=w746) -> (w752:T6)
        n419 = call <vilib>:"Add State(s) to Queue__JKI_lib_State_Machine.vi"("State(s) in (\"\")"=w762) -> ("States Out"=w761:string)  [unwired: 14 in]
      }
      frame "Image: Calculate y space" {
        # "Your code here.\n(You can make a copy of, or modify, this frame)"
        n420 = Unbundle By Name(w771) -> ("Points.Top Left"=w777:T2, "Points.Bottom Left"=w776:T2, "PCR Size"=w763:u16)
        n421 = case shown="1" w763 {
          tunnel: [16 8] -> w764
          frame 0, Default {
          }
          frame 1 {
          }
        }
        n422 = Unbundle(w777) -> ("X"=w774:sgl, "Y"=w772:sgl)
        n423 = Unbundle(w776) -> ("X"=w775:sgl, "Y"=w773:sgl)
        n424 = Decrement(x=w764) -> (x-1=w767:i32)
        n425 = Subtract(x=w775, y=w774) -> (x-y=w768:sgl)
        n426 = Divide(x=w768, y=w767) -> (x/y=w769:sgl)
        n427 = Subtract(x=w773, y=w772) -> (x-y=w766:sgl)
        n428 = Divide(x=w766, y=w767) -> (x/y=w765:sgl)
        n429 = Bundle By Name(cluster=w771, "Points.x space 2"=w769, "Points.y space 2"=w765) -> (w770:T6)
        n430 = call <vilib>:"Add State(s) to Queue__JKI_lib_State_Machine.vi"("State(s) in (\"\")"=w780) -> ("States Out"=w779:string)  [unwired: 14 in]
      }
      frame "Image: Set ROI" {
        # "Your code here.\n(You can make a copy of, or modify, this frame)"
        n431 = Unbundle By Name(w786) -> ("State"=w788:i32)
        n432 = case shown="0, Default" w788 {
          tunnel: [w792 w795 w797 w799] -> w787
          tunnel: w786 -> [w793 w794 w796 w798]
          frame 0, Default {
            n433 = Unbundle By Name(w793) -> ("Points.Top Left"=w792:T2)
          }
          frame 1 {
            n434 = Unbundle By Name(w794) -> ("Points.Top Right"=w795:T2)
          }
          frame 2 {
            n435 = Unbundle By Name(w796) -> ("Points.Bottom Left"=w797:T2)
          }
          frame 3 {
            n436 = Unbundle By Name(w798) -> ("Points.Bottom Right"=w799:T2)
          }
        }
        n437 = call "IMAQ Convert Point to ROI"("error in (no error)"=w785, "Point"=w787) -> ("error out"=w784:errorcluster, "ROI Descriptor"=w789:T9)  [unwired: 7 in]
        n438 = property on="Image" class="ImageControl"(error in=w784, "ROI"=w789) -> (error out=w783:errorcluster)  [unwired: 1 in, 1 out]
        n439 = call <vilib>:"Add State(s) to Queue__JKI_lib_State_Machine.vi"("State(s) in (\"\")"=w791) -> ("States Out"=w790:string)  [unwired: 14 in]
      }
      frame "Image: Draw Line" {
        w800 = u32 2  # Width
        # "Your code here.\n(You can make a copy of, or modify, this frame)"
        n440 = Unbundle By Name(w804) -> ("Image Out"=w805:T1)
        n441 = case shown="\"Vertical\"" w806 {
          tunnel: w805 -> [w810 w818 w827 w834 w840 w845 w854]
          tunnel: w804 -> [_ w819 w828 w829 w835 w849 w858]
          tunnel: [w810 w813 w826 w833 w839 w841 w850] -> w803
          tunnel: w802 -> [w809 w817 w825 w832 w838 w843 w853]
          tunnel: [w809 w812 w824 w831 w837 w842 w852] -> w801
          tunnel: w800 -> [_ w811 w820 _ _ w844 w851]
          frame "False", Default {
          }
          frame "TL_TR" {
            n442 = Unbundle By Name(w819) -> ("Points.Top Left"=w816:T2, "Points.Top Right"=w815:T2)
            n443 = Build Array(w816, w815) -> (w814:T2[])
            n444 = call "IMAQ Overlay Multiple Lines 2"("Image"=w818, "Line End Points"=w814, "error in (no error)"=w817, "Width"=w811) -> ("Image Out"=w813:T1, "error out"=w812:errorcluster)  [unwired: 10 in]
          }
          frame "TL_BL" {
            n445 = Unbundle By Name(w828) -> ("Points.Top Left"=w823:T2, "Points.Bottom Left"=w822:T2)
            n446 = Build Array(w823, w822) -> (w821:T2[])
            n447 = call "IMAQ Overlay Multiple Lines 2"("Image"=w827, "Line End Points"=w821, "error in (no error)"=w825, "Width"=w820) -> ("Image Out"=w826:T1, "error out"=w824:errorcluster)  [unwired: 10 in]
          }
          frame "Vertical" {
            n448 = call "TCam_VerticalLines.vi"("Width"=u32 1, "error in (no error)"=w832, "Cluster"=w829, "Refnum in"=w834) -> ("error out"=w831:errorcluster, "Refnum out"=w833:T1)  [unwired: 6 in]
          }
          frame "Horizontal" {
            n449 = call "TCam_HorizontalLines.vi"("Width"=u32 1, "error in (no error)"=w838, "Cluster"=w835, "Refnum in"=w840) -> ("error out"=w837:errorcluster, "Refnum out"=w839:T1)  [unwired: 6 in]
          }
          frame "TR_BR" {
            n450 = Unbundle By Name(w849) -> ("Points.Top Right"=w848:T2, "Points.Bottom Right"=w847:T2)
            n451 = Build Array(w848, w847) -> (w846:T2[])
            n452 = call "IMAQ Overlay Multiple Lines 2"("Image"=w845, "Line End Points"=w846, "error in (no error)"=w843, "Width"=w844) -> ("Image Out"=w841:T1, "error out"=w842:errorcluster)  [unwired: 10 in]
          }
          frame "BL_BR" {
            n453 = Unbundle By Name(w858) -> ("Points.Bottom Left"=w857:T2, "Points.Bottom Right"=w856:T2)
            n454 = Build Array(w857, w856) -> (w855:T2[])
            n455 = call "IMAQ Overlay Multiple Lines 2"("Image"=w854, "Line End Points"=w855, "error in (no error)"=w853, "Width"=w851) -> ("Image Out"=w850:T1, "error out"=w852:errorcluster)  [unwired: 10 in]
          }
        }
        n456 = local write "Image"(w803) -> ()
        n457 = call <vilib>:"Add State(s) to Queue__JKI_lib_State_Machine.vi"("State(s) in (\"\")"=w808) -> ("States Out"=w807:string)  [unwired: 14 in]
      }
      frame "Image: Draw Points" {
        # "Your code here.\n(You can make a copy of, or modify, this frame)"
        n458 = Unbundle By Name(w861) -> ("Points.Top Left.X"=w870:sgl, "Points.Top Right.X"=w869:sgl, "Points.Bottom Left.X"=w868:sgl, "Points.Bottom Right.X"=w867:sgl)
        n459 = Equal To 0?(x=w870) -> (x = 0?=w866:bool)
        n460 = Equal To 0?(x=w869) -> (x = 0?=w865:bool)
        n461 = Equal To 0?(x=w868) -> (x = 0?=w864:bool)
        n462 = Equal To 0?(x=w867) -> (x = 0?=w863:bool)
        n463 = Unbundle By Name(w861) -> ("Image Out"=w872:T1, "Scan Area"=w859:dbl)
        n464 = Compound Arithmetic op=OR(w866, w865, w864, w863) -> (w862:bool)
        n465 = case shown="False" w862 {
          tunnel: w872 -> [w881 _]
          tunnel: w861 -> [w878 w882]
          tunnel: [w876 w882] -> w860
          tunnel: w859 -> [w875 _]
          frame False {
            n466 = local read "Points"() -> (w880:T2[])
            n467 = call "TCam_CenterArray.vi"("Size"=w875, "Point Array"=w880, "Image in"=w881) -> ("Array"=w877:cluster{"X":i32, "Y":i32}[][], "Image"=w879:T1)  [unwired: 3 in]
            n468 = local write "Image"(w879) -> ()
            n469 = Bundle By Name(cluster=w878, "Points.Pixels"=w877) -> (w876:T6)
          }
          frame True {
          }
        }
        n470 = call <vilib>:"Add State(s) to Queue__JKI_lib_State_Machine.vi"("State(s) in (\"\")"=w874) -> ("States Out"=w873:string)  [unwired: 14 in]
      }
      frame "Image: Calculate Positions" {
        # "Your code here.\n(You can make a copy of, or modify, this frame)"
        n471 = Unbundle By Name(w885) -> ("Scan Area"=w883:dbl, "Points.Top Left.X"=w893:sgl, "Points.Top Right.X"=w892:sgl, "Points.Bottom Left.X"=w891:sgl, "Points.Bottom Right.X"=w890:sgl)
        n472 = Equal To 0?(x=w893) -> (x = 0?=w889:bool)
        n473 = Equal To 0?(x=w892) -> (x = 0?=w888:bool)
        n474 = Equal To 0?(x=w891) -> (x = 0?=w887:bool)
        n475 = Equal To 0?(x=w890) -> (x = 0?=w886:bool)
        n476 = Compound Arithmetic op=OR(w889, w888, w887, w886) -> (w884:bool)
        n477 = case shown="False" w884 {
          tunnel: w885 -> [w898 _]
          tunnel: w883 -> [w897 _]
          frame False {
            n478 = call "TCam_PointCalculator.vi"("Cluster"=w898, "Size"=w897) -> ("Points"=→"Points":T2[])  [unwired: 9 in]
          }
          frame True {
          }
        }
        n479 = call <vilib>:"Add State(s) to Queue__JKI_lib_State_Machine.vi"("State(s) in (\"\")"=w896) -> ("States Out"=w895:string)  [unwired: 14 in]
      }
      frame "Image: Calculate Temps" {
        # "Your code here.\n(You can make a copy of, or modify, this frame)"
        n480 = Unbundle By Name(w905) -> ("Image Out"=w903:T1, "Points.Pixels"=w902:cluster{"X":i32, "Y":i32}[][], "Points.Top Left.X"=w913:sgl, "Points.Top Right.X"=w912:sgl, "Points.Bottom Left.X"=w911:sgl, "Points.Bottom Right.X"=w910:sgl)
        n481 = Equal To 0?(x=w913) -> (x = 0?=w909:bool)
        n482 = Equal To 0?(x=w912) -> (x = 0?=w908:bool)
        n483 = Equal To 0?(x=w911) -> (x = 0?=w907:bool)
        n484 = Equal To 0?(x=w910) -> (x = 0?=w906:bool)
        n485 = local read "Points"() -> (w901:T2[])
        n486 = Compound Arithmetic op=OR(w909, w908, w907, w906) -> (w904:bool)
        n487 = case shown="False" w904 {
          tunnel: w903 -> [w919 w920]
          tunnel: w902 -> [w918 _]
          tunnel: w901 -> [_ _]
          tunnel: [w917 w920] -> w900
          frame False {
            n488 = call "TCam_WellTemp.vi"("Pixels"=w918, "Image in"=w919) -> ("Image Out"=w917:T1)  [unwired: 7 in, 2 out]
          }
          frame True {
          }
        }
        n489 = local write "Image"(w900) -> ()
        n490 = call <vilib>:"Add State(s) to Queue__JKI_lib_State_Machine.vi"("State(s) in (\"\")"=w916) -> ("States Out"=w915:string)  [unwired: 14 in]
      }
      frame "Image: Calculate Well" {
        # "Your code here.\n(You can make a copy of, or modify, this frame)"
        n491 = Unbundle By Name(w922) -> ("Image Out"=w927:T1, "Points.Pixels"=w926:cluster{"X":i32, "Y":i32}[][], "Points.Top Left.X"=w935:sgl, "Points.Top Right.X"=w934:sgl, "Points.Bottom Left.X"=w933:sgl, "Points.Bottom Right.X"=w932:sgl)
        n492 = local read "Points"() -> (w925:T2[])
        n493 = Equal To 0?(x=w935) -> (x = 0?=w931:bool)
        n494 = Equal To 0?(x=w934) -> (x = 0?=w930:bool)
        n495 = Equal To 0?(x=w933) -> (x = 0?=w929:bool)
        n496 = Equal To 0?(x=w932) -> (x = 0?=w928:bool)
        n497 = Compound Arithmetic op=OR(w931, w930, w929, w928) -> (w924:bool)
        n498 = case shown="False" w924 {
          tunnel: w927 -> [w960 _]
          tunnel: w926 -> [w959 _]
          tunnel: w925 -> [w958 _]
          tunnel: [w953 _] -> w923
          tunnel: w922 -> [w946 _]
          tunnel: w922 -> [w944 w965]
          tunnel: [w943 w965] -> w921
          frame False {
            n499 = local read "ImageIdx"() -> (w940:u32)
            n500 = property on="ImageIdx" class="Slide (strict)"() -> ("Scale.Maximum"=w948:dbl)  [unwired: 2 in, 2 out]
            n501 = call "TCam_WellCalculater.vi"("DrawTempOverlay"=TRUE, "Well Pos"=w958, "Pixels"=w959, "Image in"=w960, "index"="Well") -> ("Image Out"=w957:T1, "mean"=w942:dbl)  [unwired: 5 in]
            n502 = Increment(x=w940) -> (x+1=w954:u32)
            n503 = local write "Image"(w957) -> ()
            n504 = Greater?(x=w954, y=w948) -> (0:w956:bool)
            n505 = Unbundle By Name(w946) -> ("Temps"=w945:dbl[])
            n506 = case shown="False" w956 {
              tunnel: w954 -> [_ w964]
              tunnel: [w963 w964] -> w955
              tunnel: w954 -> [w963 _]
              tunnel: ["Data: Set Image\nImage: Calculate Well" ("State(s) in Front (\"\")") _] -> w953
              tunnel: [TRUE _] -> w952
              frame False {
              }
              frame True {
              }
            }
            n507 = Divide(x=w940, y=w948) -> (x/y=w951:dbl)
            n508 = property on="Temps single" class="WFGraph (strict)"("Cursor.Cursor X"=w940) -> ()  [unwired: 2 in, 2 out]
            n509 = Multiply(x=w951, y=100.0) -> (x*y=w949:dbl)
            n510 = Build Array (concatenate)(w945, w942) -> (w941:dbl[])
            "Temps single" <- w941
            n511 = local write "Slide"(w949) -> ()
            n512 = Bundle By Name(cluster=w944, "Temps"=w941) -> (w943:T6)
            n513 = local write "ImageIdx"(w955) -> ()
            n514 = property on="Slide" class="Slide (strict)"("Visible"=w952) -> ()  [unwired: 2 in, 2 out]
          }
          frame True {
          }
        }
        n515 = call <vilib>:"Add State(s) to Queue__JKI_lib_State_Machine.vi"("State(s) in Front (\"\")"=w923, "State(s) in (\"\")"=w938) -> ("States Out"=w937:string)  [unwired: 13 in]
      }
      frame "Image: Calculate All Temps" {
        # "Your code here.\n(You can make a copy of, or modify, this frame)"
        n516 = Unbundle By Name(w968) -> ("img_array"=w971:T1[], "Points.Pixels"=w970:cluster{"X":i32, "Y":i32}[][], "Points.Top Left.X"=w979:sgl, "Points.Top Right.X"=w978:sgl, "Points.Bottom Left.X"=w977:sgl, "Points.Bottom Right.X"=w976:sgl)
        n517 = Equal To 0?(x=w979) -> (x = 0?=w975:bool)
        n518 = Equal To 0?(x=w978) -> (x = 0?=w974:bool)
        n519 = Equal To 0?(x=w977) -> (x = 0?=w973:bool)
        n520 = Equal To 0?(x=w976) -> (x = 0?=w972:bool)
        n521 = Compound Arithmetic op=OR(w975, w974, w973, w972) -> (w969:bool)
        n522 = case shown="False" w969 {
          tunnel: w971 -> [w985 _]
          tunnel: w970 -> [w987 _]
          tunnel: [TRUE ("Visible") FALSE ("Visible")] -> w966
          tunnel: [w983 dbl[][] []] -> w967
          frame False {
            n523 = for {
              N -> [w990]
              tunnel: w985 -> [w1001] mode=indexing
              tunnel: w987 -> [w1000]
              tunnel: [w999] -> w986 mode=indexing
              workers-P: _ -> [_]
              i -> [w988]
              n524 = call "TCam_WellTemp.vi"("Pixels"=w1000, "Image in"=w1001) -> ("Temps"=w999:dbl[])  [unwired: 7 in, 2 out]
              n525 = property on="ImageIdx" class="Slide (strict)"() -> ("Scale.Maximum"=w996:dbl)  [unwired: 2 in, 2 out]
              n526 = local read "img"() -> (w998:i32)
              n527 = property on="Temps" class="WFGraph (strict)"("Cursor.Cursor X"=w988) -> ()  [unwired: 2 in, 2 out]
              n528 = Increment(x=w998) -> (x+1=w989:i32)
              n529 = Divide(x=w989, y=w996) -> (x/y=w1003:dbl)
              n530 = local write "img"(w989) -> ()
              n531 = Format Into String(w989) -> (resulting string=w995:string)  [unwired: 3 in, 1 out]
              n532 = Multiply(x=w1003, y=100.0) -> (x*y=w997:dbl)
              n533 = property on="Temps grads" class="WFGraph (strict)"("Cursor.Cursor X"=w988) -> ()  [unwired: 2 in, 2 out]
              n534 = Format Into String(w990) -> (resulting string=w991:string)  [unwired: 3 in, 1 out]
              n535 = local write "Slide"(w997) -> ()
              n536 = Concatenate Strings("Processing image " ("Tutorial"), w995, " of " ("Tutorial"), w991) -> (w994:string)
              n537 = local write "Tutorial"(w994) -> ()
            }
            n538 = Transpose 2D Array(2D array=w986) -> (transposed array=w983:dbl[][])
          }
          frame True {
          }
        }
        "Temps" <- w967
        n539 = property on="Correct Data" class="Bool"("Visible"=w966) -> ()  [unwired: 2 in, 2 out]
        n540 = call <vilib>:"Add State(s) to Queue__JKI_lib_State_Machine.vi"("State(s) in (\"\")"=w982) -> ("States Out"=w981:string)  [unwired: 14 in]
      }
      frame "Image: Calculate Gradients" {
        # "Your code here.\n(You can make a copy of, or modify, this frame)"
        n541 = local read "Temps"() -> (w1007:dbl[][])
        n542 = for {
          tunnel: w1007 -> [w1016] mode=indexing
          workers-P: _ -> [_]
          tunnel: [w1012] -> w1006 mode=indexing
          n543 = Array Size(array=w1016) -> (size(s)=w1015:i32)
          n544 = Decrement(x=w1015) -> (x-1=w1014:i32)
          n545 = for {
            N: w1014 -> [_]
            tunnel: w1016 -> [w1024]
            shift-right: [w1018] -> w1012
            shift-left: dbl[] [0.0] -> [w1017]
            i -> [w1023]
            n546 = Increment(x=w1023) -> (x+1=w1022:i32)
            n547 = Index Array(array=w1024, index=w1023) -> (element=w1020:dbl)
            n548 = Index Array(array=w1024, index=w1022) -> (element=w1021:dbl)
            n549 = Subtract(x=w1021, y=w1020) -> (x-y=w1019:dbl)
            n550 = Build Array (concatenate)(w1017, w1019) -> (w1018:dbl[])
          }
        }
        "Temps grads" <- w1006
        n551 = call <vilib>:"Add State(s) to Queue__JKI_lib_State_Machine.vi"("State(s) in (\"\")"=w1011) -> ("States Out"=w1010:string)  [unwired: 14 in]
      }
      frame "Image: Calculate Freezing Points" {
        # "Your code here.\n(You can make a copy of, or modify, this frame)"
        n552 = local read "Temps grads"() -> (w1030:dbl[][])
        n553 = local read "Temps"() -> (w1029:dbl[][])
        n554 = for {
          tunnel: w1030 -> [w1037] mode=indexing
          workers-P: _ -> [_]
          tunnel: w1029 -> [w1047] mode=indexing
          tunnel: [w1041] -> w1028 mode=indexing
          tunnel: [w1039] -> w1027 mode=indexing
          tunnel: [w1035] -> w1026 mode=indexing
          # "Gradient Check"
          n555 = call <vilib>:"Std Deviation and Variance.vi"("X"=w1037) -> ("standard deviation"=w1036:dbl)  [unwired: 1 in, 2 out]
          n556 = Array Max & Min(array=w1037) -> (max value=w1045:dbl, max index (indices)=w1040:i32)  [unwired: 2 out]
          n557 = Multiply(x=5.0, y=w1036) -> (x*y=w1044:dbl)
          n558 = Array Subset(array=w1047, length=w1040) -> (w1046:dbl[])  [unwired: 1 in]
          n559 = Greater?(x=w1045, y=w1044) -> (0:w1042:bool)
          n560 = Array Max & Min(array=w1046) -> (min value=w1038:dbl)  [unwired: 3 out]
          n561 = case shown="True" w1042 {
            selector: w1042 -> [w1048 w1051]
            tunnel: [0 w1053] -> w1041
            tunnel: w1040 -> [_ w1053]
            tunnel: [0.0 w1052] -> w1039
            tunnel: w1038 -> [_ w1052]
            tunnel: [w1048 w1051] -> w1035
            frame False {
            }
            frame True {
            }
          }
        }
        "FreezeIdx" <- w1028
        "FreezeTemps" <- w1027
        "FreezeArray" <- w1026
        n562 = call <vilib>:"Add State(s) to Queue__JKI_lib_State_Machine.vi"("State(s) in Front (\"\")"="UI: Menu Save >> True\nUI: Menu Overlay Temps >> True" ("State(s) in Front (\"\")"), "State(s) in (\"\")"=w1034) -> ("States Out"=w1033:string)  [unwired: 13 in]
      }
      frame "Image: Overlay Freeze Temps" {
        # "Your code here.\n(You can make a copy of, or modify, this frame)"
        n563 = local read "FreezeTemps"() -> (w1057:dbl[])
        n564 = local read "FreezeArray"() -> (w1055:bool[])
        n565 = local read "FreezeIdx"() -> (w1056:i32[])
        n566 = local read "Points"() -> (w1058:T2[])
        n567 = Unbundle By Name(w1060) -> ("img_array"=w1059:T1[])
        n568 = call "OverlayFreezeRange.vi"("FreezeIdx"=w1056, "FreezeArray"=w1055) -> ("Range"=w1054:i32)
        n569 = for {
          N -> [w1064]
          tunnel: w1056 -> [w1079] mode=indexing
          tunnel: w1059 -> [w1080]
          tunnel: w1058 -> [w1078] mode=indexing
          tunnel: w1057 -> [w1077] mode=indexing
          tunnel: w1055 -> [w1076] mode=indexing
          tunnel: w1054 -> [w1075]
          n570 = local read "img"() -> (w1074:i32)
          n571 = case shown="True" w1076 {
            tunnel: w1080 -> [_ w1089]
            tunnel: w1079 -> [_ w1081]
            tunnel: w1078 -> [_ w1087]
            tunnel: w1077 -> [_ w1084]
            tunnel: w1075 -> [_ w1083]
            frame False {
            }
            frame True {
              n572 = Divide(x=w1081, y=w1083) -> (x/y=w1086:dbl)
              n573 = Array Subset(array=w1089, index=w1081) -> (w1088:T1[])  [unwired: 1 in]
              n574 = Multiply(x=w1086, y=30.0) -> (x*y=w1082:dbl)
              n575 = for {
                tunnel: w1088 -> [w1094] mode=indexing
                tunnel: w1087 -> [w1093]
                tunnel: w1084 -> [w1092]
                workers-P: _ -> [_]
                tunnel: w1082 -> [w1091]
                n576 = call "ColorRamp.vi"("Slide"=w1091) -> ("Color"=w1090:u32)
                n577 = Format Into String(format string="%3.2f", w1092) -> (resulting string=w1097:string)  [unwired: 2 in, 1 out]
                n578 = call "IMAQ Overlay Text"("BG Color (Transparent)"=w1090, "Font, Size & Style"=T8 {"Desired Font (Application)"=enum."Application Font", "[User-specified Font]"={"Font Name"="", "Size"=6, "Strikeout?"=FALSE, "Italic?"=FALSE, "Underline?"=FALSE, "Outline?"=FALSE, "Shadow?"=FALSE, "Bold?"=FALSE, "Rotation Angle"=0.0}, "Horizontal Alignment"=1, "Vertical Alignment"=0}, "String"=w1097, "Origin"=w1093, "Image"=w1094) -> ()  [unwired: 5 in, 2 out]
              }
            }
          }
          n579 = Increment(x=w1074) -> (x+1=w1068:i32)
          n580 = Divide(x=w1074, y=w1064) -> (x/y=w1069:dbl)
          n581 = local write "img"(w1068) -> ()
          n582 = Multiply(x=w1069, y=100.0) -> (x*y=w1070:dbl)
          n583 = local write "Slide"(w1070) -> ()
          n584 = Format Into String(initial string="Overlaying Well " ("Tutorial"), w1074) -> (resulting string=w1072:string)  [unwired: 2 in, 1 out]
          n585 = Format Into String(initial string=" of ", w1064) -> (resulting string=w1071:string)  [unwired: 2 in, 1 out]
          n586 = Concatenate Strings(w1072, w1071) -> (w1073:string)
          n587 = local write "Tutorial"(w1073) -> ()
        }
        n588 = call <vilib>:"Add State(s) to Queue__JKI_lib_State_Machine.vi"("State(s) in (\"\")"=w1063) -> ("States Out"=w1062:string)  [unwired: 14 in]
      }
      frame "Image: Overlay Freeze" {
        # "Your code here.\n(You can make a copy of, or modify, this frame)"
        n589 = local read "FreezeArray"() -> (w1099:bool[])
        n590 = local read "FreezeIdx"() -> (w1100:i32[])
        n591 = local read "Points"() -> (w1101:T2[])
        n592 = Unbundle By Name(w1103) -> ("img_array"=w1102:T1[])
        n593 = call "OverlayFreezeRange.vi"("FreezeIdx"=w1100, "FreezeArray"=w1099) -> ("Range"=w1098:i32)
        n594 = for {
          N -> [w1109]
          tunnel: w1100 -> [w1121] mode=indexing
          tunnel: w1102 -> [w1122]
          tunnel: w1101 -> [w1120] mode=indexing
          tunnel: w1099 -> [w1119] mode=indexing
          tunnel: w1098 -> [w1118]
          n595 = local read "img"() -> (w1110:i32)
          n596 = case shown="True" w1119 {
            tunnel: w1122 -> [_ w1130]
            tunnel: w1121 -> [_ w1123]
            tunnel: w1120 -> [_ w1128]
            tunnel: w1118 -> [_ w1125]
            frame False {
            }
            frame True {
              n597 = Divide(x=w1123, y=w1125) -> (x/y=w1127:dbl)
              n598 = Array Subset(array=w1130, index=w1123) -> (w1129:T1[])  [unwired: 1 in]
              n599 = Multiply(x=w1127, y=30.0) -> (x*y=w1124:dbl)
              n600 = for {
                tunnel: w1129 -> [w1136] mode=indexing
                tunnel: w1128 -> [w1135]
                workers-P: _ -> [_]
                tunnel: w1124 -> [w1134]
                n601 = call "ColorRamp.vi"("Slide"=w1134) -> ("Color"=w1133:u32)
                n602 = call "IMAQ Overlay Text"("BG Color (Transparent)"=w1133, "Font, Size & Style"=T8 {"Desired Font (Application)"=enum."Application Font", "[User-specified Font]"={"Font Name"="", "Size"=1, "Strikeout?"=FALSE, "Italic?"=FALSE, "Underline?"=FALSE, "Outline?"=FALSE, "Shadow?"=FALSE, "Bold?"=FALSE, "Rotation Angle"=0.0}, "Horizontal Alignment"=1, "Vertical Alignment"=0}, "String"="   ", "Origin"=w1135, "Image"=w1136) -> ()  [unwired: 5 in, 2 out]
              }
            }
          }
          n603 = Increment(x=w1110) -> (x+1=w1117:i32)
          n604 = Divide(x=w1110, y=w1109) -> (x/y=w1116:dbl)
          n605 = local write "img"(w1117) -> ()
          n606 = Multiply(x=w1116, y=100.0) -> (x*y=w1115:dbl)
          n607 = local write "Slide"(w1115) -> ()
          n608 = Format Into String(initial string="Overlaying Well " ("Tutorial"), w1110) -> (resulting string=w1112:string)  [unwired: 2 in, 1 out]
          n609 = Format Into String(initial string=" of ", w1109) -> (resulting string=w1113:string)  [unwired: 2 in, 1 out]
          n610 = Concatenate Strings(w1112, w1113) -> (w1111:string)
          n611 = local write "Tutorial"(w1111) -> ()
        }
        n612 = call <vilib>:"Add State(s) to Queue__JKI_lib_State_Machine.vi"("State(s) in (\"\")"=w1106) -> ("States Out"=w1105:string)  [unwired: 14 in]
      }
      frame "Image: Overlay Freeze Old" {
        # "Your code here.\n(You can make a copy of, or modify, this frame)"
        n613 = local read "FreezeArray"() -> (w1138:bool[])
        n614 = Unbundle By Name(w1141) -> ("img_array"=w1143:T1[])
        n615 = local read "FreezeIdx"() -> (w1139:i32[])
        n616 = Unbundle By Name(w1141) -> ("Points.Pixels"=w1140:cluster{"X":i32, "Y":i32}[][])
        n617 = local read "Points"() -> (w1142:T2[])
        n618 = call "OverlayFreezeRange.vi"("FreezeIdx"=w1139, "FreezeArray"=w1138) -> ("Range"=w1137:i32)
        n619 = for {
          N -> [w1149]
          tunnel: w1139 -> [w1164] mode=indexing
          tunnel: w1143 -> [w1167]
          tunnel: w1142 -> [w1165] mode=indexing
          workers-P: _ -> [_]
          tunnel: w1137 -> [w1162]
          tunnel: w1140 -> [w1161] mode=indexing
          tunnel: w1138 -> [w1147] mode=indexing
          n620 = local read "img"() -> (w1150:i32)
          n621 = Increment(x=w1150) -> (x+1=w1155:i32)
          n622 = Divide(x=w1164, y=w1162) -> (x/y=w1163:dbl)
          n623 = Array Subset(array=w1167, index=w1164) -> (w1166:T1[])  [unwired: 1 in]
          n624 = local write "img"(w1155) -> ()
          n625 = Multiply(x=w1163, y=30.0) -> (x*y=w1160:dbl)
          n626 = Divide(x=w1150, y=w1149) -> (x/y=w1158:dbl)
          n627 = case shown="True" w1147 {
            tunnel: w1166 -> [_ w1171]
            tunnel: w1165 -> [_ w1170]
            tunnel: w1161 -> [_ w1169]
            tunnel: w1160 -> [_ w1168]
            frame False {
            }
            frame True {
              n628 = for {
                tunnel: w1171 -> [w1172] mode=indexing
                tunnel: w1170 -> [w1176]
                tunnel: w1168 -> [w1174]
                tunnel: w1169 -> [w1175]
                n629 = call "ColorRamp.vi"("Slide"=w1174) -> ("Color"=w1173:u32)
                n630 = call "IMAQ Overlay Points"("Color"=w1173, "Array of Points"=w1175, "Point"=w1176, "Image"=w1172) -> ()  [unwired: 6 in, 2 out]
              }
            }
          }
          n631 = Multiply(x=w1158, y=100.0) -> (x*y=w1157:dbl)
          n632 = local write "Slide"(w1157) -> ()
          n633 = Format Into String(w1150) -> (resulting string=w1153:string)  [unwired: 3 in, 1 out]
          n634 = Format Into String(w1149) -> (resulting string=w1154:string)  [unwired: 3 in, 1 out]
          n635 = Concatenate Strings("Overlaying Well " ("Tutorial"), w1153, " of " ("Tutorial"), w1154) -> (w1152:string)
          n636 = local write "Tutorial"(w1152) -> ()
        }
        n637 = call <vilib>:"Add State(s) to Queue__JKI_lib_State_Machine.vi"("State(s) in (\"\")"=w1146) -> ("States Out"=w1145:string)  [unwired: 14 in]
      }
      frame "Image: Remove Overlays" {
        # "Your code here.\n(You can make a copy of, or modify, this frame)"
        n638 = Unbundle By Name(w1178) -> ("img_array"=w1177:T1[])
        n639 = for {
          tunnel: w1177 -> [w1182] mode=indexing
          n640 = call "IMAQ Clear Overlay"("Image"=w1182) -> ()  [unwired: 9 in, 2 out]
        }
        n641 = call <vilib>:"Add State(s) to Queue__JKI_lib_State_Machine.vi"("State(s) in (\"\")"=w1181) -> ("States Out"=w1180:string)  [unwired: 14 in]
      }
      frame "Image: Update Focus Well" {
        # "Your code here.\n(You can make a copy of, or modify, this frame)"
        n642 = local read "FreezeIdx"() -> (w1183:i32[])
        n643 = local read "Temps"() -> (w1191:dbl[][])
        n644 = local read "Temps grads"() -> (w1190:dbl[][])
        n645 = local read "PartitionArray"() -> (w1186:string[])
        n646 = local read "FreezeTemps"() -> (w1189:dbl[])
        n647 = call "PCRNameArray.vi"("input cluster"=w1185) -> ("WellArray"=w1184:string[])
        n648 = local read "Well"() -> (w1187:i32)
        n649 = Empty Array?(array=w1191) -> (empty?=w1188:bool)
        n650 = case shown="False" w1188 {
          tunnel: w1187 -> [w1196 _]
          tunnel: w1191 -> [w1208 _]
          tunnel: w1190 -> [w1207 _]
          tunnel: w1189 -> [w1206 _]
          tunnel: w1186 -> [w1203 _]
          tunnel: w1184 -> [w1201 _]
          tunnel: w1183 -> [w1197 _]
          frame False {
            n651 = Index Array(array=w1208, index (row)=w1196) -> (element=w1199:dbl[])  [unwired: 1 in]
            n652 = Index Array(array=w1206, index=w1196) -> (element=→"FreezeTemp":dbl)
            n653 = Index Array(array=w1207, index (row)=w1196) -> (element=→"Temps single grad":dbl[])  [unwired: 1 in]
            n654 = Index Array(array=w1203, index=w1196) -> (element=→"Contents":string)
            n655 = Index Array(array=w1201, index=w1196) -> (element=→"Well":string)
            n656 = Index Array(array=w1197, index=w1196) -> (element=w1195:i32)
            n657 = Index Array(array=w1199, index=w1195) -> (element=→"CurTemp":dbl)
            n658 = property on="Temps single" class="WFGraph (strict)"("Cursor.Cursor X"=w1195) -> ()  [unwired: 2 in, 2 out]
            n659 = property on="Temps single grad" class="WFGraph (strict)"("Cursor.Cursor X"=w1195) -> ()  [unwired: 2 in, 2 out]
            n660 = local write "ImageIdx"(w1195) -> ()
            n661 = local write "Temps single"(w1199) -> ()
          }
          frame True {
          }
        }
        n662 = call <vilib>:"Add State(s) to Queue__JKI_lib_State_Machine.vi"("State(s) in (\"\")"=w1194) -> ("States Out"=w1193:string)  [unwired: 14 in]
      }
      frame "Image: Correct Offset" {
        # "Your code here.\n(You can make a copy of, or modify, this frame)"
        n663 = local read "Temps"() -> (w1211:dbl[][])
        n664 = local read "Offsets"() -> (w1210:dbl[])
        n665 = for {
          tunnel: w1211 -> [w1218] mode=indexing
          tunnel: w1210 -> [w1217]
          tunnel: [w1216] -> w1209 mode=indexing
          n666 = Subtract(x=w1218, y=w1217) -> (x-y=w1216:dbl[])
        }
        n667 = local write "Temps"(w1209) -> ()
        n668 = call <vilib>:"Add State(s) to Queue__JKI_lib_State_Machine.vi"("State(s) in (\"\")"=w1215) -> ("States Out"=w1214:string)  [unwired: 14 in]
      }
      frame "Image: Remove Offset" {
        # "Your code here.\n(You can make a copy of, or modify, this frame)"
        n669 = local read "Temps"() -> (w1221:dbl[][])
        n670 = local read "Offsets"() -> (w1220:dbl[])
        n671 = for {
          tunnel: w1221 -> [w1228] mode=indexing
          tunnel: w1220 -> [w1227]
          tunnel: [w1226] -> w1219 mode=indexing
          n672 = Add(x=w1228, y=w1227) -> (x+y=w1226:dbl[])
        }
        n673 = local write "Temps"(w1219) -> ()
        n674 = call <vilib>:"Add State(s) to Queue__JKI_lib_State_Machine.vi"("State(s) in (\"\")"=w1225) -> ("States Out"=w1224:string)  [unwired: 14 in]
      }
      frame "Image: Calculate Offset" {
        # "Your code here.\n(You can make a copy of, or modify, this frame)"
        n675 = local read "ThermTemps"() -> (w1230:dbl[])
        n676 = call "TCam_FixpointTemps.vi"("input cluster"=w1231, "Therm_Temps"=w1230) -> ("Offsets"=→"Offsets":dbl[])  [unwired: 1 out]
        n677 = call <vilib>:"Add State(s) to Queue__JKI_lib_State_Machine.vi"("State(s) in (\"\")"=w1234) -> ("States Out"=w1233:string)  [unwired: 14 in]
      }
    }
  }
  n678 = property on="Remove_Correction" class="Bool"("Visible"=TRUE) -> ()  [unwired: 2 in, 2 out]
